vi "Text control 2 v6.8_pump-specific.vi"() -> ()   [LabVIEW 2016]
panel:
  in  "Tab Control":enum32{"Main", "Other parameters"}(tab)
  out "Line running":i32
  out "Total lines":i32
  out "Path":path=path "C:/users/rlp38/09Apr2009LTtesting/test2.txt"
  out "I vs Vg":cluster{"Y data in":dbl[], "X data in":dbl[]}[](graph)
  out "Is max":dbl format="%.2e"
  out "Id max":dbl format="%.2e"
  out "Ig max":dbl format="%.2e"
  out "Imax vs time":cluster{"Y data in":dbl[], "X data in":dbl[]}[](graph)
  out "Imin vs time":cluster{"Y data in":dbl[], "X data in":dbl[]}[](graph)
  out "I vs Vd":cluster{"Y data in":dbl[], "X data in":dbl[]}[](graph)
  in  "Script":string="#-------------------------------------------------------\n# SPM pump cleaning script\n#\n# Version: 0.5\n# Author: Dimitrios Simatos\n# Last updated: 2018-01-05\n#-------------------------------------------------------\n# Description\n#\n# This script is designed to run the cleaning sequence of the SPM OEM pump.\n# This script needs to be run 4 times!\n#-------------------------------------------------------\n# Changes\n#\n# Placed initialization and hard stop commands in the beginning.\n#-------------------------------------------------------\n# Important points\n#\n# Never leave any liquid in the pump to dry after the experiments. If they dry, the residue may block the valve.\n# Always run the cleaning cycle after the experiments.\n# Use clockwise rotation when going up in valve port numbers and vice versa.\n#-------------------------------------------------------\n# Things to do before running the script\n#\n# Set time units to minutes.\n# Set filenames.\n# Replace the tubing, if necessary.\n#-------------------------------------------------------\n# Port connections\n#\n# Port 1: Waste\n# Port 2: Waste\n# Port 3: Various cleaning liquids\n# Port 4: Waste\n# Port 5: Waste\n# Port 6: Waste\n#\n# Between each of the 4 runs, the settings of Port 3 will change, according to the cleaning protocol.\n# The settings for Port 3 are:\n# 1st run: 1% v/v solution of sodium hypochlorite in ultrapure water\n# 2nd run: 0.1% w/v solution of sodium dodecyl sulfate in ultrapure water\n# 3rd run: Ultrapure water\n# 4th run: Waste (in air, not immersed in liquid)\n#-------------------------------------------------------\n# Cleaning protocol for the SPM OEM pump (from the manual)\n#\n# A cleaning procedure should be performed at the end of each day or in between two different experiments.\n# An effective cleaning can be performed in the following manner:\n# • Bleach solution to kill microorganisms\n# 1. Prepare a solution of 1% chlorine bleach and deionized water\n#    NOTE: Prepare a 1% v/v solution of sodium hypochlorite in deionized water\n# 2. Prepare a reservoir and place 1 tubing in the bleach solution and 5 tubings in a waste recipient\n# 3. Pick up the bleach solution through 1 port to entirely fill the syringe\n# 4. Sequentially output the syringe content through the remaining ports and throw it to the waste\n# 5. Repeat operation at least 2 times\n# • Detergent solution to remove debris\n# 1. Prepare a solution of 0.1% detergent and deionized water\n#    NOTE: Prepare a 0.1% w/v solution of sodium dodecyl sulfate in deionized water\n# 2. Move the tubing from the bleach solution reservoir and place it into a reservoir of detergent solution\n# 3. Pick up the detergent solution through 1 port to entirely fill the syringe\n# 4. Sequentially output the detergent solution through the remaining ports into the waste recipient\n# 5. Repeat operation at least 2 times\n# • Rinsing water to prepare the pump for your next experiment\n# 1. Move the tubing from the detergent solution reservoir and place it into a reservoir of deionized water\n# 2. Pick up the rinsing solution through 1 port to entirely fill the syringe\n# 3. Sequentially output the rinse water through the remaining ports into the waste recipient\n# 4. Repeat operation at least 2 times\n# • Replace the tubing, if necessary\n#-------------------------------------------------------\n# Pumping cycles and execution time\n#\n# Execution time for a single cycle: 6 x (1 min + 10 sec) = 7 minutes\n# Total execution time: 4 x 7 = 28 minutes\n# Since the script has to run 4 times, the cleaning lasts for: 4 x 28 = 112 minutes\n# Air must be the last to be pumped through the valve, to remove all liquids.\n# There are 4 pumping cycles. Each one draws a different liquid through port 3 and pumps it sequentially through ports 1,2,4,5,6.\n# During the sequential pumping, each port receives 200 ml of liquid (20% of the total syringe volume = 600 \"plunger units\")\n# The device must be disconnected from the port during the cleaning procedure.\n# All cycles are similar, except cycle 1 has the initialization command uncommented and the first report valve command commented.\n#-------------------------------------------------------\n# Volume of liquid needed\n#\n# Volume of liquid needed per cycle: 1 ml\n# Total volume of liquid needed per script run: 4 x 1 = 4 ml\n# Since the script has to run 4 times, the first 3 with different liquids, I need:\n# 4 ml of 1% v/v solution of sodium hypochlorite in ultrapure water\n# 4 ml of 0.1% w/v solution of sodium dodecyl sulfate in ultrapure water\n# 4 ml of ultrapure water\n#-------------------------------------------------------\n# Parameters\n#\n# Syringe size: 1 ml\n# Step resolution N = 0.01 mm\n# Drawing flow V = 300 pulses/second (6000 ul/min)\n# Pumping flow V = 300 pulses/second (6000 ul/min)\n#-------------------------------------------------------\n# Pump initialization\npump /1T #hard stop pump\npump /1ZR #initialize pump\n#-------------------------------------------------------\n# Cycle 1\n# Fill the syringe\npump /1Q #query pump\npump /1? #report absolute plunger position\n#pump /1?6 #report valve position\nwait-min 1 #wait 1 minute\npump /1N0R #set step resolution: 0.01 mm\npump /1Q #query pump\npump /1? #report absolute plunger position (the plunger should be at 0)\npump /1?6 #report valve position\nwait 1000 #wait 1 second\npump /1V300R #choose speed: 300 steps/s (6000 ul/min)\npump /1Q #query pump\nwait 1000 #wait 1 second\npump /1I3R #go to port 3, clockwise rotation\npump /1Q #query pump\npump /1?6 #report valve position\nwait 1000 #wait 1 second\npump /1A3000R #go to absolute position 3000 (= draw 1 ml)\nwait 30000 #wait 30 seconds\npump /1Q #query pump\npump /1? #report absolute plunger position (the plunger should have finished moving)\n#pump /1?6 #report valve position\n# The sequential pumping begins\n# Port 1\npump /1O1R #switch to port 1, counterclockwise rotation\npump /1Q #query pump\npump /1?6 #report valve position\npump /1A2400R #go to absolute position 2400 (= pump 200 ul)\npump /1Q #query pump\npump /1? #report absolute plunger position (the plunger should be moving to 0)\nwait-min 1 #wait 1 minute\npump /1? #report absolute plunger position (the plunger should have finished moving)\n# Port 2\npump /1I2R #switch to port 2, clockwise rotation\npump /1Q #query pump\npump /1?6 #report valve position\npump /1A1800R #go to absolute position 1800 (= pump 200 ul)\npump /1Q #query pump\npump /1? #report absolute plunger position (the plunger should be moving to 0)\nwait-min 1 #wait 1 minute\npump /1? #report absolute plunger position (the plunger should have finished moving)\n# Port 4\npump /1I4R #switch to port 4, clockwise rotation\npump /1Q #query pump\npump /1?6 #report valve position\npump /1A1200R #go to absolute position 1200 (= pump 200 ul)\npump /1Q #query pump\npump /1? #report absolute plunger position (the plunger should be moving to 0)\nwait-min 1 #wait 1 minute\npump /1? #report absolute plunger position (the plunger should have finished moving)\n# Port 5\npump /1I5R #switch to port 5, clockwise rotation\npump /1Q #query pump\npump /1?6 #report valve position\npump /1A600R #go to absolute position 600 (= pump 200 ul)\npump /1Q #query pump\npump /1? #report absolute plunger position (the plunger should be moving to 0)\nwait-min 1 #wait 1 minute\npump /1? #report absolute plunger position (the plunger should have finished moving)\n# Port 6\npump /1I6R #switch to port 6, clockwise rotation\npump /1Q #query pump\npump /1?6 #report valve position\npump /1A0R #go to absolute position 0 (= pump 200 ul)\npump /1Q #query pump\npump /1? #report absolute plunger position (the plunger should be moving to 0)\nwait-min 1 #wait 1 minute\npump /1? #report absolute plunger position (the plunger should have finished moving)\n#-------------------------------------------------------\n# Cycle 2\n# Fill the syringe\n#pump /1ZR #initialize pump\npump /1Q #query pump\npump /1? #report absolute plunger position\npump /1?6 #report valve position\nwait-min 1 #wait 1 minute\npump /1N0R #set step resolution: 0.01 mm\npump /1Q #query pump\npump /1? #report absolute plunger position (the plunger should be at 0)\npump /1?6 #report valve position\nwait 1000 #wait 1 second\npump /1V300R #choose speed: 300 steps/s (6000 ul/min)\npump /1Q #query pump\nwait 1000 #wait 1 second\npump /1O3R #go to port 3, counterclockwise rotation\npump /1Q #query pump\npump /1?6 #report valve position\nwait 1000 #wait 1 second\npump /1A3000R #go to absolute position 3000 (= draw 1 ml)\nwait 30000 #wait 30 seconds\npump /1Q #query pump\npump /1? #report absolute plunger position (the plunger should have finished moving)\n#pump /1?6 #report valve position\n# The sequential pumping begins\n# Port 1\npump /1O1R #switch to port 1, counterclockwise rotation\npump /1Q #query pump\npump /1?6 #report valve position\npump /1A2400R #go to absolute position 2400 (= pump 200 ul)\npump /1Q #query pump\npump /1? #report absolute plunger position (the plunger should be moving to 0)\nwait-min 1 #wait 1 minute\npump /1? #report absolute plunger position (the plunger should have finished moving)\n# Port 2\npump /1I2R #switch to port 2, clockwise rotation\npump /1Q #query pump\npump /1?6 #report valve position\npump /1A1800R #go to absolute position 1800 (= pump 200 ul)\npump /1Q #query pump\npump /1? #report absolute plunger position (the plunger should be moving to 0)\nwait-min 1 #wait 1 minute\npump /1? #report absolute plunger position (the plunger should have finished moving)\n# Port 4\npump /1I4R #switch to port 4, clockwise rotation\npump /1Q #query pump\npump /1?6 #report valve position\npump /1A1200R #go to absolute position 1200 (= pump 200 ul)\npump /1Q #query pump\npump /1? #report absolute plunger position (the plunger should be moving to 0)\nwait-min 1 #wait 1 minute\npump /1? #report absolute plunger position (the plunger should have finished moving)\n# Port 5\npump /1I5R #switch to port 5, clockwise rotation\npump /1Q #query pump\npump /1?6 #report valve position\npump /1A600R #go to absolute position 600 (= pump 200 ul)\npump /1Q #query pump\npump /1? #report absolute plunger position (the plunger should be moving to 0)\nwait-min 1 #wait 1 minute\npump /1? #report absolute plunger position (the plunger should have finished moving)\n# Port 6\npump /1I6R #switch to port 6, clockwise rotation\npump /1Q #query pump\npump /1?6 #report valve position\npump /1A0R #go to absolute position 0 (= pump 200 ul)\npump /1Q #query pump\npump /1? #report absolute plunger position (the plunger should be moving to 0)\nwait-min 1 #wait 1 minute\npump /1? #report absolute plunger position (the plunger should have finished moving)\n#-------------------------------------------------------\n# Cycle 3\n# Fill the syringe\n#pump /1ZR #initialize pump\npump /1Q #query pump\npump /1? #report absolute plunger position\npump /1?6 #report valve position\nwait-min 1 #wait 1 minute\npump /1N0R #set step resolution: 0.01 mm\npump /1Q #query pump\npump /1? #report absolute plunger position (the plunger should be at 0)\npump /1?6 #report valve position\nwait 1000 #wait 1 second\npump /1V300R #choose speed: 300 steps/s (6000 ul/min)\npump /1Q #query pump\nwait 1000 #wait 1 second\npump /1O3R #go to port 3, counterclockwise rotation\npump /1Q #query pump\npump /1?6 #report valve position\nwait 1000 #wait 1 second\npump /1A3000R #go to absolute position 3000 (= draw 1 ml)\nwait 30000 #wait 30 seconds\npump /1Q #query pump\npump /1? #report absolute plunger position (the plunger should have finished moving)\n#pump /1?6 #report valve position\n# The sequential pumping begins\n# Port 1\npump /1O1R #switch to port 1, counterclockwise rotation\npump /1Q #query pump\npump /1?6 #report valve position\npump /1A2400R #go to absolute position 2400 (= pump 200 ul)\npump /1Q #query pump\npump /1? #report absolute plunger position (the plunger should be moving to 0)\nwait-min 1 #wait 1 minute\npump /1? #report absolute plunger position (the plunger should have finished moving)\n# Port 2\npump /1I2R #switch to port 2, clockwise rotation\npump /1Q #query pump\npump /1?6 #report valve position\npump /1A1800R #go to absolute position 1800 (= pump 200 ul)\npump /1Q #query pump\npump /1? #report absolute plunger position (the plunger should be moving to 0)\nwait-min 1 #wait 1 minute\npump /1? #report absolute plunger position (the plunger should have finished moving)\n# Port 4\npump /1I4R #switch to port 4, clockwise rotation\npump /1Q #query pump\npump /1?6 #report valve position\npump /1A1200R #go to absolute position 1200 (= pump 200 ul)\npump /1Q #query pump\npump /1? #report absolute plunger position (the plunger should be moving to 0)\nwait-min 1 #wait 1 minute\npump /1? #report absolute plunger position (the plunger should have finished moving)\n# Port 5\npump /1I5R #switch to port 5, clockwise rotation\npump /1Q #query pump\npump /1?6 #report valve position\npump /1A600R #go to absolute position 600 (= pump 200 ul)\npump /1Q #query pump\npump /1? #report absolute plunger position (the plunger should be moving to 0)\nwait-min 1 #wait 1 minute\npump /1? #report absolute plunger position (the plunger should have finished moving)\n# Port 6\npump /1I6R #switch to port 6, clockwise rotation\npump /1Q #query pump\npump /1?6 #report valve position\npump /1A0R #go to absolute position 0 (= pump 200 ul)\npump /1Q #query pump\npump /1? #report absolute plunger position (the plunger should be moving to 0)\nwait-min 1 #wait 1 minute\npump /1? #report absolute plunger position (the plunger should have finished moving)\n#-------------------------------------------------------\n# Cycle 4\n# Fill the syringe\n#pump /1ZR #initialize pump\npump /1Q #query pump\npump /1? #report absolute plunger position\npump /1?6 #report valve position\nwait-min 1 #wait 1 minute\npump /1N0R #set step resolution: 0.01 mm\npump /1Q #query pump\npump /1? #report absolute plunger position (the plunger should be at 0)\npump /1?6 #report valve position\nwait 1000 #wait 1 second\npump /1V300R #choose speed: 300 steps/s (6000 ul/min)\npump /1Q #query pump\nwait 1000 #wait 1 second\npump /1O3R #go to port 3, counterclockwise rotation\npump /1Q #query pump\npump /1?6 #report valve position\nwait 1000 #wait 1 second\npump /1A3000R #go to absolute position 3000 (= draw 1 ml)\nwait 30000 #wait 30 seconds\npump /1Q #query pump\npump /1? #report absolute plunger position (the plunger should have finished moving)\n#pump /1?6 #report valve position\n# The sequential pumping begins\n# Port 1\npump /1O1R #switch to port 1, counterclockwise rotation\npump /1Q #query pump\npump /1?6 #report valve position\npump /1A2400R #go to absolute position 2400 (= pump 200 ul)\npump /1Q #query pump\npump /1? #report absolute plunger position (the plunger should be moving to 0)\nwait-min 1 #wait 1 minute\npump /1? #report absolute plunger position (the plunger should have finished moving)\n# Port 2\npump /1I2R #switch to port 2, clockwise rotation\npump /1Q #query pump\npump /1?6 #report valve position\npump /1A1800R #go to absolute position 1800 (= pump 200 ul)\npump /1Q #query pump\npump /1? #report absolute plunger position (the plunger should be moving to 0)\nwait-min 1 #wait 1 minute\npump /1? #report absolute plunger position (the plunger should have finished moving)\n# Port 4\npump /1I4R #switch to port 4, clockwise rotation\npump /1Q #query pump\npump /1?6 #report valve position\npump /1A1200R #go to absolute position 1200 (= pump 200 ul)\npump /1Q #query pump\npump /1? #report absolute plunger position (the plunger should be moving to 0)\nwait-min 1 #wait 1 minute\npump /1? #report absolute plunger position (the plunger should have finished moving)\n# Port 5\npump /1I5R #switch to port 5, clockwise rotation\npump /1Q #query pump\npump /1?6 #report valve position\npump /1A600R #go to absolute position 600 (= pump 200 ul)\npump /1Q #query pump\npump /1? #report absolute plunger position (the plunger should be moving to 0)\nwait-min 1 #wait 1 minute\npump /1? #report absolute plunger position (the plunger should have finished moving)\n# Port 6\npump /1I6R #switch to port 6, clockwise rotation\npump /1Q #query pump\npump /1?6 #report valve position\npump /1A0R #go to absolute position 0 (= pump 200 ul)\npump /1Q #query pump\npump /1? #report absolute plunger position (the plunger should be moving to 0)\nwait-min 1 #wait 1 minute\npump /1? #report absolute plunger position (the plunger should have finished moving)\n#-------------------------------------------------------"
  out "Command running:":string
  out "Serial port data":string
  out "Elapsed Time":dbl caption="Elapsed Time (s)"
  in  "Time Units":u16(ring)=1 items=["Seconds", "Minutes", "Hours"]
  in  "Time Offset":dbl caption="Set Start Time (s)"
  in  "Reset":bool
  in  "Auto Reset":bool
  in  "integration time":u32(slide) max=2 step=1 scale=0.0..2.0
  in  "Interrupt scan":bool
  out "Absolute plunger position vs time":cluster{"Y data in":dbl[], "X data in":dbl[]}[](graph)
  out "Valve position vs time":cluster{"Y data in":dbl[], "X data in":dbl[]}[](graph)
  out "Is on":dbl format="%.2e"
  out "Id on":dbl format="%.2e"
  out "Ig on":dbl format="%.2e"
  out "Ion vs time":cluster{"Y data in":dbl[], "X data in":dbl[]}[](graph)
  out "Ioff vs time":cluster{"Y data in":dbl[], "X data in":dbl[]}[](graph)
  out "Ig min":dbl format="%.2e"
  out "Id min":dbl format="%.2e"
  out "Is min":dbl format="%.2e"
  out "Is off":dbl format="%.2e"
  out "Id off":dbl format="%.2e"
  out "Ig off":dbl format="%.2e"
  in  "Integration time (long)":dbl=0.32 min=0.04 max=2.0 step=0.02 format="%.2f"
  in  "Integration time (short)":dbl=0.0019 min=8e-05 max=0.0019 step=8e-05 format="%^.0e"
  in  "Gate: Compliance":dbl=0.001 format="%.8f"
  in  "Drain: Compliance":dbl=0.001 format="%.8f"
  in  "Hard stop pump":bool
  in  "Halt pump":bool
  in  "Interrupt program":bool
  in  "Suffix (script)":string="step_1_up-H2O_initial_script.txt"
  in  "Filename (variable part)":string="step_1_up-H2O_initial_"
  in  "Plot output curve extrema vs time":bool
  in  "Plot transfer curve extrema vs time":bool=TRUE
  in  "Plot sample extrema vs time":bool
  out "I vs time (Bias Stress)":cluster{"Y data in":dbl[], "X data in":dbl[]}[](graph)
  in  "Sample I - Probe 4 (Disabled)":u32(ring)=3 items=["SMU1  ", "SMU2  ", "SMU3  ", "SMU4  ", "SMU5  ", "SMU6  "]
  in  "Sample I - Source/Common":u32(ring) items=["SMU1  ", "SMU2  ", "SMU3  ", "SMU4  ", "SMU5  ", "SMU6  "]
  in  "Sample I - Probe 3 (Disabled)":u32(ring)=2 items=["SMU1  ", "SMU2  ", "SMU3  ", "SMU4  ", "SMU5  ", "SMU6  "]
  in  "Sample I - Drain/Gate":u32(ring)=1 items=["SMU1  ", "SMU2  ", "SMU3  ", "SMU4  ", "SMU5  ", "SMU6  "]
  in  "Sample - Probe 4":u32(ring)=3 items=["SMU1  ", "SMU2  ", "SMU3  ", "SMU4  ", "SMU5  ", "SMU6  "]
  in  "Sample - Source/Common":u32(ring) items=["SMU1  ", "SMU2  ", "SMU3  ", "SMU4  ", "SMU5  ", "SMU6  "]
  in  "Sample - Gate":u32(ring)=2 items=["SMU1  ", "SMU2  ", "SMU3  ", "SMU4  ", "SMU5  ", "SMU6  "]
  in  "Sample - Drain":u32(ring)=1 items=["SMU1  ", "SMU2  ", "SMU3  ", "SMU4  ", "SMU5  ", "SMU6  "]
  in  "VSU2 Stress - Source/Common":u32(ring) items=["SMU1  ", "SMU2  ", "SMU3  ", "SMU4  ", "SMU5  ", "SMU6  "]
  in  "Stress I - Source/Common":u32(ring) items=["SMU1  ", "SMU2  ", "SMU3  ", "SMU4  ", "SMU5  ", "SMU6  "]
  in  "Stress I - Drain/Gate":u32(ring)=1 items=["SMU1  ", "SMU2  ", "SMU3  ", "SMU4  ", "SMU5  ", "SMU6  "]
  in  "Stress V - Source/Common":u32(ring) items=["SMU1  ", "SMU2  ", "SMU3  ", "SMU4  ", "SMU5  ", "SMU6  "]
  in  "Stress V - Gate":u32(ring)=2 items=["SMU1  ", "SMU2  ", "SMU3  ", "SMU4  ", "SMU5  ", "SMU6  "]
  in  "Stress V - Drain":u32(ring)=1 items=["SMU1  ", "SMU2  ", "SMU3  ", "SMU4  ", "SMU5  ", "SMU6  "]
  in  "FPP - Source":u32(ring) items=["VSU1  ", "VSU2  "]
  in  "FPP - Probe 2":u32(ring)=3 items=["SMU1  ", "SMU2  ", "SMU3  ", "SMU4  ", "SMU5  ", "SMU6  "]
  in  "FPP - Probe 1":u32(ring) items=["SMU1  ", "SMU2  ", "SMU3  ", "SMU4  ", "SMU5  ", "SMU6  "]
  in  "FPP - Gate":u32(ring)=2 items=["SMU1  ", "SMU2  ", "SMU3  ", "SMU4  ", "SMU5  ", "SMU6  "]
  in  "FPP - Drain":u32(ring)=1 items=["SMU1  ", "SMU2  ", "SMU3  ", "SMU4  ", "SMU5  ", "SMU6  "]
  in  "Pulsed Stress V - Vextra":u32(ring)=1 items=["VSU1  ", "VSU2  "]
  in  "Pulsed Stress V - Probe 4":u32(ring)=3 items=["SMU1  ", "SMU2  ", "SMU3  ", "SMU4  ", "SMU5  ", "SMU6  "]
  in  "Pulsed Stress V - Source/Common":u32(ring) items=["SMU1  ", "SMU2  ", "SMU3  ", "SMU4  ", "SMU5  ", "SMU6  "]
  in  "Pulsed Stress V - Gate":u32(ring)=2 items=["SMU1  ", "SMU2  ", "SMU3  ", "SMU4  ", "SMU5  ", "SMU6  "]
  in  "Pulsed Stress V - Drain":u32(ring)=1 items=["SMU1  ", "SMU2  ", "SMU3  ", "SMU4  ", "SMU5  ", "SMU6  "]
  in  "Transfer/Output - Probe 4":u32(ring)=3 items=["SMU1  ", "SMU2  ", "SMU3  ", "SMU4  ", "SMU5  ", "SMU6  "]
  in  "Transfer/Output - Source/Common":u32(ring) items=["SMU1  ", "SMU2  ", "SMU3  ", "SMU4  ", "SMU5  ", "SMU6  "]
  in  "Transfer/Output - Gate":u32(ring)=2 items=["SMU1  ", "SMU2  ", "SMU3  ", "SMU4  ", "SMU5  ", "SMU6  "]
  in  "Transfer/Output - Drain":u32(ring)=1 items=["SMU1  ", "SMU2  ", "SMU3  ", "SMU4  ", "SMU5  ", "SMU6  "]
  in  "Gate Range\nmode":u16(ring) items=["Auto", "Limited", "Fixed"]
  in  "Gate Range":u8(slide)=3 max=11 scale=0.0..11.0
  in  "Source/Drain\nRange mode":u16(ring) items=["Auto", "Limited", "Fixed"]
  in  "Source/Drain Range":u8(slide)=3 max=11 scale=0.0..11.0
  in  "Panel Controls":T1={"Emergency Stop"=refnum, "TransGraph Max"=1e-05, "Text/Graph (text=false)"=TRUE} {"TransGraph Max" format="%.2e"}
  in  "Panel Controls 2":T2={"Emergency Stop"=refnum, "TransGraph Max"=1e-05, "Text/Graph (text=false)"=TRUE, "TransGraph Min"=1e-11} {"TransGraph Min" format="%.2e"; "TransGraph Max" format="%.2e"}
  in  "Probe 4":cluster{"on/off":bool, "Voltage":dbl} {"Voltage" min=-100.0 max=100.0 format="%.2f"}
  in  "Full Reset":bool
  in  "Standby":T3
  out "error out":errorcluster
  in  "Delay before read (ms)":u32=1000
  in  "byte count":u32=64
  in  "Serial End Mode for Reads":u16(ring)=2 items=["None", "LastBit", "TermChar"]
  in  "Timeout (ms)":u32=10000
  in  "Enable Termination\nChar (T)":bool=TRUE
  in  "Termination char\n(0xA = '\\n' = LF)\n(0xD = '\\r' = CR)":u8=13 format="%.0x"
  in  "flow control":u16(ring) items=["None"=0, "XON/XOFF"=1, "RTS/CTS"=2, "DTR/DSR"=4]
  in  "stop bits":u16(ring)=10 items=["1.0"=10, "1.5"=15, "2.0"=20]
  in  "parity":u16(ring) items=["None", "Odd", "Even", "Mark", "Space"]
  in  "data bits":u16=8 min=5 max=8 step=1
  in  "VISA resource name":refnum<visa-resource-name>="COM6"
  in  "baud rate":u32=9600
  out "Timings Indicator":T4 {"integration time" scale=0.0..2.0}
  in  "Timings (overwritten by the Front Panel)":T5={"integration time"=0, "Short/Long integration time"=0.00064, "hold time (sec)"=0.0, "delay time (sec)"=0.0, "Step Time (0 disables)"=0.0, "sweep method"=0, "Pulse period"=0.005, "Base voltage"=0.0, "Pulse width"=0.0005} {"Pulse width" min=0.0005 max=0.1 step=0.0001 format="%.4f"; "Base voltage" format="%^.4e"; "Pulse period" min=0.005 max=1.0 step=0.0001 format="%.4f"; "sweep method" items=["Continuous", "Pulsed"]; "Step Time (0 disables)" format="%.2f"; "delay time (sec)" format="%.4f"; "hold time (sec)" format="%.4f"; "Short/Long integration time" format="%^.0e"; "integration time" scale=0.0..2.0}
  out "Probe 4 Indicator":cluster{"on/off":bool, "Voltage":dbl} {"Voltage" min=-100.0 max=100.0 format="%.2f"}
  in  "VISA resource name in":refnum<visa-resource-name>="GPIB0::14::INSTR"
  in  "Gate":T6={"Gate Start"=0.0, "Gate Stop"=2.0, "Gate Step (linear only)"=1.0, "Gate Compliance"=0.0001, "Gate PComp"=0.0, "Range mode"=0, "Range"=6} {"Range" max=11 scale=0.0..11.0; "Range mode" items=["Auto", "Limited", "Fixed"]; "Gate PComp" format="%^.2e"; "Gate Compliance" format="%^.2e"; "Gate Step (linear only)" format="%^.4e"; "Gate Stop" format="%^.4e"; "Gate Start" format="%^.4e"}
  in  "Drain 2":T7={"Drain Start"=0.0, "Drain Stop"=2.0, "Drain Compliance"=0.0001, "Drain Step"=1.0, "Drain PComp"=0.0, "Range mode"=0, "Range"=6} {"Range" max=11 scale=0.0..11.0; "Range mode" items=["Auto", "Limited", "Fixed"]; "Drain PComp" format="%^.2e"; "Drain Step" format="%^.4e"; "Drain Compliance" format="%^.2e"; "Drain Stop" format="%^.4e"; "Drain Start" format="%^.4e"}
  # "Syntax:\nitime [s|m|l] time(sec): [s|m|l] determines the integration time setting (small|medium|long) and time sets the value.\nNOTE: The value of the integration time has to be within the range allowed by its category (s|m|l), otherwise, the closest value will be used. (e.g. if the category is set to short but the time value is very long, the actual value used will be the maximum short integration time.\nIntegration times:\n    Short: Default: 640 us. Range: 8E-5 - 1.92E-3 seconds.\n    Medium: Fixed at 1 NPL cycle (0.02 seconds).\n    Long: Default: 16 NPL cycles (0.32 seconds). Range: 2-100 NPL cycles (0.04 seconds - 2 seconds).\ngaterangemode [a|l|f]\ndrainrangemode [a|l|f]\npulsed [on|off] PulsePeriod(sec) PulseBaseVoltage PulseONWidth(sec)\nstandby [on l off]\nwait NumMilliseconds\nwait-min NumMinutes\n# texthere = comment\nProbe4 [ON|OFF] Voltage\ntransfer [s|d] VgStart VgStop VgStep VdStart VdStop VdStep\noutput [s|d] VgStart VgStop VgStep VdStart VdStop VdStep\nsample Vg Vd NumSamples Time(s) SampleInterval(s)\nsamplei Idg NumSamples Time(s) SampleInterval(s) VDGcompliance\n100 samples is approximately 13 seconds with medium integration\n# If in doubt use SampleInterval(s) = 0.004\n    NOTE: When doing bias stress measurements, set the Time Units to \"Seconds\", as the \"sample\" command has been configured to give the output to seconds.\nstressV VG VD IGcompliance IDcompliance Duration(sec)\nstressI IDG VDGcompliance Duration(sec)\nvsu2pulse Bias Duration(s)\npulsedstressV [s|d] VEstop VgON VgOFF Period(s) PulseONwidth(s) Vd\nsample-fpp Vg Vd NumSamples Time\nresample-fpp Vg Vd\ntransfer-fpp [s|d] VgStart VgStop VgStep VdStart VdStop VdStep\noutput-fpp [s|d] VgStart VgStop VgStep VdStart VdStop VdStep\nserial SerialPortCommand\npump SerialPortCommand for the SPM pump\n\nSPM Pump Syntax (<x>: pump number, use 1 if only one pump):\nif the command syntax contains [R], then append the letter R to the command\n/<x>Q: query (a query command should follow each command)\n/<x>Z[R] or /<x>Y[R]: initialize pump\n/<x>N<n>[R] (<n>=0,1): <0> (<1>) microstep 0.01 mm (0.00125 mm) resolution\n/<x>I<n> (<n>=0-6): turn to port number n (clockwise)\n/<x>O<n> (<n>=0-6): turn to port number n (counterclockwise)\n/<x>X: Re-execute last command string\n/<x>G<n>[R] (<n>=0-60000): repeat command sequence (default: 0, 0=loop forever)\n/<x>g: Mark the start of a repeat sequence (max = 10)\n/<x>M<n>[R] (<n>=0-86400000): delay command execution by n milliseconds\n/<x>H: Halt; Pause the sequence after finishing the current move\n/<x>T: Hardstop; Interrupt the current move and suppress it from the sequence\n/<x>A<n>[R] (<n>=0-3000 with N=0, 0-24000 with N=1): absolute position\n/<x>P<n>[R] (<n>=0-3000 with N=0, 0-24000 with N=1): relative pickup\n/<x>D<n>[R] (<n>=0-3000 with N=0, 0-24000 with N=1): relative dispense\n/<x>V<n>[R] (<n>=1-1600 default: 150): set peak speed (pulses/sec)\nNOTE: The lowest speed limit is 1 pulse/sec, not 5, as the manual states.\n/<x>S<n>[R] (<n>=10-40 default: 22): set speed (NOT in pulses/sec, look in manual)\nNOTE: When controlled with absolute position, one does not need to pay special attention to the syringe that is mounted on the pump.\nWithdraw from lower stage (ports 3, 5), dispense from higher stage (ports 2, 4, 6).\nConnect Port 1 to waste."
  # "Time"
  # "1\n2\n3\n4\n5\n6\n7\n8\n9\n10\n11\n12\n13\n14\n15\n16\n17\n18\n19\n20"
  # "Serial port settings"
  # "SMUs"
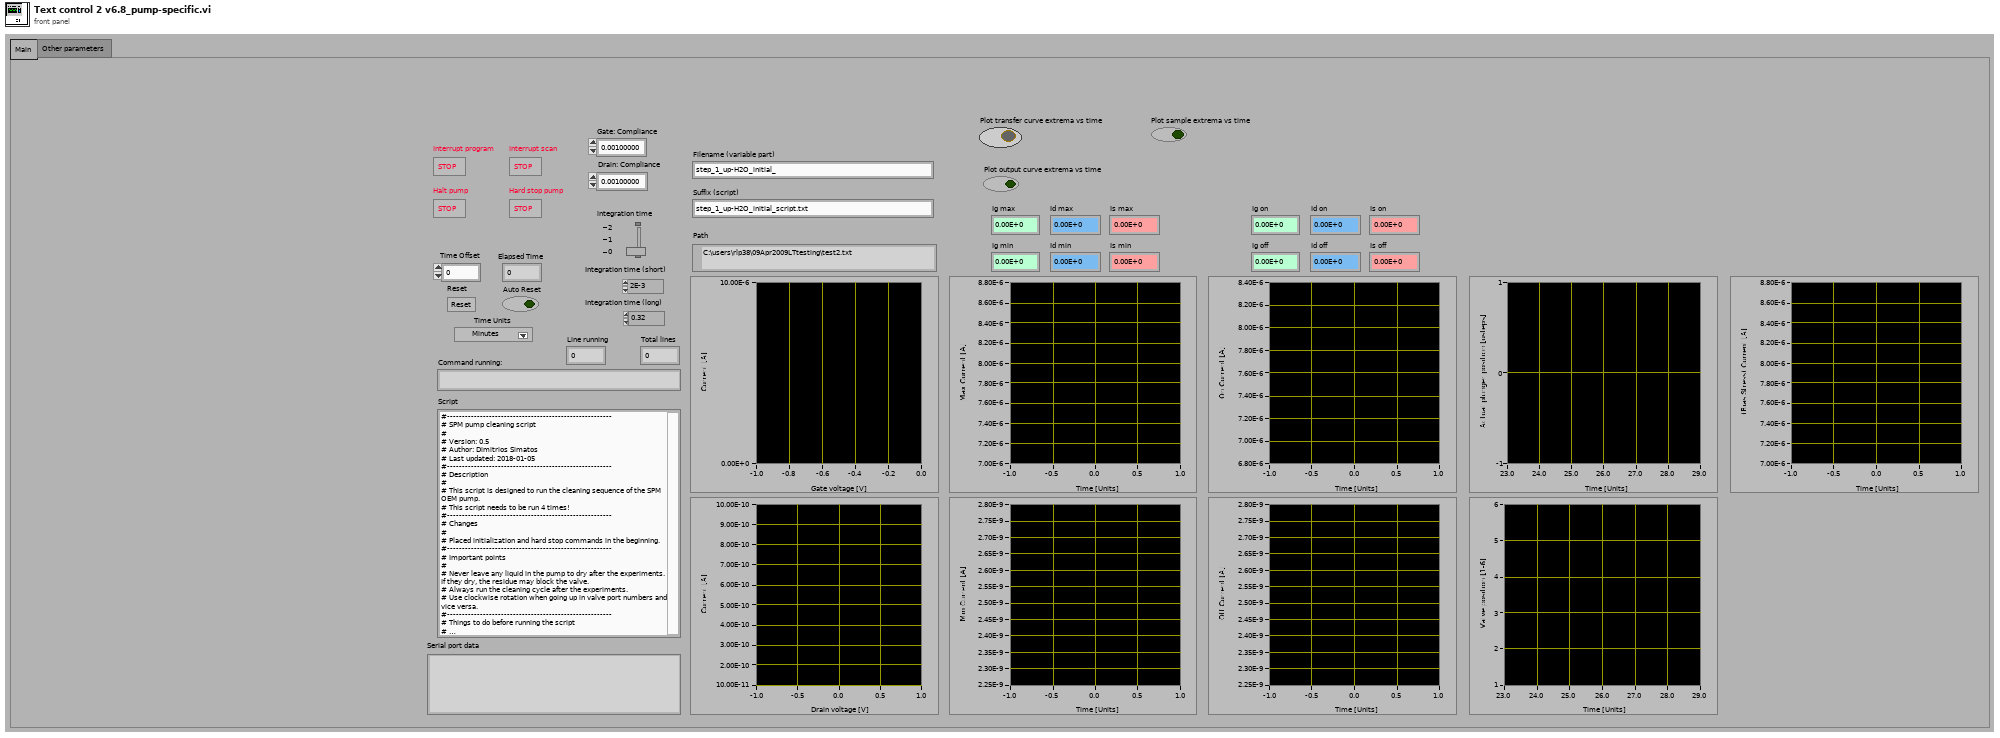
[diagram p1: front panel]
types:
  T1 = cluster{"Emergency Stop":refnum<vi>, "TransGraph Max":dbl, "Text/Graph (text=false)":bool}
  T2 = cluster{"Emergency Stop":refnum<vi>, "TransGraph Max":dbl, "Text/Graph (text=false)":bool, "TransGraph Min":dbl}
  T3 = cluster{"Gate Standby":bool, "Drain Standby":bool}
  T4 = cluster{"Short/Long integration time":dbl, "hold time (sec)":dbl, "delay time (sec)":dbl, "Step Time (0 disables)":dbl, "sweep method":u16, "Pulse period":dbl, "Base voltage":dbl, "Pulse width":dbl, "integration time":u32}
  T5 = cluster{"integration time":u32, "Short/Long integration time":dbl, "hold time (sec)":dbl, "delay time (sec)":dbl, "Step Time (0 disables)":dbl, "sweep method":u16, "Pulse period":dbl, "Base voltage":dbl, "Pulse width":dbl}
  T6 = cluster{"Gate Start":dbl, "Gate Stop":dbl, "Gate Step (linear only)":dbl, "Gate Compliance":dbl, "Gate PComp":dbl, "Range mode":u16, "Range":u8}
  T7 = cluster{"Drain Start":dbl, "Drain Stop":dbl, "Drain Compliance":dbl, "Drain Step":dbl, "Drain PComp":dbl, "Range mode":u16, "Range":u8}
  T8 = enum16{"open", "replace", "create", "open or create", "replace or create", "replace or create with confirmation"}
  T9 = cluster{"V2 Start":dbl, "V2 Step":dbl, "Number of points":i32}
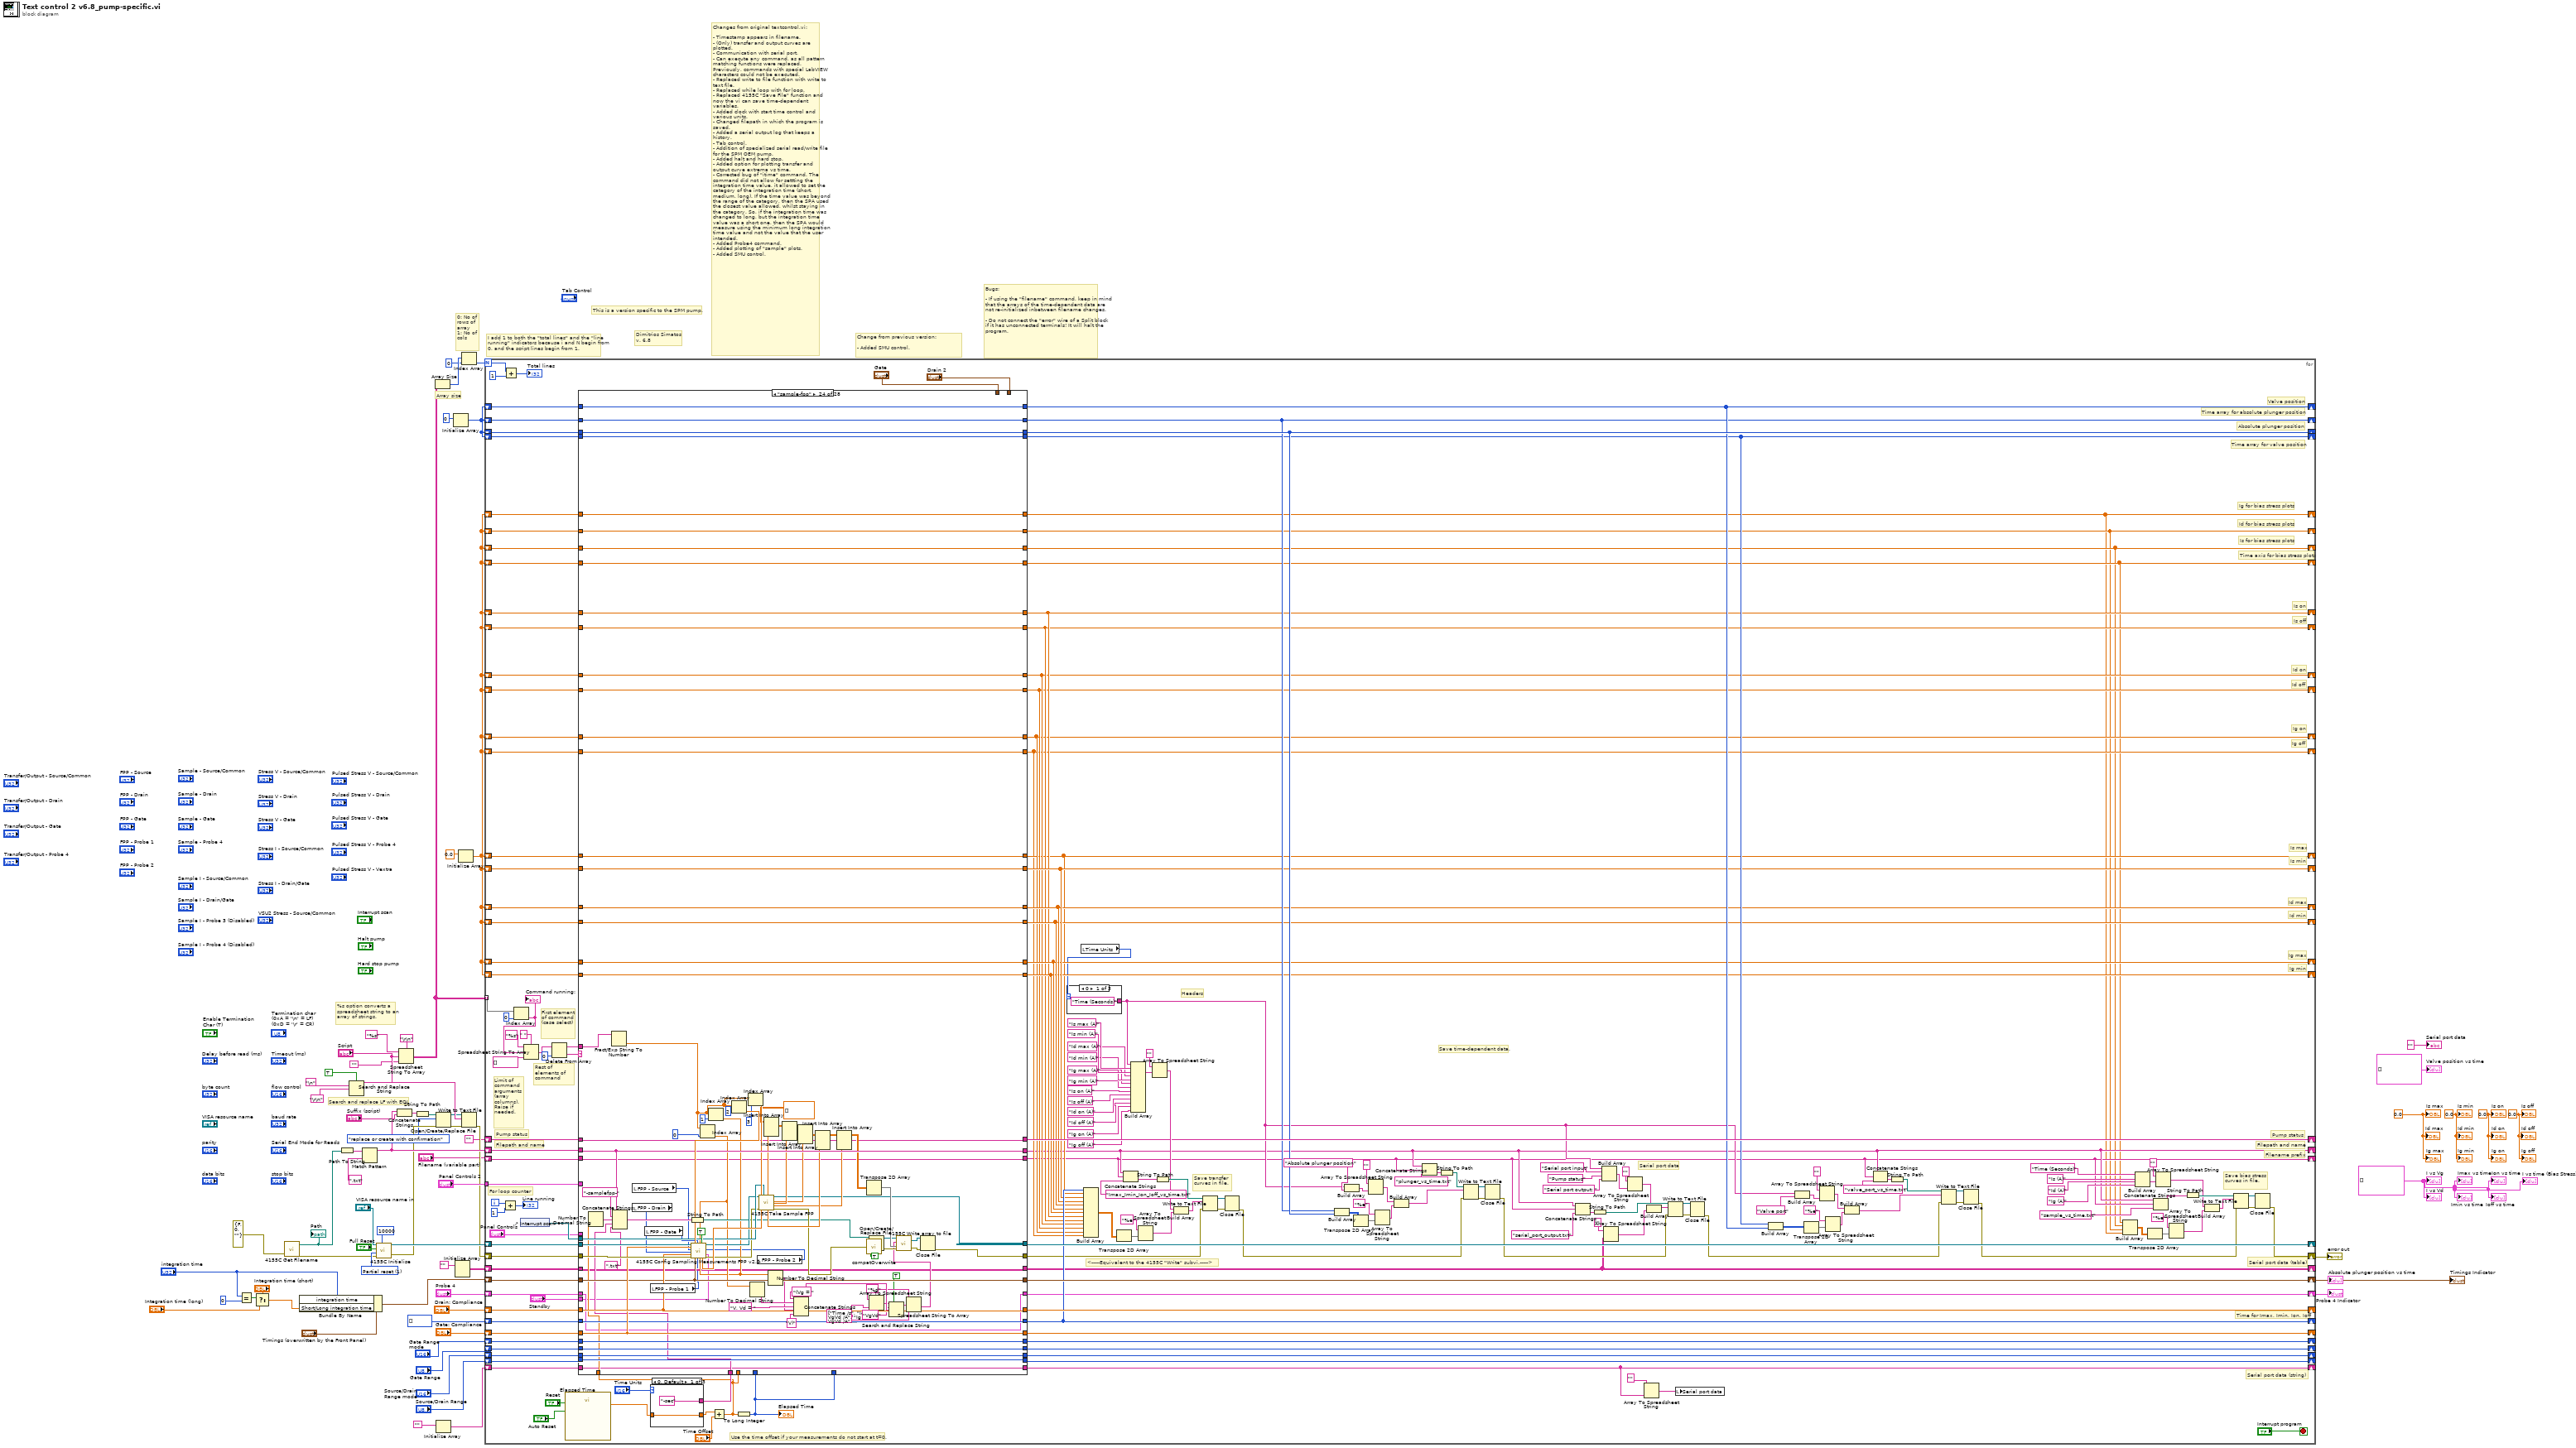
[diagram p0: block diagram]
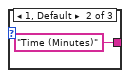
[diagram p2: hidden frame]
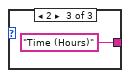
[diagram p3: hidden frame]
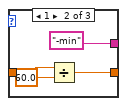
[diagram p4: hidden frame]
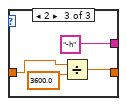
[diagram p5: hidden frame]
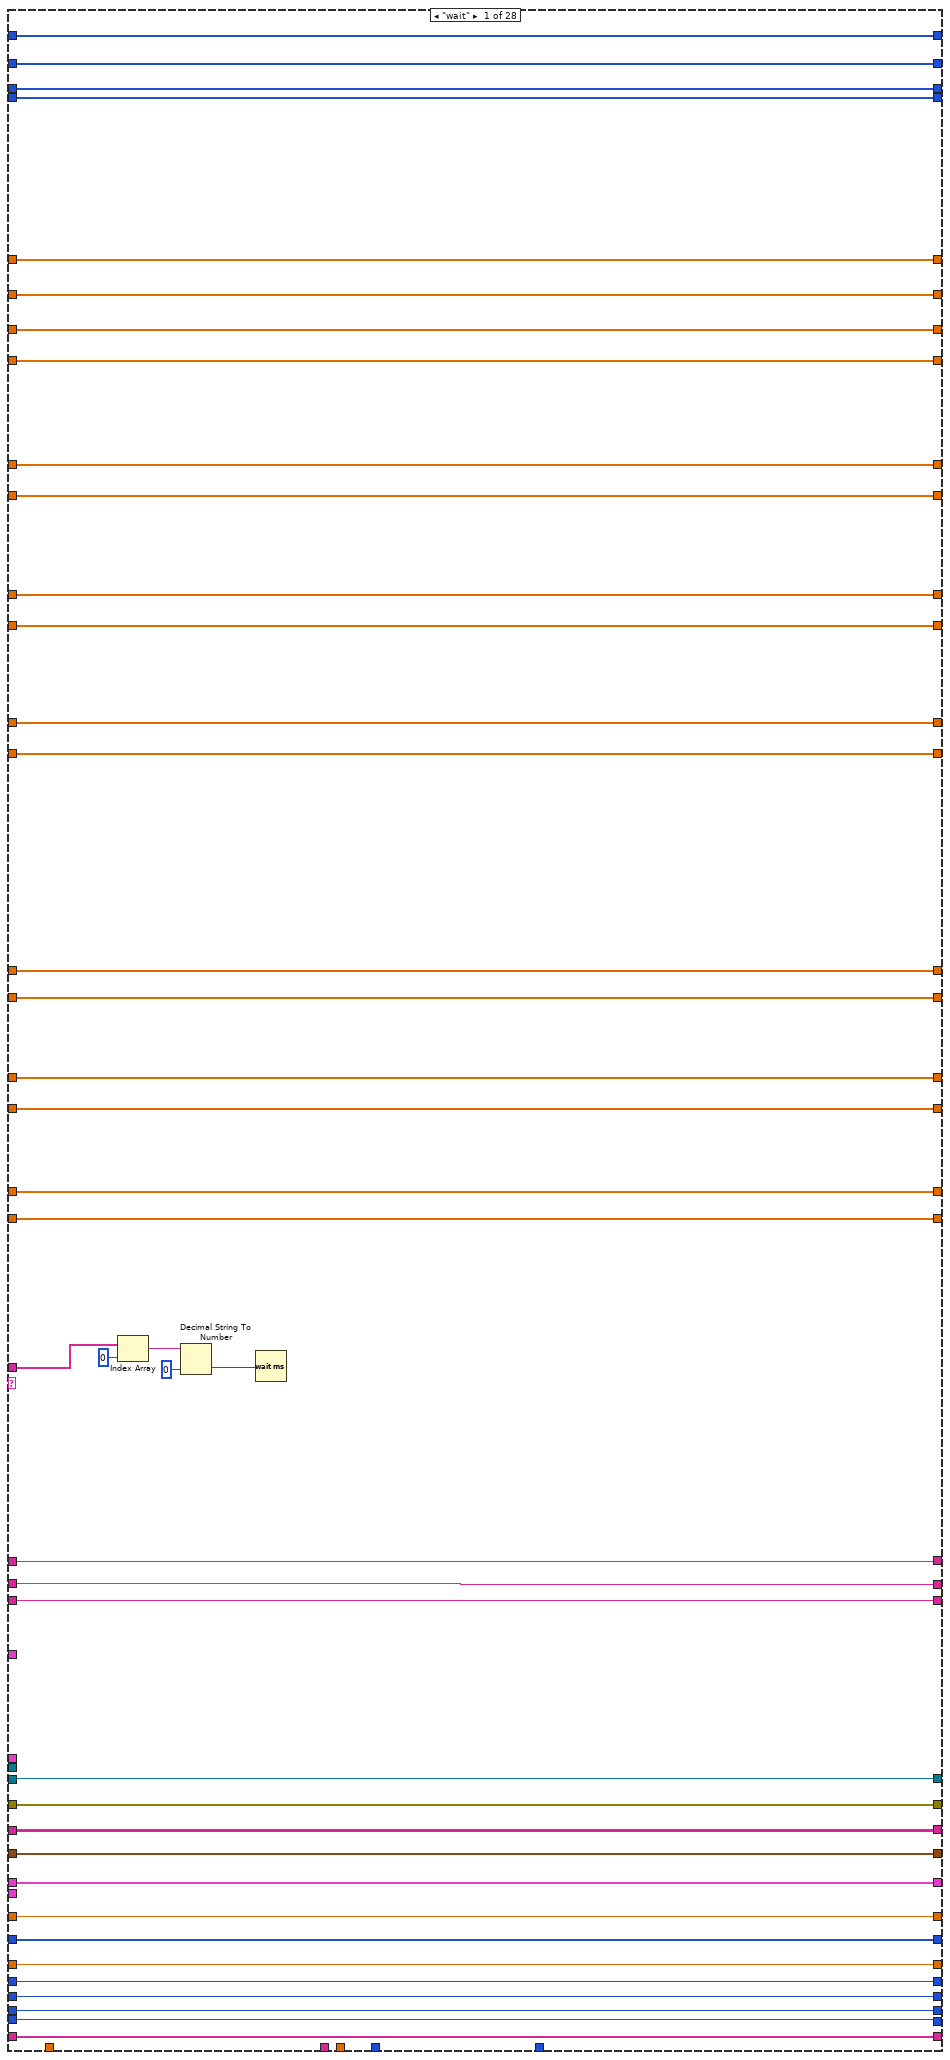
[diagram p6: hidden frame]
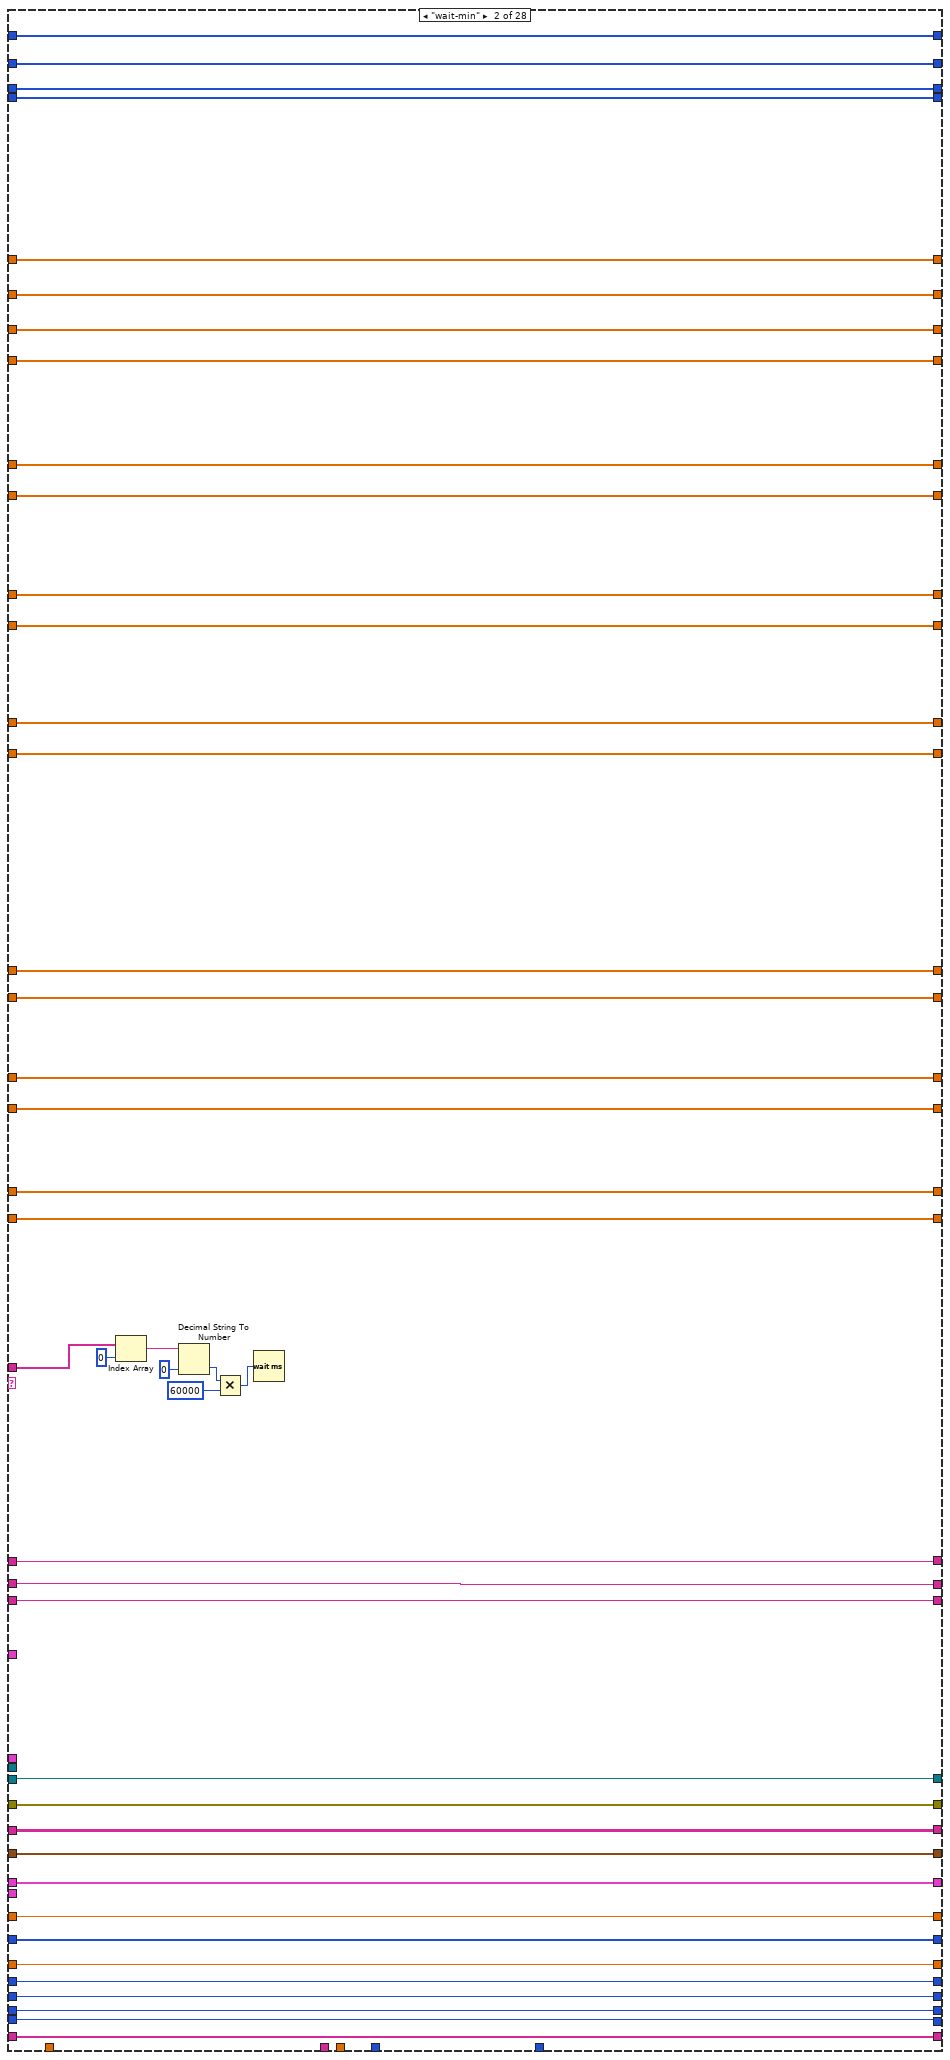
[diagram p7: hidden frame]
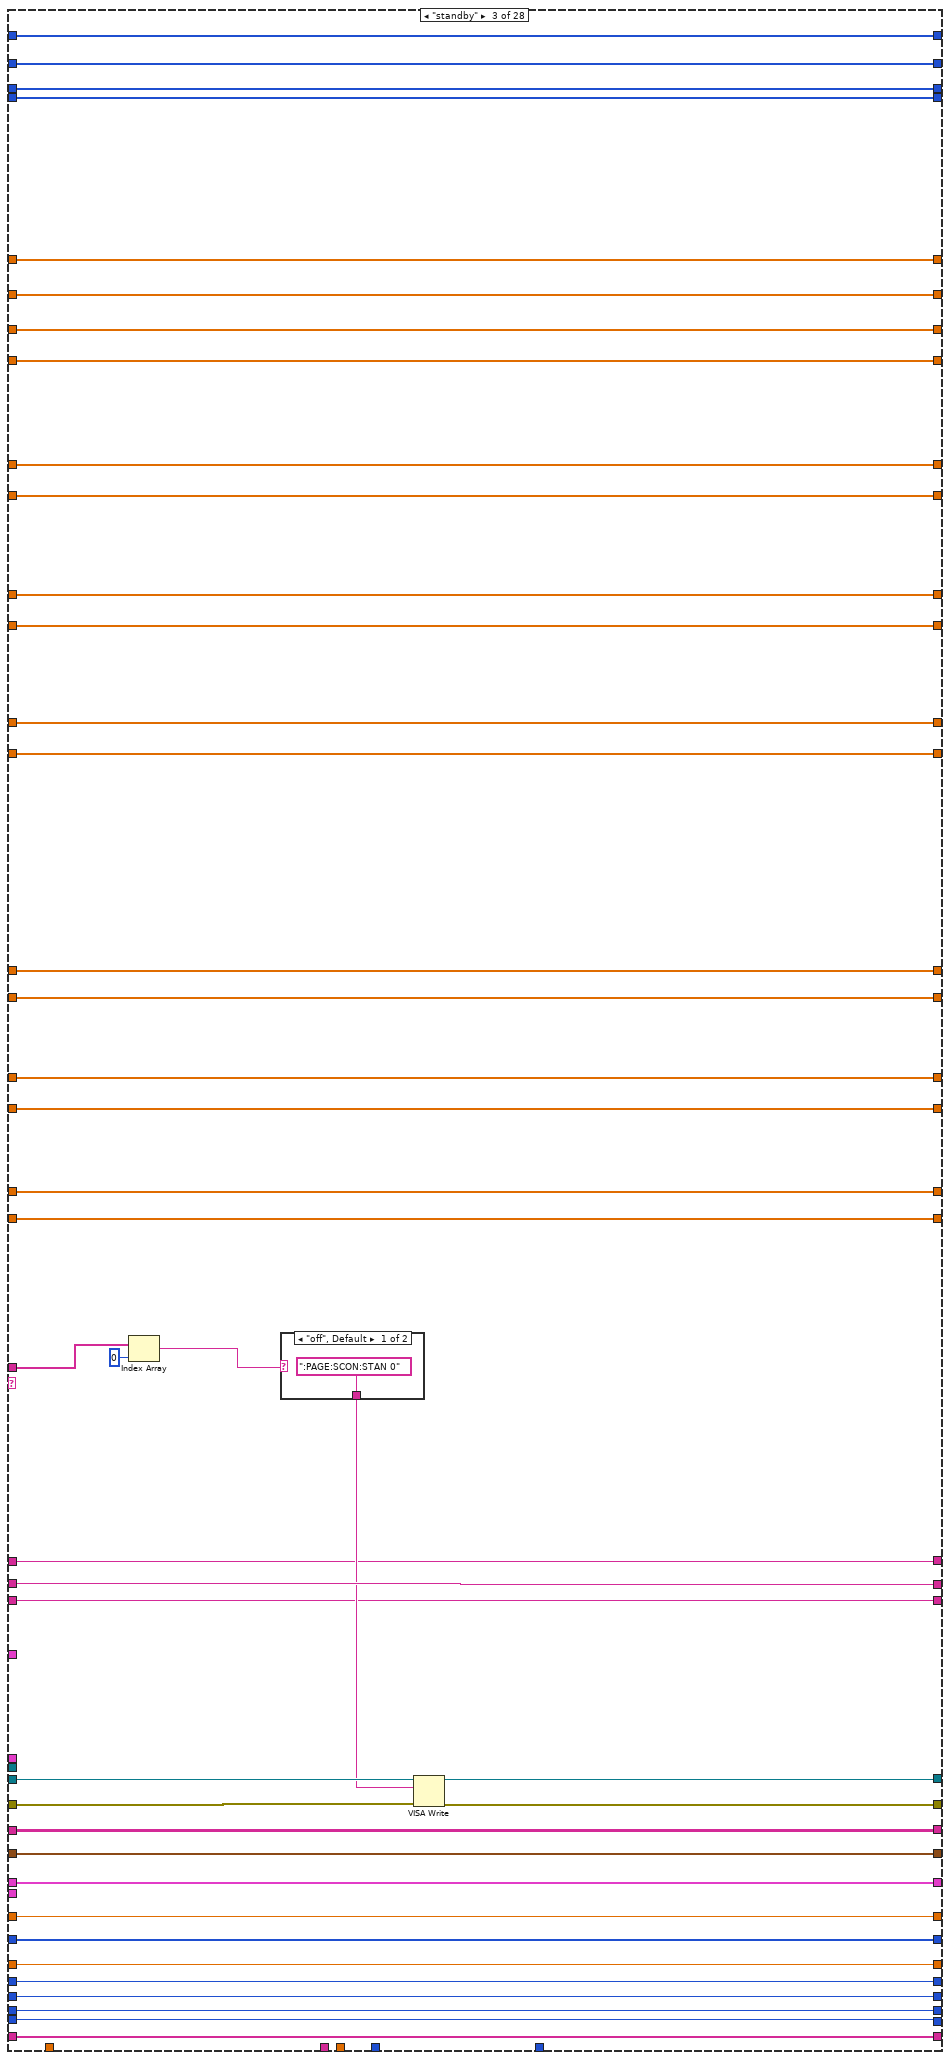
[diagram p8: hidden frame]
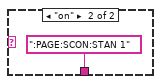
[diagram p9: hidden frame]
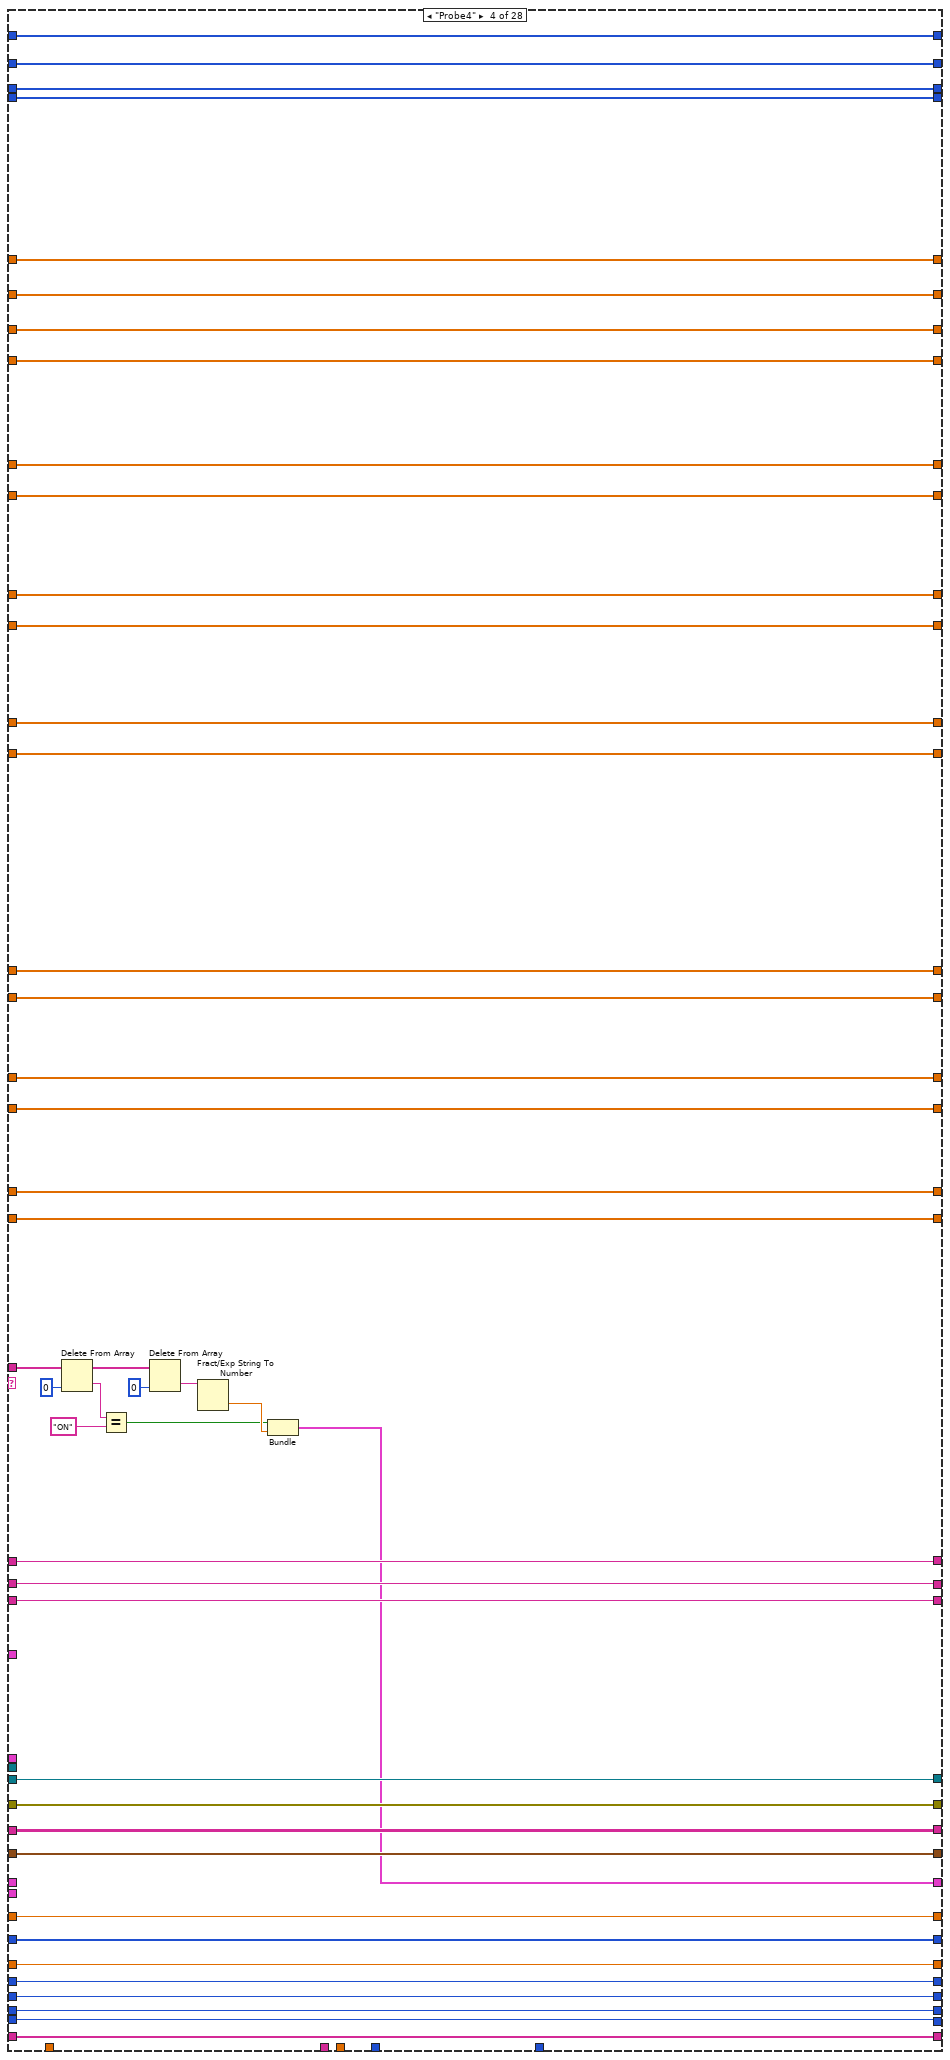
[diagram p10: hidden frame]
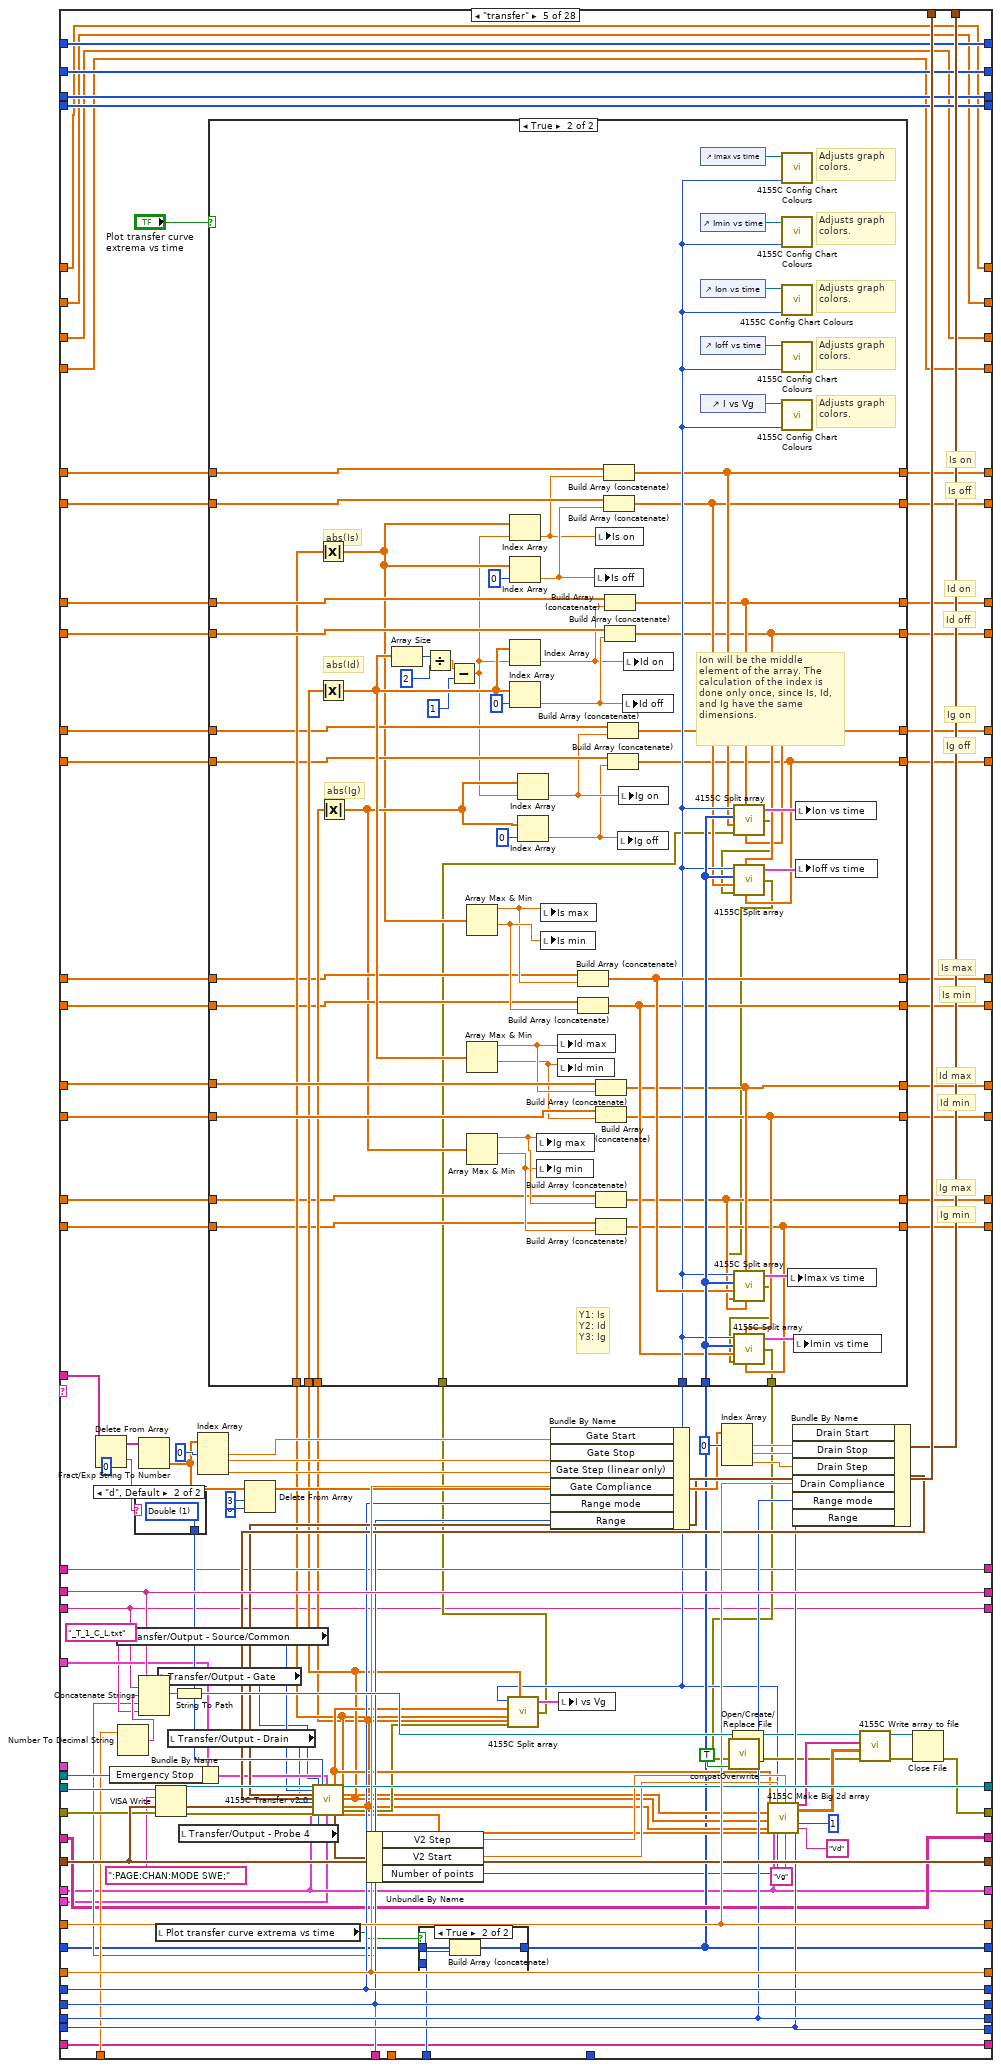
[diagram p11: hidden frame]
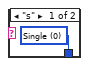
[diagram p14: hidden frame]
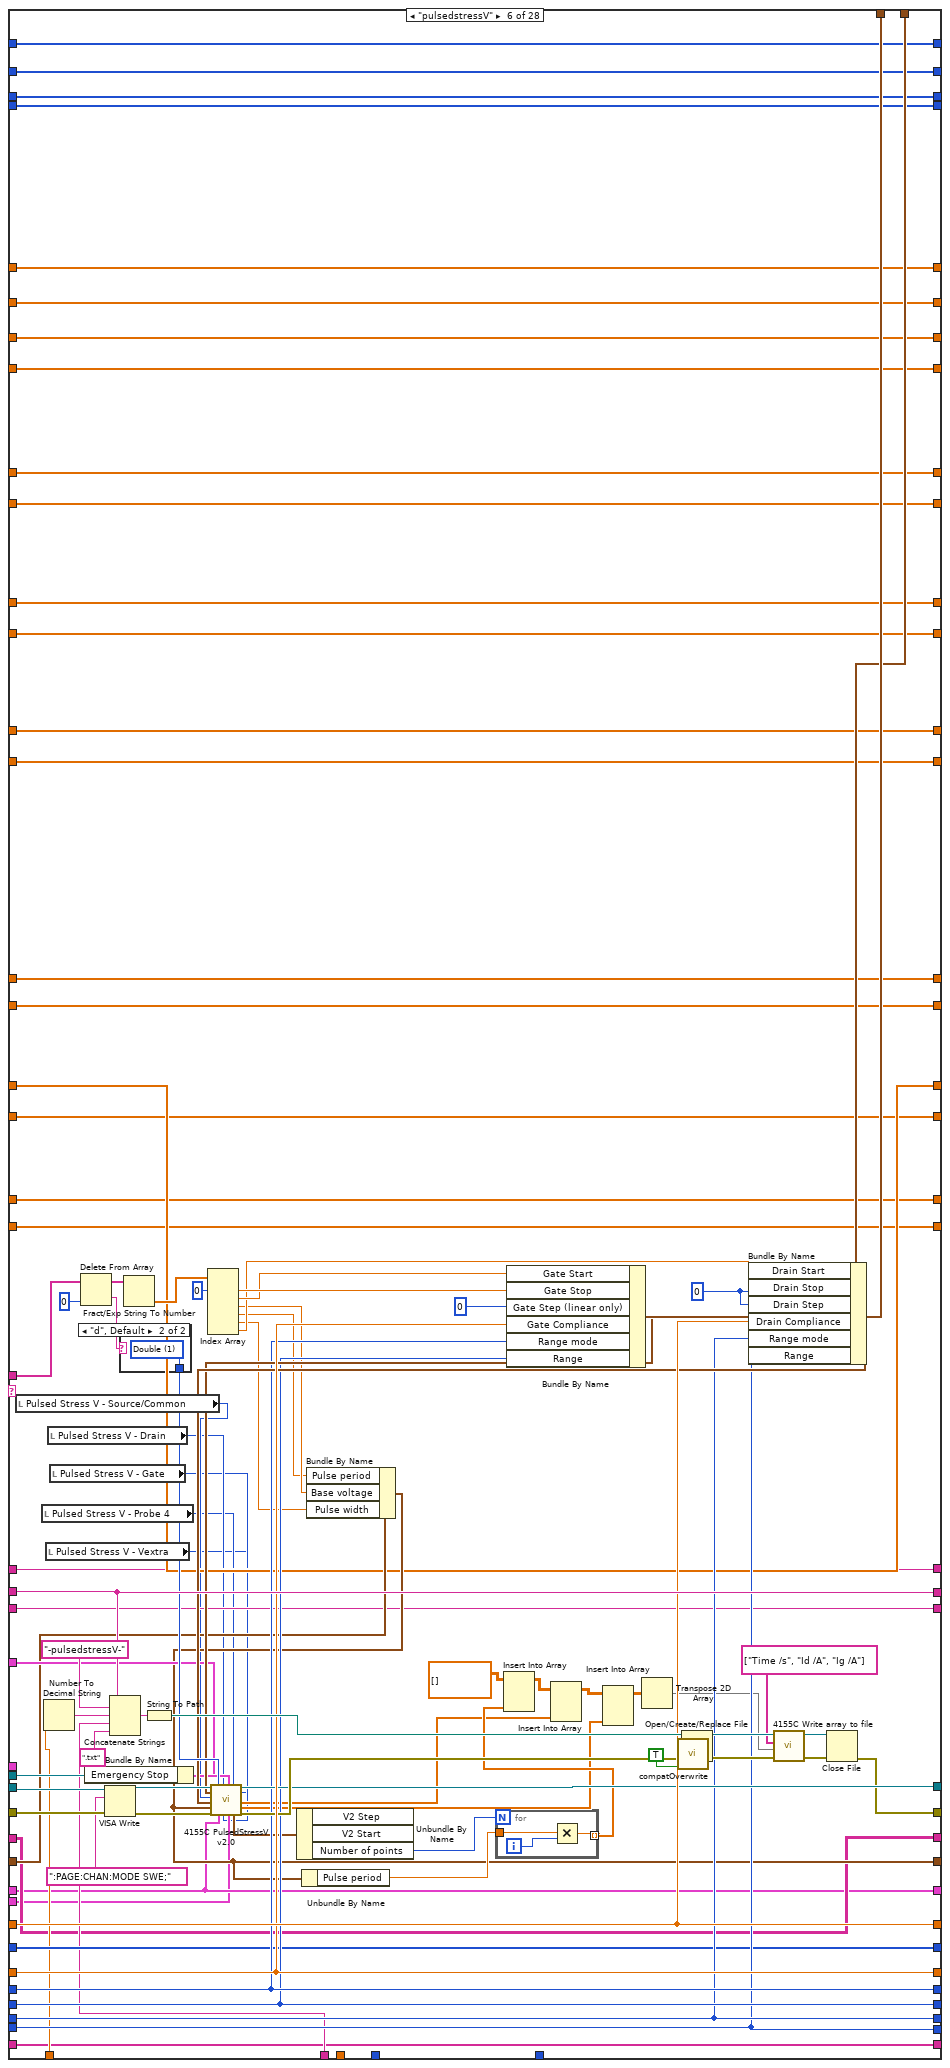
[diagram p15: hidden frame]
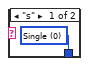
[diagram p16: hidden frame]
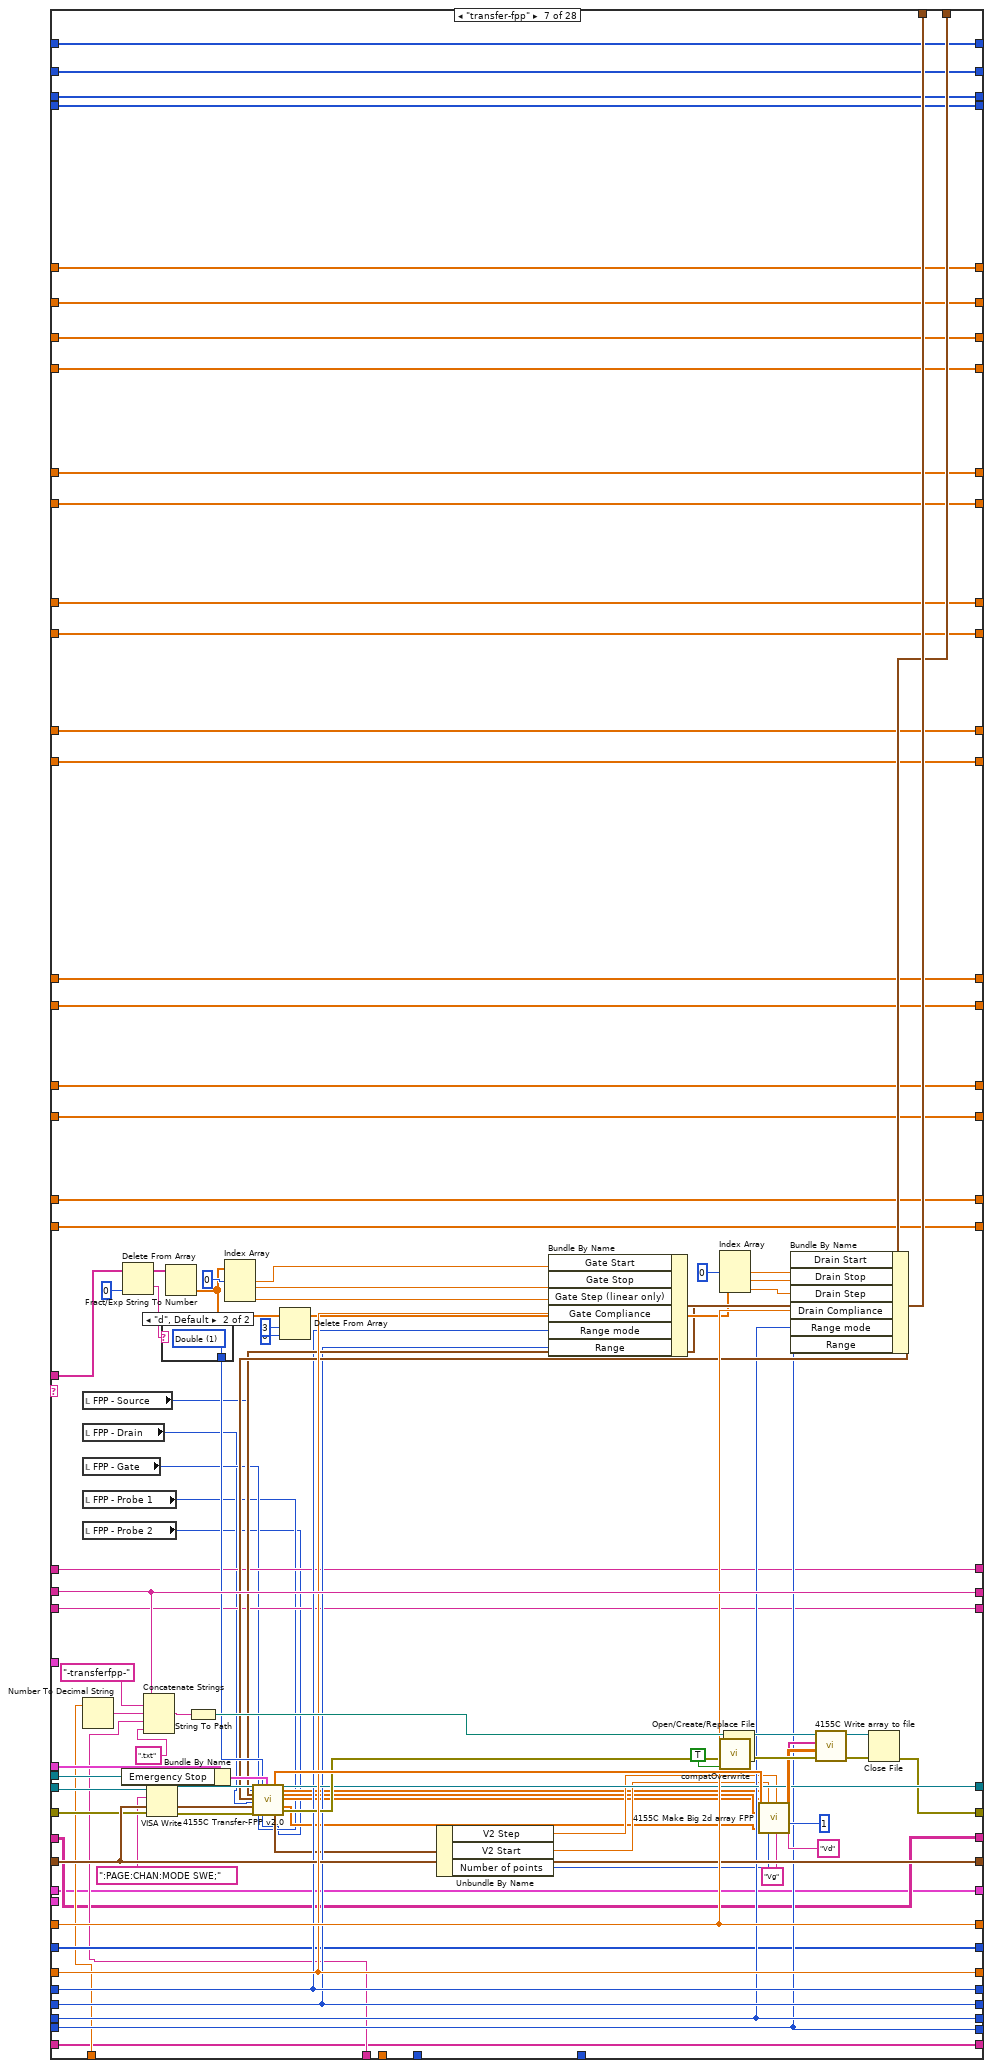
[diagram p17: hidden frame]
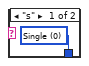
[diagram p18: hidden frame]
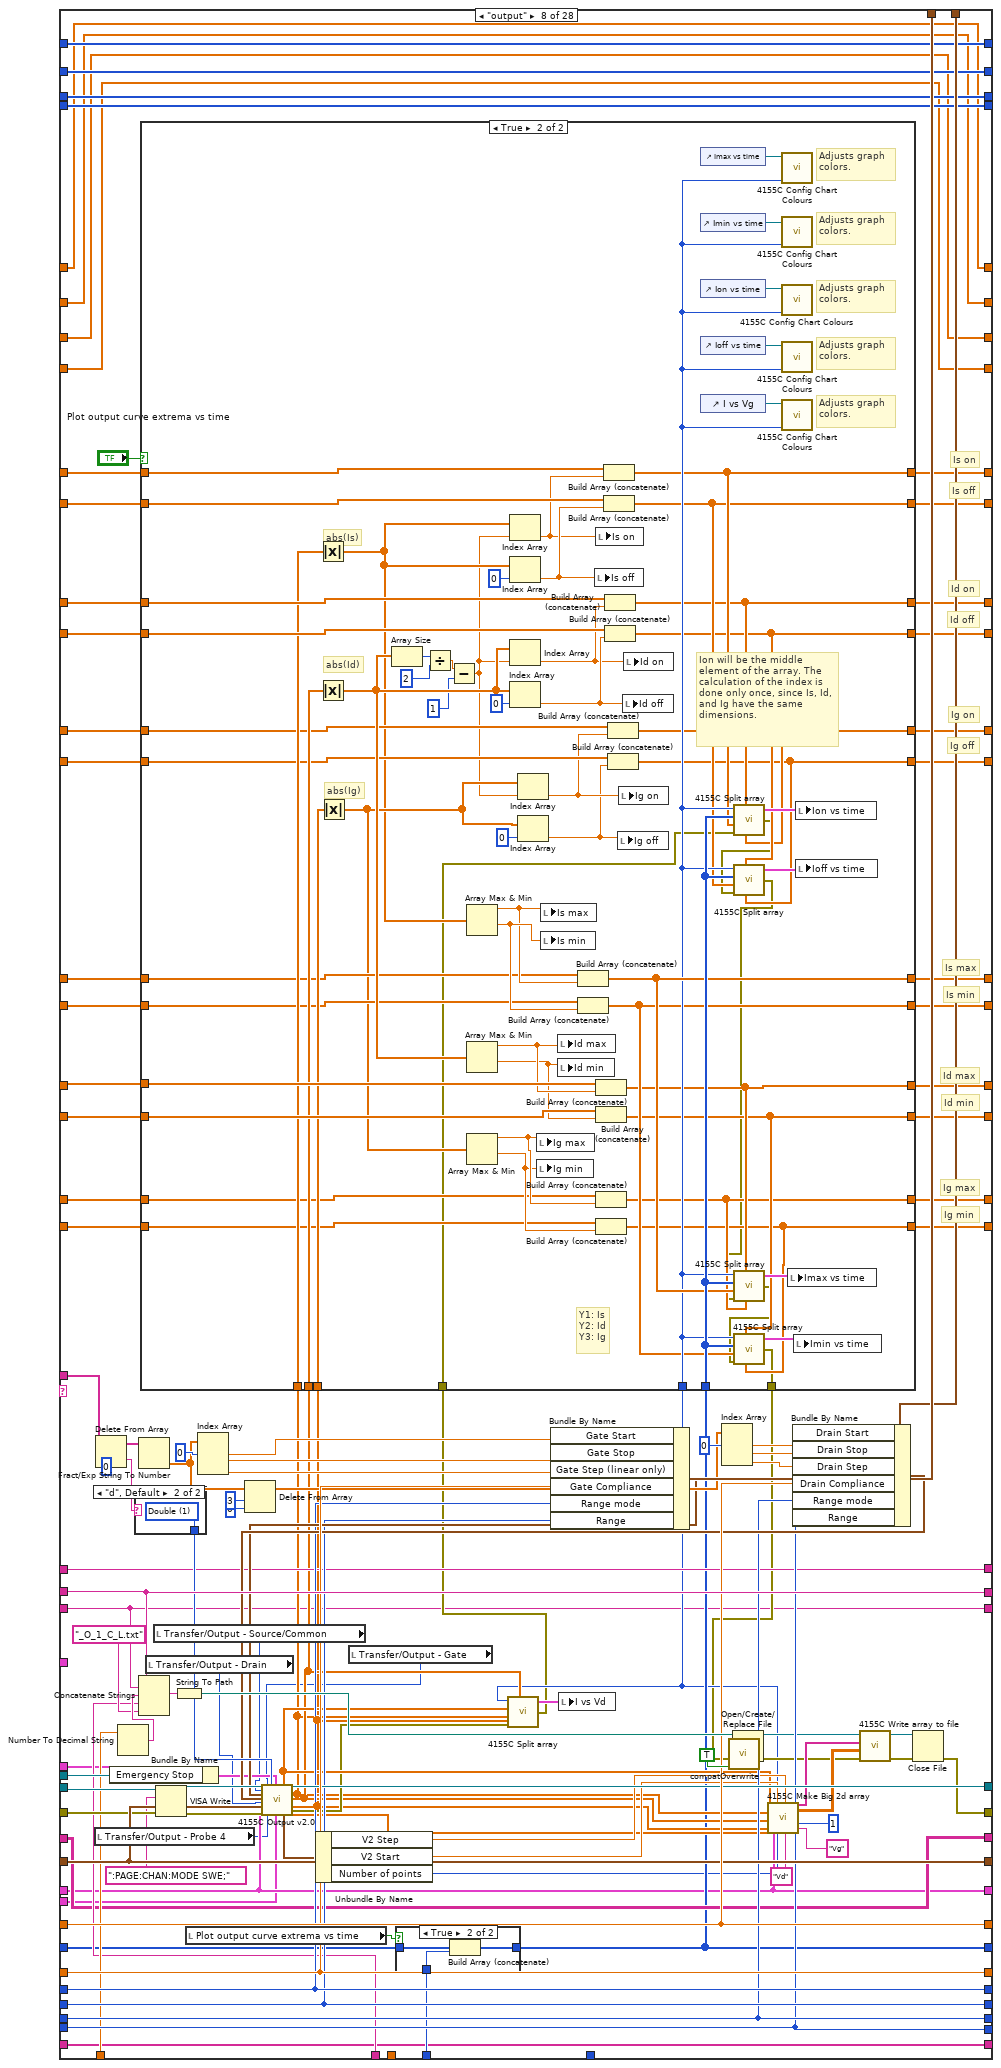
[diagram p19: hidden frame]
diagram:
  w1 = cluster{"Y data in":dbl[], "X data in":dbl[]}[] [] ("I vs Vg")
  w12 = 0.0 ("Is off")
  w13 = 0.0 ("Is on")
  w14 = 0.0 ("Is min")
  w15 = 0.0 ("Is max")
  w63 = u16 1 items=["Reset All", "Partial reset"] ("Type of reset")
  # "Change from previous version:\n\n- Added SMU control."
  # "This is a version specific to the SPM pump."
  # "I add 1 to both the \"total lines\" and the \"line running\" indicators because i and N begin from 0, and the script lines begin from 1."
  # "Bugs:\n\n- If using the \"filename\" command, keep in mind that the arrays of the time-dependent data are not re-initialized inbetween filename changes. \n\n- Do not connect the \"error\" wire of a Split block if it has unconnected terminals! It will halt the program."
  # "Array size"
  # "%s option converts a spreadsheet string to an array of strings."
  # "0: No of rows of array\n1: No of cols"
  # "Dimitrios Simatos\nv. 6.8"
  # "Changes from original textcontrol.vi:\n\n- Timestamp appears in filename.\n- (Only) transfer and output curves are plotted.\n- Communication with serial port.\n- Can execute any command, as all pattern matching functions were replaced. Previously, commands with special LabVIEW characters could not be executed.\n- Replaced write to file function with write to text file.\n- Replaced while loop with for loop.\n- Replaced 4155C \"Save File\" function and now the vi can save time-dependent variables.\n- Added clock with start time control and various units.\n- Changed filepath in which the program is saved.\n- Added a serial output log that keeps a history.\n- Tab control.\n- Addition of specialized serial read/write file for the SPM OEM pump.\n- Added halt and hard stop.\n- Added option for plotting transfer and output curve extrema vs time.\n- Corrected bug of \"itime\" command. The command did not allow for settting the integration time value, it allowed to set the category of the integration time (short, medium, long). If the time value was beyond the range of the category, then the SPA used the closest value allowed, whilst staying in the category. So, if the integration time was changed to long, but the integration time value was a short one, then the SPA would measure using the minimum long integration time value and not the value that the user intended.\n- Added Probe4 command.\n- Added plotting of \"sample\" plots.\n- Added SMU control."
  # "Search and replace LF with EOL"
  n1 = Equal?(x="integration time", y=u32 0) -> (x = y?=w64:bool)
  n2 = Select(t="Integration time (short)", s=w64, f="Integration time (long)") -> (s? t:f=w16:dbl)
  n3 = call "4155C Get Filename.vi"("error in (no error)"=errorcluster {"status"=FALSE, "code"=0, "source"=""}) -> ("error out"=w58:errorcluster, "path"=w33:path)  [unwired: 2 in, 1 out]
  "Path" <- w33
  n4 = Bundle By Name(cluster="Timings (overwritten by the Front Panel)", "integration time"="integration time", "Short/Long integration time"=w16) -> (w56:T5)
  n5 = Path To String(path=w33) -> (string=w34:string)
  n6 = Search and Replace String(replace all?=TRUE ("replace all? (F)"), input string="Script", search string="\n", replace string="\r\n") -> (result string=w46:string)  [unwired: 4 in, 3 out]
  n7 = Match Pattern(string=w34, regular expression=".txt") -> (before substring=w29:string)  [unwired: 1 in, 3 out]
  n8 = call "4155C Initialise.vi"("VISA resource name in"="VISA resource name in", "Reset"="Full Reset", "Type of reset"=w63, "error in (no error)"=w58, "VISA Timeout Value"=u32 10000) -> ("VISA Resource Name out"=w57:refnum<visa-resource-name>, "error out"=w5:errorcluster)
  n9 = Concatenate Strings(w29, "Suffix (script)") -> (w28:string)
  n10 = Spreadsheet String To Array(delimiter (Tab)="\r\n", format string="%s", spreadsheet string="Script", array type (2D Dbl)="") -> (array=w37:string[][])
  n11 = String To Path(string=w28) -> (path=w8:path)
  n12 = Array Size(array=w37) -> (size(s)=w41:i32[])
  n13 = Initialize Array("") -> (w21:string[])  [unwired: 1 in]
  n14 = Open/Create/Replace File(file path (use dialog)=w8, error in=w5, operation (0:open)=T8."replace or create with confirmation") -> (refnum out=w7:refnum<file>, error out=w6:errorcluster)  [unwired: 3 in, 1 out]
  n15 = Initialize Array(0 ("element")) -> (w23:i32[])  [unwired: 1 in]
  n16 = Initialize Array("") -> (w19:string[][])  [unwired: 2 in]
  n17 = Initialize Array(0.0 ("element")) -> (w2:dbl[])  [unwired: 1 in]
  n18 = Index Array(array=w41, index=0) -> (element=w39:i32)
  n19 = Write to Text File(file (use dialog)=w7, text=w46, error in=w6) -> (error out=w27:errorcluster)  [unwired: 1 in, 2 out]
  n20 = for {
    N: w39 -> [w208]
    shift-left: "Source/Drain Range" -> [w248]
    shift-right: [w244] -> _
    shift-left: "Source/Drain\nRange mode" -> [w249]
    shift-right: [w245] -> _
    shift-left: "Gate Range" -> [w250]
    shift-right: [w246] -> _
    shift-left: "Gate Range\nmode" -> [w251]
    shift-right: [w247] -> _
    shift-left: "Gate: Compliance" -> [w260]
    shift-right: [w256] -> _
    shift-left: "Drain: Compliance" -> [w261]
    shift-right: [w257] -> _
    shift-left: w56 -> [w262]
    shift-right: [w258] -> w17
    shift-left: w27 -> [w263]
    shift-right: [w76] -> w32
    shift-left: w57 -> [w264]
    shift-right: [w259] -> _
    shift-left: w29 -> [w265]
    shift-right: [w75] -> _
    tunnel: "Panel Controls 2" -> [w242]
    shift-right: [w120] -> _
    shift-left: w2 -> [w241]
    shift-right: [w178] -> _
    shift-left: i32[] [] -> [w237]
    tunnel: w37 -> [w236] mode=indexing
    shift-right: [w119] -> _
    shift-left: w2 -> [w213]
    shift-right: [w151] -> _
    shift-left: w21 -> [w200]
    shift-right: [w179] -> _
    shift-left: w23 -> [w195]
    shift-right: [w161] -> _
    shift-left: w23 -> [w194]
    shift-right: [w193] -> _
    shift-left: "" -> [w192]
    shift-right: [w156] -> _
    shift-left: w23 -> [w176]
    shift-right: [w155] -> _
    shift-left: w23 -> [w160]
    shift-right: [w152] -> _
    shift-left: w19 -> [w154]
    shift-right: [w113] -> _
    shift-left: w2 -> [w141]
    shift-right: [w114] -> _
    shift-left: w2 -> [w140]
    shift-right: [w118] -> _
    shift-left: w2 -> [w129]
    shift-right: [w117] -> _
    shift-left: w2 -> [w128]
    shift-right: [w111] -> _
    shift-left: w2 -> [w127]
    shift-right: [w121] -> _
    shift-left: w2 -> [w126]
    shift-right: [w112] -> _
    shift-left: w2 -> [w125]
    shift-right: [w110] -> _
    shift-left: w2 -> [w124]
    shift-right: [w116] -> _
    shift-left: w2 -> [w123]
    shift-right: [w115] -> _
    shift-left: w2 -> [w122]
    shift-right: [w74] -> _
    shift-left: "Filename (variable part)" -> [w105]
    shift-right: [w102] -> w3
    shift-left: "Probe 4" -> [w243]
    shift-right: [w70] -> _
    shift-left: w2 -> [w99]
    shift-right: [w71] -> _
    shift-left: w2 -> [w98]
    shift-right: [w72] -> _
    shift-left: w2 -> [w97]
    shift-right: [w73] -> _
    shift-left: w2 -> [w96]
    i -> [w203]
    stop <- "Interrupt program" stop-if-true
    # "Ig for bias stress plots"
    # "Id for bias stress plots"
    # "Is for bias stress plots"
    # "Time axis for bias stress plots"
    # "Save bias stress curves in file."
    # "Filename prefix"
    # "Is off"
    # "Is on"
    # "Ig off"
    # "Ig on"
    # "Is min"
    # "Is max"
    # "Ig min"
    # "Ig max"
    # "Id min"
    # "Id max"
    # "Id off"
    # "Id on"
    # "Pump status"
    # "Filepath and name"
    # "Pump status"
    # "Limit of command arguments (array columns). Raise if needed."
    # "Serial port data (string)"
    # "Serial port data (table)"
    # "Time array for valve position"
    # "Time array for absolute plunger position"
    # "Valve position"
    # "Absolute plunger position"
    # "Serial port data"
    # "For loop counter"
    # "<-----Equivalent to the 4155C \"Write\" subvi.----->"
    # "Headers"
    # "Save transfer curves in file."
    # "Filepath and name"
    # "Save time-dependent data."
    # "Use the time offset if your measurements do not start at t=0."
    # "Time for Imax, Imin, Ion, Ioff"
    # "Rest of elements of command"
    # "First element of command\n(case select)"
    n21 = Add(x=w203, y=1) -> (x+y=→"Line running":i32)
    n22 = Add(x=w208, y=1) -> (x+y=→"Total lines":i32)
    n23 = Index Array(array=w236, index=0 ("line index")) -> (element=w231:string)
    "Command running:" <- w231
    n24 = control-ref of="Interrupt scan"() -> (w255:refnum<vi>)
    n25 = Spreadsheet String To Array(delimiter (Tab)=" ", format string="%s", spreadsheet string=w231, array type (2D Dbl)=string[] []) -> (array=w229:string[])
    n26 = Delete From Array(array=w229, index=0) -> (deleted portion=w142:string, array with subset deleted=w228:string[])  [unwired: 1 in]
    n27 = call "Elapsed Time"("Reset"="Reset", "Auto Reset"="Auto Reset") -> ("Elapsed Time (s)"=w238:dbl)  [unwired: 10 in, 7 out]
    n28 = case shown="0, Default" "Time Units" {
      tunnel: ["-sec" "-min" "-h"] -> w239
      tunnel: [w269 w273 w276] -> w209
      tunnel: w238 -> [w269 w272 w277]
      frame 0, Default {
      }
      frame 1 {
        n29 = Divide(x=w272, y=60.0) -> (x/y=w273:dbl)
      }
      frame 2 {
        n30 = Divide(x=w277, y=3600.0) -> (x/y=w276:dbl)
      }
    }
    n31 = Add(x=w209, y="Time Offset") -> (x+y=w100:dbl)
    n32 = To Long Integer(number=w100) -> (32bit integer=w101:i32)
    "Elapsed Time" <- w101
    n33 = case shown="\"sample-fpp\"" w142 {
      tunnel: w228 -> [w319 w362 w404 w412 w557 w675 w830 w959 w1130 w1162 w1247 w1298 w1347 w1392 w1430 _ _ w1639 w1769 _ w1885 w1955 w2022 w2121 w2207 w2251 w2326 w2385]
      tunnel: w265 -> [w314 w358 w402 w434 w564 w739 w838 w966 w1138 w1185 w1236 w1290 w1340 w1386 w1423 w1466 w1532 w1565 w1751 w1806 w1872 w1942 w2010 w2115 w2203 w2253 w2328 w2387]
      tunnel: w264 -> [w313 w357 w393 w432 w535 w724 w807 w937 w1106 w1186 w1237 w1291 w1341 w1387 w1424 w1471 w1534 w1644 w1775 w1810 w1891 w1961 w2028 w2127 w2161 w2257 w2332 w2389]
      tunnel: w263 -> [w312 w356 w392 w431 w534 w723 w806 w936 w1103 w1187 w1238 w1292 w1342 w1388 w1425 w1470 w1505 w1643 w1774 w1809 w1890 w1960 w2027 w2126 w2160 w2256 w2331 w2390]
      tunnel: w262 -> [w311 w355 w401 w429 w560 w700 w834 w962 w1134 w1195 w1246 w1289 w1339 w1385 w1422 w1469 w1529 w1614 w1743 w1815 w1865 w1935 w2003 w2114 w2202 w2258 w2333 w2392]
      tunnel: w261 -> [w310 w354 w400 w428 w562 w737 w836 w964 w1136 w1194 w1245 w1297 w1346 w1391 w1429 w1468 w1514 w1642 w1773 w1818 w1889 w1959 w2026 w2125 w2211 w2259 w2334 w2393]
      tunnel: w260 -> [w309 w353 w399 w426 w561 w736 w835 w963 w1135 w1193 w1244 w1296 w1345 w1390 w1428 w1467 w1515 w1622 w1752 w1817 w1873 w1943 w2011 w2116 w2204 w2261 w2335 w2395]
      tunnel: [w313 w357 w391 w432 w559 w734 w832 w961 w1132 w1186 w1237 w1291 w1341 w1387 w1424 w1471 w1534 w1615 w1725 w1808 w1866 w1936 w2004 w2068 w2163 w2257 w2332 w2389] -> w259
      tunnel: [w312 w356 w390 w431 w558 w733 w831 w960 w1131 w1187 w1238 w1292 w1342 w1388 w1425 w1470 w1504 w1623 w1726 w1807 w1874 w1944 w2012 w2067 w2162 w2255 w2330 w2390] -> w175
      tunnel: [w311 w355 w401 w429 w560 w696 w834 w962 w1134 w1188 w1239 w1289 w1339 w1385 w1422 w1469 w1529 w1614 w1743 w1815 w1865 w1935 w2003 w2114 w2202 w2258 w2333 w2392] -> w258
      tunnel: [w310 w354 w400 w428 w562 w737 w836 w964 w1136 w1194 w1245 w1297 w1346 w1391 w1429 w1468 w1514 w1642 w1773 w1818 w1889 w1959 w2026 w2125 w2211 w2259 w2334 w2393] -> w257
      tunnel: [w309 w353 w399 w426 w561 w736 w835 w963 w1135 w1193 w1244 w1296 w1345 w1390 w1428 w1467 w1515 w1622 w1752 w1817 w1873 w1943 w2011 w2116 w2204 w2261 w2335 w2395] -> w256
      tunnel: [w314 w358 w402 w434 w564 w739 w838 w966 w1138 w1185 w1236 w1290 w1340 w1386 w1423 w1466 w1532 w1565 w1751 w1806 w1872 w1942 w2010 w2115 w2203 w2253 w2328 w2387] -> w75
      tunnel: w255 -> [_ _ _ _ w566 w743 w843 w968 w1142 _ _ _ _ _ _ _ _ w1619 w1748 _ w1871 w1941 w2009 w2087 w2179 _ _ _]
      tunnel: "Gate" -> [_ _ _ _ w544 w727 w817 w946 w1117 _ _ _ _ _ _ _ _ _ _ _ _ _ _ _ _ _ _ _]
      tunnel: "Drain 2" -> [_ _ _ _ w543 w726 w816 w945 w1116 _ _ _ _ _ _ _ _ _ _ _ _ _ _ _ _ _ _ _]
      tunnel: "Panel Controls" -> [_ _ _ _ _ _ w815 w866 w1115 _ _ _ _ _ _ _ _ _ _ _ _ _ _ _ _ _ _ _]
      tunnel: w251 -> [w308 w352 w398 w425 w528 w717 w800 w930 w1101 w1192 w1243 _ w1338 w1384 w1421 w1465 w1516 w1610 w1739 w1811 w1861 w1931 w1999 w2110 w2198 w2262 w2336 w2396]
      tunnel: w250 -> [w307 w351 w397 w424 w527 w716 w799 w929 w1100 w1191 w1242 w1295 _ w1375 w1427 w1464 w1517 w1611 w1740 w1812 w1862 w1932 w2000 w2111 w2199 w2263 w2337 w2397]
      tunnel: w249 -> [w306 w350 w396 w423 w526 w715 w798 w928 w1099 w1190 w1241 w1294 w1344 w1389 _ w1463 w1518 w1612 w1741 w1813 w1863 w1933 w2001 w2112 w2200 w2264 w2338 w2398]
      tunnel: w248 -> [w305 w349 w395 w422 w525 w714 w797 w927 w1102 w1189 w1240 w1293 w1343 _ w1426 w1462 w1519 w1613 w1742 w1814 w1864 w1934 w2002 w2113 w2201 w2265 w2339 w2399]
      tunnel: [w308 w352 w398 w425 w528 w717 w800 w930 w1101 w1192 w1243 w1288 w1338 w1384 w1421 w1465 w1516 w1610 w1739 w1811 w1861 w1931 w1999 w2110 w2198 w2262 w2336 w2396] -> w247
      tunnel: [w307 w351 w397 w424 w527 w716 w799 w929 w1100 w1191 w1242 w1295 w1330 w1375 w1427 w1464 w1517 w1611 w1740 w1812 w1862 w1932 w2000 w2111 w2199 w2263 w2337 w2397] -> w246
      tunnel: [w306 w350 w396 w423 w526 w715 w798 w928 w1099 w1190 w1241 w1294 w1344 w1389 w1420 w1463 w1518 w1612 w1741 w1813 w1863 w1933 w2001 w2112 w2200 w2264 w2338 w2398] -> w245
      tunnel: [w305 w349 w395 w422 w525 w714 w797 w927 w1102 w1189 w1240 w1293 w1343 w1376 w1426 w1462 w1519 w1613 w1742 w1814 w1864 w1934 w2002 w2113 w2201 w2265 w2339 w2399] -> w244
      tunnel: w243 -> [w283 w324 w367 _ w461 w663 w763 w863 w1064 w1159 w1213 w1266 w1308 w1353 w1398 w1440 w1476 w1587 w1699 w1784 w1826 w1900 w1969 w2041 w2132 w2216 w2270 w2383]
      tunnel: w242 -> [_ _ _ _ w519 w711 _ _ _ _ _ _ _ _ _ _ _ _ _ _ _ _ _ _ _ _ _ _]
      tunnel: [w304 w345 w388 w439 w476 w688 w787 w879 w1088 w1184 w1234 w1287 w1329 w1374 w1419 w1461 w1500 w1576 w1704 w1805 w1850 w1924 w1993 w2065 w2156 w2254 w2329 w2404] -> w120
      tunnel: w241 -> [w304 w345 w388 w439 w516 w688 w787 w919 w1088 w1184 w1234 w1287 w1329 w1374 w1419 w1461 w1500 w1583 w1704 w1805 w1850 w1924 w1993 w2065 w2156 w2254 w2329 w2404]
      tunnel: w100 -> [_ _ _ _ w515 w685 w785 w918 w1085 _ _ _ _ _ _ _ w1498 w1603 w1721 _ w1847 w1921 w1990 w2062 w2152 _ _ _]
      tunnel: w239 -> [_ _ _ _ w512 w684 w783 w915 w1084 _ _ _ _ _ _ _ w1496 w1601 w1720 _ w1846 w1920 w1989 w2061 w2153 _ w2297 _]
      tunnel: w101 -> [_ _ _ _ w508 _ _ w911 _ _ _ _ _ _ _ _ _ _ _ _ _ _ _ _ _ _ w2300 _]
      tunnel: [w303 w344 w387 w427 w480 w687 w786 w883 w1087 w1183 w1233 w1286 w1328 w1373 w1418 w1460 w1499 w1568 w1723 w1804 w1849 w1923 w1992 w2064 w2155 w2260 w2309 w2394] -> w178
      tunnel: w237 -> [w303 w344 w387 w427 w511 w687 w786 w914 w1087 w1183 w1233 w1286 w1328 w1373 w1418 w1460 w1499 w1572 w1723 w1804 w1849 w1923 w1992 w2064 w2155 w2260 w2309 w2394]
      tunnel: [w302 w343 w386 w438 w475 w683 w782 w878 w1083 w1182 w1232 w1285 w1327 w1372 w1417 w1459 w1495 w1575 w1703 w1803 w1845 w1919 w1988 w2060 w2151 w2249 w2325 w2403] -> w119
      tunnel: w213 -> [w302 w343 w386 w438 w507 w683 w782 w910 w1083 w1182 w1232 w1285 w1327 w1372 w1417 w1459 w1495 w1582 w1703 w1803 w1845 w1919 w1988 w2060 w2151 w2249 w2325 w2403]
      tunnel: [w301 w342 w385 w421 w500 w682 w781 w903 w1082 w1181 w1231 w1284 w1326 w1371 w1416 w1458 w1494 w1600 w1719 w1802 w1844 w1918 w1987 w2059 w2150 w2248 w2324 w2400] -> w151
      tunnel: w200 -> [w301 w342 w385 w421 w500 w682 w781 w903 w1082 w1181 w1231 w1284 w1326 w1371 w1416 w1458 w1494 w1600 w1719 w1802 w1844 w1918 w1987 w2059 w2150 w2247 w2298 w2400]
      tunnel: [w300 w341 w384 w449 w499 w681 w780 w902 w1081 w1180 w1230 w1283 w1325 w1370 w1415 w1457 w1493 w1599 w1718 w1801 w1843 w1917 w1986 w2058 w2149 w2233 w2311 w2414] -> w179
      tunnel: w195 -> [w300 w341 w384 w449 w499 w681 w780 w902 w1081 w1180 w1230 w1283 w1325 w1370 w1415 w1457 w1493 w1599 w1718 w1801 w1843 w1917 w1986 w2058 w2149 w2233 w2310 w2414]
      tunnel: [w299 w340 w383 w451 w498 w680 w779 w901 w1080 w1179 w1229 w1282 w1324 w1369 w1414 w1456 w1492 w1598 w1717 w1800 w1842 w1916 w1985 w2057 w2148 w2232 w2293 w2416] -> w161
      tunnel: w194 -> [w299 w340 w383 w451 w498 w680 w779 w901 w1080 w1179 w1229 w1282 w1324 w1369 w1414 w1456 w1492 w1598 w1717 w1800 w1842 w1916 w1985 w2057 w2148 w2232 w2291 w2416]
      tunnel: [w298 w339 w382 w435 w497 w679 w778 w900 w1079 w1178 w1228 w1281 w1323 w1368 w1413 w1455 w1491 w1597 w1716 w1799 w1841 w1915 w1984 w2056 w2147 w2231 w2290 w2388] -> w193
      tunnel: w192 -> [w298 w339 w382 w435 w497 w679 w778 w900 w1079 w1178 w1228 w1281 w1323 w1368 w1413 w1455 w1491 w1597 w1716 w1799 w1841 w1915 w1984 w2056 w2147 w2231 w2301 w2388]
      tunnel: w101 -> [_ _ _ _ _ _ _ _ _ _ _ _ _ _ _ _ _ _ _ _ _ _ _ _ _ _ w2289 _]
      tunnel: w176 -> [w297 w338 w381 w450 w496 w678 w777 w899 w1078 w1177 w1227 w1280 w1322 w1367 w1412 w1454 w1490 w1596 w1715 w1798 w1840 w1914 w1983 w2055 w2146 w2230 w2288 w2415]
      tunnel: [w297 w338 w381 w450 w496 w678 w777 w899 w1078 w1177 w1227 w1280 w1322 w1367 w1412 w1454 w1490 w1596 w1715 w1798 w1840 w1914 w1983 w2055 w2146 w2230 w2287 w2415] -> w156
      tunnel: [w296 w337 w380 w448 w495 w677 w776 w898 w1077 w1176 w1226 w1279 w1321 w1366 w1411 w1453 w1489 w1595 w1714 w1797 w1839 w1913 w1982 w2054 w2145 w2229 w2286 w2413] -> w155
      tunnel: w160 -> [w296 w337 w380 w448 w495 w677 w776 w898 w1077 w1176 w1226 w1279 w1321 w1366 w1411 w1453 w1489 w1595 w1714 w1797 w1839 w1913 w1982 w2054 w2145 w2229 w2285 w2413]
      tunnel: [w295 w336 w379 w430 w494 w676 w775 w897 w1076 w1175 w1225 w1278 w1320 w1365 w1410 w1452 w1488 w1594 w1713 w1796 w1838 w1912 w1981 w2053 w2144 w2228 w2283 w2391] -> w152
      tunnel: w154 -> [w295 w336 w379 w430 w494 w676 w775 w897 w1076 w1175 w1225 w1278 w1320 w1365 w1410 w1452 w1488 w1594 w1713 w1796 w1838 w1912 w1981 w2053 w2144 w2228 w2282 w2391]
      tunnel: [w293 w334 w377 w444 w469 w673 w773 w872 w1074 w1173 w1224 w1277 w1318 w1363 w1408 w1450 w1486 w1593 w1712 w1795 w1837 w1911 w1979 w2052 w2143 w2227 w2281 w2409] -> w113
      tunnel: w141 -> [w293 w334 w377 w444 w493 w673 w773 w896 w1074 w1173 w1224 w1277 w1318 w1363 w1408 w1450 w1486 w1593 w1712 w1795 w1837 w1911 w1979 w2052 w2143 w2227 w2281 w2409]
      tunnel: [w294 w335 w378 w445 w470 w674 w774 w873 w1075 w1174 w1223 w1276 w1319 w1364 w1409 w1451 w1487 w1592 w1711 w1794 w1836 w1910 w1980 w2051 w2142 w2226 w2280 w2410] -> w114
      tunnel: w140 -> [w294 w335 w378 w445 w492 w674 w774 w895 w1075 w1174 w1223 w1276 w1319 w1364 w1409 w1451 w1487 w1592 w1711 w1794 w1836 w1910 w1980 w2051 w2142 w2226 w2280 w2410]
      tunnel: [w286 w327 w370 w437 w474 w670 w771 w877 w1072 w1166 w1221 w1274 w1316 w1361 w1406 w1448 w1479 w1574 w1702 w1793 w1829 w1903 w1972 w2044 w2137 w2219 w2279 w2402] -> w118
      tunnel: w129 -> [w286 w327 w370 w437 w488 w670 w771 w891 w1072 w1166 w1221 w1274 w1316 w1361 w1406 w1448 w1479 w1581 w1702 w1793 w1829 w1903 w1972 w2044 w2137 w2219 w2279 w2402]
      tunnel: [w285 w326 w369 w436 w473 w671 w772 w876 w1073 w1165 w1222 w1275 w1317 w1362 w1407 w1449 w1478 w1573 w1701 w1792 w1828 w1902 w1971 w2043 w2136 w2218 w2278 w2401] -> w117
      tunnel: w128 -> [w285 w326 w369 w436 w487 w671 w772 w890 w1073 w1165 w1222 w1275 w1317 w1362 w1407 w1449 w1478 w1580 w1701 w1792 w1828 w1902 w1971 w2043 w2136 w2218 w2278 w2401]
      tunnel: [w288 w329 w372 w441 w479 w669 w769 w882 w1070 w1171 w1219 w1272 w1314 w1359 w1404 w1446 w1481 w1578 w1706 w1787 w1831 w1905 w1974 w2046 w2135 w2223 w2276 w2406] -> w111
      tunnel: w127 -> [w288 w329 w372 w441 w486 w669 w769 w889 w1070 w1171 w1219 w1272 w1314 w1359 w1404 w1446 w1481 w1585 w1706 w1787 w1831 w1905 w1974 w2046 w2135 w2223 w2276 w2406]
      tunnel: [w287 w328 w371 w440 w477 w672 w770 w880 w1071 w1172 w1220 w1273 w1315 w1360 w1405 w1447 w1480 w1577 w1705 w1786 w1830 w1904 w1973 w2045 w2134 w2222 w2277 w2405] -> w121
      tunnel: w126 -> [w287 w328 w371 w440 w485 w672 w770 w888 w1071 w1172 w1220 w1273 w1315 w1360 w1405 w1447 w1480 w1584 w1705 w1786 w1830 w1904 w1973 w2045 w2134 w2222 w2277 w2405]
      tunnel: [w290 w331 w374 w443 w468 w668 w767 w871 w1068 w1169 w1217 w1270 w1312 w1357 w1402 w1444 w1483 w1589 w1708 w1789 w1833 w1907 w1976 w2048 w2139 w2225 w2274 w2408] -> w112
      tunnel: w125 -> [w290 w331 w374 w443 w484 w668 w767 w887 w1068 w1169 w1217 w1270 w1312 w1357 w1402 w1444 w1483 w1589 w1708 w1789 w1833 w1907 w1976 w2048 w2139 w2225 w2274 w2408]
      tunnel: [w289 w330 w373 w442 w467 w667 w768 w870 w1069 w1170 w1218 w1271 w1313 w1358 w1403 w1445 w1482 w1588 w1707 w1788 w1832 w1906 w1975 w2047 w2138 w2224 w2275 w2407] -> w110
      tunnel: w124 -> [w289 w330 w373 w442 w483 w667 w768 w886 w1069 w1170 w1218 w1271 w1313 w1358 w1403 w1445 w1482 w1588 w1707 w1788 w1832 w1906 w1975 w2047 w2138 w2224 w2275 w2407]
      tunnel: [w292 w333 w376 w447 w472 w666 w765 w875 w1066 w1167 w1215 w1268 w1310 w1355 w1400 w1442 w1485 w1591 w1710 w1791 w1835 w1909 w1978 w2050 w2141 w2221 w2272 w2412] -> w116
      tunnel: w123 -> [w292 w333 w376 w447 w482 w666 w765 w885 w1066 w1167 w1215 w1268 w1310 w1355 w1400 w1442 w1485 w1591 w1710 w1791 w1835 w1909 w1978 w2050 w2141 w2221 w2272 w2412]
      tunnel: [w291 w332 w375 w446 w471 w665 w766 w874 w1067 w1168 w1216 w1269 w1311 w1356 w1401 w1443 w1484 w1590 w1709 w1790 w1834 w1908 w1977 w2049 w2140 w2220 w2273 w2411] -> w115
      tunnel: w122 -> [w291 w332 w375 w446 w481 w665 w766 w884 w1067 w1168 w1216 w1269 w1311 w1356 w1401 w1443 w1484 w1590 w1709 w1790 w1834 w1908 w1977 w2049 w2140 w2220 w2273 w2411]
      tunnel: w105 -> [w284 w325 w368 w433 w464 w664 w764 w867 w1065 w1164 w1214 w1267 w1309 w1354 w1399 w1441 w1477 w1564 w1700 w1785 w1827 w1901 w1970 w2042 w2133 w2217 w2271 _]
      tunnel: [w284 w325 w368 w433 w464 w664 w764 w867 w1065 w1164 w1214 w1267 w1309 w1354 w1399 w1441 w1477 w1564 w1700 w1785 w1827 w1901 w1970 w2042 w2133 w2217 w2271 w2384] -> w74
      tunnel: [w283 w324 w367 w411 w461 w663 w763 w863 w1064 w1159 w1213 w1266 w1308 w1353 w1398 w1440 w1476 w1587 w1699 w1784 w1826 w1900 w1969 w2041 w2132 w2216 w2270 w2383] -> w102
      tunnel: w100 -> [_ _ _ _ _ _ _ _ _ _ _ _ _ _ _ _ _ w1563 _ _ _ _ _ _ _ _ _ _]
      tunnel: [w282 w323 w366 w410 w460 w662 w762 w862 w1063 w1158 w1212 w1265 w1307 w1352 w1397 w1439 w1475 w1547 w1698 w1783 w1825 w1899 w1968 w2040 w2131 w2215 w2269 w2382] -> w70
      tunnel: [w281 w322 w365 w409 w459 w661 w761 w861 w1062 w1157 w1211 w1264 w1306 w1351 w1396 w1438 w1474 w1546 w1697 w1782 w1824 w1898 w1967 w2039 w2130 w2214 w2268 w2381] -> w71
      tunnel: [w280 w321 w364 w408 w458 w660 w760 w860 w1061 w1156 w1210 w1263 w1305 w1350 w1395 w1437 w1473 w1548 w1696 w1781 w1823 w1897 w1966 w2038 w2129 w2213 w2267 w2380] -> w72
      tunnel: [w279 w320 w363 w407 w457 w659 w759 w859 w1060 w1155 w1209 w1262 w1304 w1349 w1394 w1436 w1472 w1545 w1695 w1780 w1822 w1896 w1965 w2037 w2128 w2212 w2266 w2379] -> w73
      tunnel: w99 -> [w282 w323 w366 w410 w460 w662 w762 w862 w1063 w1158 w1212 w1265 w1307 w1352 w1397 w1439 w1475 w1544 w1698 w1783 w1825 w1899 w1968 w2040 w2131 w2215 w2269 w2382]
      tunnel: w98 -> [w281 w322 w365 w409 w459 w661 w761 w861 w1062 w1157 w1211 w1264 w1306 w1351 w1396 w1438 w1474 w1543 w1697 w1782 w1824 w1898 w1967 w2039 w2130 w2214 w2268 w2381]
      tunnel: w97 -> [w280 w321 w364 w408 w458 w660 w760 w860 w1061 w1156 w1210 w1263 w1305 w1350 w1395 w1437 w1473 w1542 w1696 w1781 w1823 w1897 w1966 w2038 w2129 w2213 w2267 w2380]
      tunnel: w96 -> [w279 w320 w363 w407 w457 w659 w759 w859 w1060 w1155 w1209 w1262 w1304 w1349 w1394 w1436 w1472 w1541 w1695 w1780 w1822 w1896 w1965 w2037 w2128 w2212 w2266 w2379]
      tunnel: "Standby" -> [_ _ _ _ w456 w658 _ w858 _ _ _ _ _ _ _ _ _ w1539 w1694 _ _ _ _ w2036 _ _ _ _]
      frame "wait" {
        n34 = Index Array(array=w319, index=0 ("Index")) -> (element=w317:string)
        n35 = Decimal String To Number(string=w317, default (0L)=u32 0) -> (number=w316:u32)  [unwired: 1 in, 1 out]
        n36 = Wait (ms)(milliseconds to wait=w316) -> ()  [unwired: 1 out]
      }
      frame "wait-min" {
        n37 = Index Array(array=w362, index=0 ("Index")) -> (element=w360:string)
        n38 = Decimal String To Number(string=w360, default (0L)=u32 0) -> (number=w348:u32)  [unwired: 1 in, 1 out]
        n39 = Multiply(x=w348, y=u32 60000) -> (x*y=w347:u32)
        n40 = Wait (ms)(milliseconds to wait=w347) -> ()  [unwired: 1 out]
      }
      frame "standby" {
        n41 = Index Array(array=w404, index=0 ("Index")) -> (element=w394:string)
        n42 = case shown="\"off\", Default" w394 {
          tunnel: [":PAGE:SCON:STAN 0" ":PAGE:SCON:STAN 1"] -> w389
          frame "off", Default {
          }
          frame "on" {
          }
        }
        n43 = VISA Write(VISA resource name=w393, write buffer=w389, error in (no error)=w392) -> (VISA resource name out=w391:refnum<visa-resource-name>, error out=w390:errorcluster)  [unwired: 1 out]
      }
      frame "Probe4" {
        n44 = Delete From Array(array=w412, index=0) -> (deleted portion=w415:string, array with subset deleted=w418:string[])  [unwired: 1 in]
        n45 = Equal?(x=w415, y="ON") -> (x = y?=w413:bool)
        n46 = Delete From Array(array=w418, index=0) -> (deleted portion=w417:string)  [unwired: 1 in, 1 out]
        n47 = Fract/Exp String To Number(string=w417) -> (number=w414:dbl)  [unwired: 3 in, 1 out]
        n48 = Bundle(w413, w414) -> (w411:cluster{bool, dbl})  [unwired: 1 in]
      }
      frame "transfer" {
        # "Is off"
        # "Is on"
        # "Ig off"
        # "Ig on"
        # "Is min"
        # "Is max"
        # "Ig min"
        # "Ig max"
        # "Id min"
        # "Id max"
        # "Id off"
        # "Id on"
        n49 = Delete From Array(array=w557, index=0 ("Index")) -> (deleted portion=w555:string, array with subset deleted=w554:string[])  [unwired: 1 in]
        n50 = Bundle By Name(cluster=w519, "Emergency Stop"=w566) -> (w520:T2)
        n51 = local read "Transfer/Output - Source/Common"() -> (w455:u32)
        n52 = Number To Decimal String(number=w515) -> (decimal integer string=w514:string)  [unwired: 1 in]
        n53 = case shown="\"d\", Default" w555 {
          tunnel: [w651 w652] -> w553
          frame "s" {
            w651 = u16 0 items=["Single", "Double"] ("sweep mode")
          }
          frame "d", Default {
            w652 = u16 1 items=["Single", "Double"] ("sweep mode")
          }
        }
        n54 = Fract/Exp String To Number(string=w554) -> (number=w539:dbl[])  [unwired: 3 in, 1 out]
        n55 = Concatenate Strings(w564, w464, w514, w512, "_T_1_C_L.txt" ("Suffix (transfer)")) -> (w565:string)
        n56 = VISA Write(VISA resource name=w535, write buffer=":PAGE:CHAN:MODE SWE;" ("write buffer (\"\")"), error in (no error)=w534) -> (VISA resource name out=w532:refnum<visa-resource-name>, error out=w533:errorcluster)  [unwired: 1 out]
        n57 = local read "Plot transfer curve extrema vs time"() -> (w462:bool)
        n58 = local read "Transfer/Output - Gate"() -> (w453:u32)
        n59 = local read "Transfer/Output - Drain"() -> (w454:u32)
        n60 = String To Path(string=w565) -> (path=w563:path)
        n61 = local read "Transfer/Output - Probe 4"() -> (w452:u32)
        n62 = Index Array(array=w539, index #1=0 ("Index")) -> (element #1=w552:dbl, element #2=w551:dbl, element #3=w550:dbl)  [unwired: 2 in]
        n63 = Delete From Array(array=w539, length=3 ("Length"), index=0 ("Index")) -> (array with subset deleted=w537:dbl[])  [unwired: 1 out]
        n64 = case shown="True" w462 {
          tunnel: w511 -> [w568 w571]
          tunnel: w508 -> [_ w570]
          tunnel: [w568 w569] -> w480
          frame False {
          }
          frame True {
            n65 = Build Array (concatenate)(w571, w570) -> (w569:i32[])
          }
        }
        n66 = Bundle By Name(cluster=w544, "Gate Start"=w552, "Gate Stop"=w551, "Gate Step (linear only)"=w550, "Gate Compliance"=w561, "Range mode"=w528, "Range"=w527) -> (w529:T6)
        n67 = Index Array(array=w537, index #1=0 ("Index")) -> (element #1=w547:dbl, element #2=w546:dbl, element #3=w545:dbl)  [unwired: 2 in]
        n68 = call <vilib>:"compatOverwrite.vi"("overwrite (F)"=TRUE) -> ("overwrite?"=w518:T8)
        n69 = Bundle By Name(cluster=w543, "Drain Start"=w547, "Drain Stop"=w546, "Drain Step"=w545, "Drain Compliance"=w562, "Range mode"=w526, "Range"=w525) -> (w530:T7)
        n70 = call "4155C Transfer v2.0.vi"("VISA resource name in"=w532, "Source/Common"=w455, 2:"Gate"=w529, 3:"Drain"=w530, 4:"Drain"=w454, "Timings"=w560, "error in (no error)"=w533, 7:"Probe 4"=w461, 8:"Gate"=w453, 9:"Probe 4"=w452, "sweep mode"=w553, "Panel Controls"=w520, "Standby"=w456) -> ("VG"=w517:dbl[], "Outparams"=w524:T9, "VISA Resource Name out"=w559:refnum<visa-resource-name>, "IS"=w490:dbl[], "ID"=w491:dbl[], "IG"=w489:dbl[], "error out"=w509:errorcluster, "Probe 4"=w521:dbl[])  [unwired: 7 in]
        n71 = Unbundle By Name(w524) -> ("V2 Step"=w523:dbl, "V2 Start"=w522:dbl, "Number of points"=w478:i32)
        n72 = call "4155C Split array.vi"("Number of VAR2 steps"=w478, "Y2 data in"=w491, "X data in"=w517, "Y1 data in"=w490, "Y3 data in"=w489, "error in (no error)"=w509) -> ("Array of clusters"=w510:cluster{"Y data in":dbl[], "X data in":dbl[]}[], "error out"=w466:errorcluster)  [unwired: 1 in]
        n73 = case shown="True" "Plot transfer curve extrema vs time" {
          tunnel: w516 -> [w580 w650]
          tunnel: w507 -> [w581 w645]
          tunnel: w493 -> [w574 w641]
          tunnel: w492 -> [w575 w640]
          tunnel: w491 -> [_ w637]
          tunnel: w490 -> [_ w635]
          tunnel: w489 -> [_ w634]
          tunnel: w488 -> [w582 w630]
          tunnel: w487 -> [w583 w629]
          tunnel: w486 -> [w578 w626]
          tunnel: w485 -> [w579 w625]
          tunnel: w484 -> [w573 w622]
          tunnel: w483 -> [w572 w621]
          tunnel: w482 -> [w577 w618]
          tunnel: w481 -> [w576 w617]
          tunnel: w480 -> [_ w610]
          tunnel: [w578 w605] -> w479
          tunnel: w478 -> [_ w604]
          tunnel: [w579 w603] -> w477
          tunnel: [w580 w602] -> w476
          tunnel: [w581 w601] -> w475
          tunnel: [w582 w600] -> w474
          tunnel: [w583 w599] -> w473
          tunnel: [w577 w598] -> w472
          tunnel: [w576 w597] -> w471
          tunnel: [w575 w596] -> w470
          tunnel: [w574 w595] -> w469
          tunnel: [w573 w594] -> w468
          tunnel: [w572 w593] -> w467
          tunnel: w466 -> [w584 w592]
          tunnel: [w584 w588] -> w465
          frame False {
          }
          frame True {
            # "Adjusts graph colors."
            # "Adjusts graph colors."
            # "Ion will be the middle element of the array. The calculation of the index is done only once, since Is, Id, and Ig have the same dimensions."
            # "abs(Ig)"
            # "abs(Is)"
            # "Y1: Is\nY2: Id\nY3: Ig"
            # "abs(Id)"
            # "Adjusts graph colors."
            # "Adjusts graph colors."
            # "Adjusts graph colors."
            n74 = Absolute Value(x=w635) -> (abs(x)=w620:dbl[])
            n75 = Absolute Value(x=w637) -> (abs(x)=w636:dbl[])
            n76 = Absolute Value(x=w634) -> (abs(x)=w623:dbl[])
            n77 = Array Size(array=w636) -> (size(s)=w644:i32)
            n78 = Divide(x=w644, y=2) -> (x/y=w587:dbl)
            n79 = Subtract(x=w587, y=1) -> (x-y=w586:dbl)
            n80 = Array Max & Min(array=w620) -> (max value=w627:dbl, min value=w628:dbl)  [unwired: 2 out]
            n81 = Array Max & Min(array=w636) -> (max value=w649:dbl, min value=w633:dbl)  [unwired: 2 out]
            n82 = Array Max & Min(array=w623) -> (max value=w632:dbl, min value=w631:dbl)  [unwired: 2 out]
            n83 = Index Array(array=w620, index=w586) -> (element=w611:dbl)
            n84 = Index Array(array=w620, index=0) -> (element=w612:dbl)
            n85 = Index Array(array=w636, index=w586) -> (element=w613:dbl)
            n86 = Index Array(array=w636, index=0) -> (element=w614:dbl)
            n87 = Index Array(array=w623, index=w586) -> (element=w616:dbl)
            n88 = Index Array(array=w623, index=0) -> (element=w615:dbl)
            n89 = local write "Ig max"(w632) -> ()
            n90 = local write "Ig min"(w631) -> ()
            n91 = local write "Is max"(w627) -> ()
            n92 = local write "Is min"(w628) -> ()
            n93 = local write "Id max"(w649) -> ()
            n94 = local write "Id min"(w633) -> ()
            n95 = Build Array (concatenate)(w626, w627) -> (w605:dbl[])
            n96 = Build Array (concatenate)(w625, w628) -> (w603:dbl[])
            n97 = local write "Is off"(w612) -> ()
            n98 = local write "Is on"(w611) -> ()
            n99 = Build Array (concatenate)(w650, w649) -> (w602:dbl[])
            n100 = Build Array (concatenate)(w645, w633) -> (w601:dbl[])
            n101 = Build Array (concatenate)(w630, w632) -> (w600:dbl[])
            n102 = Build Array (concatenate)(w629, w631) -> (w599:dbl[])
            n103 = Build Array (concatenate)(w618, w611) -> (w598:dbl[])
            n104 = Build Array (concatenate)(w617, w612) -> (w597:dbl[])
            n105 = Build Array (concatenate)(w640, w613) -> (w596:dbl[])
            n106 = Build Array (concatenate)(w641, w614) -> (w595:dbl[])
            n107 = Build Array (concatenate)(w622, w616) -> (w594:dbl[])
            n108 = Build Array (concatenate)(w621, w615) -> (w593:dbl[])
            n109 = local write "Ig off"(w615) -> ()
            n110 = local write "Ig on"(w616) -> ()
            n111 = local write "Id off"(w614) -> ()
            n112 = local write "Id on"(w613) -> ()
            n113 = control-ref of="Imax vs time"() -> (w639:refnum<vi>)
            n114 = control-ref of="Imin vs time"() -> (w638:refnum<vi>)
            n115 = control-ref of="Ion vs time"() -> (w607:refnum<vi>)
            n116 = control-ref of="Ioff vs time"() -> (w606:refnum<vi>)
            n117 = control-ref of="I vs Vg"() -> (w648:refnum<vi>)
            n118 = call "4155C Split array.vi"("Number of VAR2 steps"=w604, "Y2 data in"=w596, "X data in"=w610, "Y1 data in"=w598, "Y3 data in"=w594, "error in (no error)"=w592) -> ("Array of clusters"=w608:cluster{"Y data in":dbl[], "X data in":dbl[]}[], "error out"=w591:errorcluster)  [unwired: 1 in]
            n119 = call "4155C Split array.vi"("Number of VAR2 steps"=w604, "Y2 data in"=w595, "X data in"=w610, "Y1 data in"=w597, "Y3 data in"=w593, "error in (no error)"=w591) -> ("Array of clusters"=w609:cluster{"Y data in":dbl[], "X data in":dbl[]}[], "error out"=w590:errorcluster)  [unwired: 1 in]
            n120 = call "4155C Split array.vi"("Number of VAR2 steps"=w604, "Y2 data in"=w602, "X data in"=w610, "Y1 data in"=w605, "Y3 data in"=w600, "error in (no error)"=w590) -> ("Array of clusters"=w647:cluster{"Y data in":dbl[], "X data in":dbl[]}[], "error out"=w589:errorcluster)  [unwired: 1 in]
            n121 = call "4155C Split array.vi"("Number of VAR2 steps"=w604, "Y2 data in"=w601, "X data in"=w610, "Y1 data in"=w603, "Y3 data in"=w599, "error in (no error)"=w589) -> ("Array of clusters"=w646:cluster{"Y data in":dbl[], "X data in":dbl[]}[], "error out"=w588:errorcluster)  [unwired: 1 in]
            n122 = call "4155C Config Chart Colours.vi"("Numeric"=w604, "XY Graph 2"=w639) -> ()  [unwired: 6 in]
            n123 = call "4155C Config Chart Colours.vi"("Numeric"=w604, "XY Graph 2"=w638) -> ()  [unwired: 6 in]
            n124 = call "4155C Config Chart Colours.vi"("Numeric"=w604, "XY Graph 2"=w607) -> ()  [unwired: 6 in]
            n125 = call "4155C Config Chart Colours.vi"("Numeric"=w604, "XY Graph 2"=w606) -> ()  [unwired: 6 in]
            n126 = call "4155C Config Chart Colours.vi"("Numeric"=w604, "XY Graph 2"=w648) -> ()  [unwired: 6 in]
            n127 = local write "Imax vs time"(w647) -> ()
            n128 = local write "Imin vs time"(w646) -> ()
            n129 = local write "Ion vs time"(w608) -> ()
            n130 = local write "Ioff vs time"(w609) -> ()
          }
        }
        n131 = local write "I vs Vg"(w510) -> ()
        n132 = Open/Create/Replace File(file path (use dialog)=w563, error in=w465, operation (0:open)=w518) -> (refnum out=w505:refnum<file>, error out=w503:errorcluster)  [unwired: 3 in, 1 out]
        n133 = call "4155C Make Big 2d array.vi"("1D Var1"=w517, "1d IS"=w490, "1d ID"=w491, "1d IG"=w489, "1d SMU4"=w521, "SMU4"=w461, "VAR2 START"=w522, "Number of VAR2 steps"=w478, "VAR2 STEP"=w523, "VAR1 Name"="Vg", "Decimal places in header"=i8 1, "VAR2 Name"="Vd") -> ("Header array"=w506:string[], "Data array"=w504:dbl[][])  [unwired: 14 in]
        n134 = call "4155C Write array to file.vi"("Byte Stream File Refnum"=w505, "Header"=w506, "Data Array"=w504, "error in (no error)"=w503) -> ("dup refnum"=w502:refnum<file>, "error out"=w501:errorcluster)  [unwired: 1 in]
        n135 = Close File(refnum=w502, error in=w501) -> (error out=w558:errorcluster)  [unwired: 1 out]
      }
      frame "pulsedstressV" {
        w694 = 0
        n136 = local read "Pulsed Stress V - Source/Common"() -> (w657:u32)
        n137 = local read "Pulsed Stress V - Probe 4"() -> (w654:u32)
        n138 = Number To Decimal String(number=w685) -> (decimal integer string=w740:string)  [unwired: 1 in]
        n139 = local read "Pulsed Stress V - Vextra"() -> (w653:u32)
        n140 = local read "Pulsed Stress V - Drain"() -> (w656:u32)
        n141 = local read "Pulsed Stress V - Gate"() -> (w655:u32)
        n142 = Delete From Array(array=w675, index=0 ("Index")) -> (deleted portion=w731:string, array with subset deleted=w730:string[])  [unwired: 1 in]
        n143 = Bundle By Name(cluster=w711, "Emergency Stop"=w743) -> (w712:T2)
        n144 = VISA Write(VISA resource name=w724, write buffer=":PAGE:CHAN:MODE SWE;" ("write buffer (\"\")"), error in (no error)=w723) -> (VISA resource name out=w721:refnum<visa-resource-name>, error out=w722:errorcluster)  [unwired: 1 out]
        n145 = Concatenate Strings(w739, "-pulsedstressV-" ("Substring"), w740, w684, ".txt" ("Substring")) -> (w742:string)
        n146 = case shown="\"d\", Default" w731 {
          tunnel: [w752 w753] -> w729
          frame "s" {
            w752 = u16 0 items=["Single", "Double"] ("sweep mode")
          }
          frame "d", Default {
            w753 = u16 1 items=["Single", "Double"] ("sweep mode")
          }
        }
        n147 = Fract/Exp String To Number(string=w730) -> (number=w725:dbl[])  [unwired: 3 in, 1 out]
        n148 = String To Path(string=w742) -> (path=w738:path)
        n149 = Index Array(array=w725, index #1=0 ("Index")) -> (element #1=w703:dbl, element #2=w702:dbl, element #3=w699:dbl, element #4=w698:dbl, element #5=w697:dbl, element #6=w701:dbl)  [unwired: 5 in]
        n150 = Bundle By Name(cluster=w700, "Pulse period"=w698, "Base voltage"=w699, "Pulse width"=w697) -> (w696:T5)
        n151 = Unbundle By Name(w696) -> ("Pulse period"=w704:dbl)
        n152 = Bundle By Name(cluster=w727, "Gate Start"=w702, "Gate Stop"=w703, "Gate Step (linear only)"=0, "Gate Compliance"=w736, "Range mode"=w717, "Range"=w716) -> (w718:T6)
        n153 = call <vilib>:"compatOverwrite.vi"("overwrite (F)"=TRUE) -> ("overwrite?"=w689:T8)
        n154 = Bundle By Name(cluster=w726, "Drain Start"=w701, "Drain Stop"=w694, "Drain Step"=w694, "Drain Compliance"=w737, "Range mode"=w715, "Range"=w714) -> (w719:T7)
        n155 = call "4155C PulsedStressV v2.0.vi"("VISA resource name in"=w721, "Gate"=w718, "Pulsed Stress V - Source/Common"=w657, "Drain"=w719, "Timings"=w696, "error in (no error)"=w722, "sweep mode"=w729, "Probe 4"=w663, "Pulsed Stress V - Drain"=w656, "Pulsed Stress V - Gate"=w655, "Panel Controls"=w712, "Standby"=w658, "Pulsed Stress V - Probe 4"=w654, "Pulsed Stress V - Vextra"=w653) -> ("Outparams"=w713:T9, "VISA Resource Name out"=w734:refnum<visa-resource-name>, "ID"=w692:dbl[], "IG"=w690:dbl[], "error out"=w735:errorcluster)  [unwired: 1 in]
        n156 = Unbundle By Name(w713) -> ("Number of points"=w691:i32)  [unwired: 2 out]
        n157 = for {
          N: w691 -> [_]
          tunnel: [w749] -> w693 mode=indexing
          tunnel: w704 -> [w751]
          i -> [w750]
          n158 = Multiply(x=w751, y=w750) -> (x*y=w749:dbl)
        }
        n159 = Insert Into Array(array=dbl[][] [] ("Input Array"), new element=w693) -> (w705:dbl[][])  [unwired: 2 in]
        n160 = Insert Into Array(array=w705, new element=w692) -> (w710:dbl[][])  [unwired: 2 in]
        n161 = Insert Into Array(array=w710, new element=w690) -> (w709:dbl[][])  [unwired: 2 in]
        n162 = Transpose 2D Array(2D array=w709) -> (transposed array=w708:dbl[][])
        n163 = Open/Create/Replace File(file path (use dialog)=w738, error in=w735, operation (0:open)=w689) -> (refnum out=w746:refnum<file>, error out=w747:errorcluster)  [unwired: 3 in, 1 out]
        n164 = call "4155C Write array to file.vi"("Byte Stream File Refnum"=w746, "Header"=string[] ["Time /s", "Id /A", "Ig /A"], "Data Array"=w708, "error in (no error)"=w747) -> ("dup refnum"=w744:refnum<file>, "error out"=w745:errorcluster)  [unwired: 1 in]
        n165 = Close File(refnum=w744, error in=w745) -> (error out=w733:errorcluster)  [unwired: 1 out]
      }
      frame "transfer-fpp" {
        n166 = local read "FPP - Source"() -> (w758:u32)
        n167 = local read "FPP - Drain"() -> (w756:u32)
        n168 = local read "FPP - Gate"() -> (w757:u32)
        n169 = local read "FPP - Probe 1"() -> (w755:u32)
        n170 = local read "FPP - Probe 2"() -> (w754:u32)
        n171 = Number To Decimal String(number=w785) -> (decimal integer string=w839:string)  [unwired: 1 in]
        n172 = Bundle By Name(cluster=w815, "Emergency Stop"=w843) -> (w851:T1)
        n173 = Delete From Array(array=w830, index=0 ("Index")) -> (deleted portion=w828:string, array with subset deleted=w827:string[])  [unwired: 1 in]
        n174 = Concatenate Strings(w838, "-transferfpp-" ("Substring"), w839, w783, ".txt" ("Substring")) -> (w841:string)
        n175 = VISA Write(VISA resource name=w807, write buffer=":PAGE:CHAN:MODE SWE;" ("write buffer (\"\")"), error in (no error)=w806) -> (VISA resource name out=w804:refnum<visa-resource-name>, error out=w805:errorcluster)  [unwired: 1 out]
        n176 = case shown="\"d\", Default" w828 {
          tunnel: [w852 w853] -> w826
          frame "s" {
            w852 = u16 0 items=["Single", "Double"] ("sweep mode")
          }
          frame "d", Default {
            w853 = u16 1 items=["Single", "Double"] ("sweep mode")
          }
        }
        n177 = Fract/Exp String To Number(string=w827) -> (number=w811:dbl[])  [unwired: 3 in, 1 out]
        n178 = String To Path(string=w841) -> (path=w837:path)
        n179 = Index Array(array=w811, index #1=0 ("Index")) -> (element #1=w825:dbl, element #2=w824:dbl, element #3=w823:dbl)  [unwired: 2 in]
        n180 = Delete From Array(array=w811, length=3 ("Length"), index=0 ("Index")) -> (array with subset deleted=w809:dbl[])  [unwired: 1 out]
        n181 = Bundle By Name(cluster=w817, "Gate Start"=w825, "Gate Stop"=w824, "Gate Step (linear only)"=w823, "Gate Compliance"=w835, "Range mode"=w800, "Range"=w799) -> (w801:T6)
        n182 = Index Array(array=w809, index #1=0 ("Index")) -> (element #1=w820:dbl, element #2=w819:dbl, element #3=w818:dbl)  [unwired: 2 in]
        n183 = call <vilib>:"compatOverwrite.vi"("overwrite (F)"=TRUE) -> ("overwrite?"=w788:T8)
        n184 = Bundle By Name(cluster=w816, "Drain Start"=w820, "Drain Stop"=w819, "Drain Step"=w818, "Drain Compliance"=w836, "Range mode"=w798, "Range"=w797) -> (w802:T7)
        n185 = call "4155C Transfer-FPP v2.0.vi"("VISA resource name in"=w804, "FPP - Source"=w758, "Gate"=w801, "Drain"=w802, "FPP - Drain"=w756, "Timings"=w834, "error in (no error)"=w805, "FPP - Gate"=w757, "FPP - Probe 1"=w755, "sweep mode"=w826, "FPP - Probe 2"=w754, "Panel Controls"=w851) -> ("VG"=w842:dbl[], "Outparams"=w796:T9, "VISA Resource Name out"=w832:refnum<visa-resource-name>, "Vprobe2"=w792:dbl[], "ID"=w791:dbl[], "IG"=w790:dbl[], "Vprobe1"=w789:dbl[], "error out"=w833:errorcluster)  [unwired: 8 in]
        n186 = Unbundle By Name(w796) -> ("V2 Step"=w795:dbl, "V2 Start"=w794:dbl, "Number of points"=w793:i32)
        n187 = Open/Create/Replace File(file path (use dialog)=w837, error in=w833, operation (0:open)=w788) -> (refnum out=w848:refnum<file>, error out=w849:errorcluster)  [unwired: 3 in, 1 out]
        n188 = call "4155C Make Big 2d array FPP.vi"("1D Var1"=w842, "1d ID"=w791, "1d Vp2"=w792, "1d IG"=w790, "1d Vp1"=w789, "VAR2 START"=w794, "Number of VAR2 steps"=w793, "VAR2 STEP"=w795, "VAR1 Name"="Vg", "Decimal places in header"=i8 1, "VAR2 Name"="Vd") -> ("Header array"=w844:string[], "Data array"=w845:dbl[][])  [unwired: 15 in]
        n189 = call "4155C Write array to file.vi"("Byte Stream File Refnum"=w848, "Header"=w844, "Data Array"=w845, "error in (no error)"=w849) -> ("dup refnum"=w846:refnum<file>, "error out"=w847:errorcluster)  [unwired: 1 in]
        n190 = Close File(refnum=w846, error in=w847) -> (error out=w831:errorcluster)  [unwired: 1 out]
      }
      frame "output" {
        # "Is off"
        # "Is on"
        # "Ig off"
        # "Ig on"
        # "Is min"
        # "Is max"
        # "Ig min"
        # "Ig max"
        # "Id min"
        # "Id max"
        # "Id off"
        # "Id on"
        n191 = local read "Transfer/Output - Probe 4"() -> (w854:u32)
        n192 = Delete From Array(array=w959, index=0 ("Index")) -> (deleted portion=w957:string, array with subset deleted=w956:string[])  [unwired: 1 in]
        n193 = Bundle By Name(cluster=w866, "Emergency Stop"=w968) -> (w922:T1)
        n194 = Number To Decimal String(number=w918) -> (decimal integer string=w917:string)  [unwired: 1 in]
        n195 = case shown="\"d\", Default" w957 {
          tunnel: [w1053 w1054] -> w955
          frame "s" {
            w1053 = u16 0 items=["Single", "Double"] ("sweep mode")
          }
          frame "d", Default {
            w1054 = u16 1 items=["Single", "Double"] ("sweep mode")
          }
        }
        n196 = Fract/Exp String To Number(string=w956) -> (number=w941:dbl[])  [unwired: 3 in, 1 out]
        n197 = Concatenate Strings(w966, w867, w917, w915, "_O_1_C_L.txt" ("Suffix (transfer)")) -> (w967:string)
        n198 = local read "Transfer/Output - Drain"() -> (w856:u32)
        n199 = local read "Transfer/Output - Source/Common"() -> (w857:u32)
        n200 = VISA Write(VISA resource name=w937, write buffer=":PAGE:CHAN:MODE SWE;" ("write buffer (\"\")"), error in (no error)=w936) -> (VISA resource name out=w934:refnum<visa-resource-name>, error out=w935:errorcluster)  [unwired: 1 out]
        n201 = String To Path(string=w967) -> (path=w965:path)
        n202 = local read "Plot output curve extrema vs time"() -> (w864:bool)
        n203 = Index Array(array=w941, index #1=0 ("Index")) -> (element #1=w954:dbl, element #2=w953:dbl, element #3=w952:dbl)  [unwired: 2 in]
        n204 = Delete From Array(array=w941, length=3 ("Length"), index=0 ("Index")) -> (array with subset deleted=w939:dbl[])  [unwired: 1 out]
        n205 = local read "Transfer/Output - Gate"() -> (w855:u32)
        n206 = case shown="True" w864 {
          tunnel: w914 -> [w970 w973]
          tunnel: w911 -> [_ w972]
          tunnel: [w970 w971] -> w883
          frame False {
          }
          frame True {
            n207 = Build Array (concatenate)(w973, w972) -> (w971:i32[])
          }
        }
        n208 = Bundle By Name(cluster=w946, "Gate Start"=w954, "Gate Stop"=w953, "Gate Step (linear only)"=w952, "Gate Compliance"=w963, "Range mode"=w930, "Range"=w929) -> (w931:T6)
        n209 = Index Array(array=w939, index #1=0 ("Index")) -> (element #1=w949:dbl, element #2=w948:dbl, element #3=w947:dbl)  [unwired: 2 in]
        n210 = call <vilib>:"compatOverwrite.vi"("overwrite (F)"=TRUE) -> ("overwrite?"=w921:T8)
        n211 = Bundle By Name(cluster=w945, "Drain Start"=w949, "Drain Stop"=w948, "Drain Step"=w947, "Drain Compliance"=w964, "Range mode"=w928, "Range"=w927) -> (w932:T7)
        n212 = call "4155C Output v2.0.vi"("VISA resource name in"=w934, "Source/Common"=w857, 2:"Gate"=w931, 3:"Drain"=w932, 4:"Drain"=w856, "Timings"=w962, "error in (no error)"=w935, 7:"Probe 4"=w863, 8:"Gate"=w855, 9:"Probe 4"=w854, "sweep mode"=w955, "Panel controls"=w922, "Standby"=w858) -> ("VD"=w920:dbl[], "Outparams"=w926:T9, "VISA Resource Name out"=w961:refnum<visa-resource-name>, "IS"=w893:dbl[], "ID"=w894:dbl[], "IG"=w892:dbl[], "error out"=w912:errorcluster, "Probe 4"=w923:dbl[])  [unwired: 7 in]
        n213 = Unbundle By Name(w926) -> ("V2 Step"=w925:dbl, "V2 Start"=w924:dbl, "Number of points"=w881:i32)
        n214 = call "4155C Split array.vi"("Number of VAR2 steps"=w881, "Y2 data in"=w894, "X data in"=w920, "Y1 data in"=w893, "Y3 data in"=w892, "error in (no error)"=w912) -> ("Array of clusters"=w913:cluster{"Y data in":dbl[], "X data in":dbl[]}[], "error out"=w869:errorcluster)  [unwired: 1 in]
        n215 = case shown="True" "Plot output curve extrema vs time" {
          tunnel: w919 -> [w977 w1052]
          tunnel: w910 -> [w976 w1047]
          tunnel: w896 -> [w982 w1043]
          tunnel: w895 -> [w983 w1042]
          tunnel: w894 -> [_ w1039]
          tunnel: w893 -> [_ w1037]
          tunnel: w892 -> [_ w1036]
          tunnel: w891 -> [w975 w1032]
          tunnel: w890 -> [w974 w1031]
          tunnel: w889 -> [w979 w1028]
          tunnel: w888 -> [w978 w1027]
          tunnel: w887 -> [w981 w1024]
          tunnel: w886 -> [w980 w1023]
          tunnel: w885 -> [w985 w1020]
          tunnel: w884 -> [w984 w1019]
          tunnel: w883 -> [_ w1012]
          tunnel: [w979 w1007] -> w882
          tunnel: w881 -> [_ w1006]
          tunnel: [w978 w1005] -> w880
          tunnel: [w977 w1004] -> w879
          tunnel: [w976 w1003] -> w878
          tunnel: [w975 w1002] -> w877
          tunnel: [w974 w1001] -> w876
          tunnel: [w985 w1000] -> w875
          tunnel: [w984 w999] -> w874
          tunnel: [w983 w998] -> w873
          tunnel: [w982 w997] -> w872
          tunnel: [w981 w996] -> w871
          tunnel: [w980 w995] -> w870
          tunnel: w869 -> [w986 w994]
          tunnel: [w986 w990] -> w868
          frame False {
          }
          frame True {
            # "Adjusts graph colors."
            # "Adjusts graph colors."
            # "Ion will be the middle element of the array. The calculation of the index is done only once, since Is, Id, and Ig have the same dimensions."
            # "abs(Ig)"
            # "abs(Is)"
            # "Y1: Is\nY2: Id\nY3: Ig"
            # "abs(Id)"
            # "Adjusts graph colors."
            # "Adjusts graph colors."
            # "Adjusts graph colors."
            n216 = Absolute Value(x=w1037) -> (abs(x)=w1022:dbl[])
            n217 = Absolute Value(x=w1039) -> (abs(x)=w1038:dbl[])
            n218 = Absolute Value(x=w1036) -> (abs(x)=w1025:dbl[])
            n219 = Array Size(array=w1038) -> (size(s)=w1046:i32)
            n220 = Divide(x=w1046, y=2) -> (x/y=w989:dbl)
            n221 = Subtract(x=w989, y=1) -> (x-y=w988:dbl)
            n222 = Array Max & Min(array=w1022) -> (max value=w1029:dbl, min value=w1030:dbl)  [unwired: 2 out]
            n223 = Array Max & Min(array=w1038) -> (max value=w1051:dbl, min value=w1035:dbl)  [unwired: 2 out]
            n224 = Array Max & Min(array=w1025) -> (max value=w1034:dbl, min value=w1033:dbl)  [unwired: 2 out]
            n225 = Index Array(array=w1022, index=w988) -> (element=w1013:dbl)
            n226 = Index Array(array=w1022, index=0) -> (element=w1014:dbl)
            n227 = Index Array(array=w1038, index=w988) -> (element=w1015:dbl)
            n228 = Index Array(array=w1038, index=0) -> (element=w1016:dbl)
            n229 = Index Array(array=w1025, index=w988) -> (element=w1018:dbl)
            n230 = Index Array(array=w1025, index=0) -> (element=w1017:dbl)
            n231 = local write "Ig max"(w1034) -> ()
            n232 = local write "Ig min"(w1033) -> ()
            n233 = local write "Is max"(w1029) -> ()
            n234 = local write "Is min"(w1030) -> ()
            n235 = local write "Id max"(w1051) -> ()
            n236 = local write "Id min"(w1035) -> ()
            n237 = Build Array (concatenate)(w1028, w1029) -> (w1007:dbl[])
            n238 = Build Array (concatenate)(w1027, w1030) -> (w1005:dbl[])
            n239 = local write "Is off"(w1014) -> ()
            n240 = local write "Is on"(w1013) -> ()
            n241 = Build Array (concatenate)(w1052, w1051) -> (w1004:dbl[])
            n242 = Build Array (concatenate)(w1047, w1035) -> (w1003:dbl[])
            n243 = Build Array (concatenate)(w1032, w1034) -> (w1002:dbl[])
            n244 = Build Array (concatenate)(w1031, w1033) -> (w1001:dbl[])
            n245 = Build Array (concatenate)(w1020, w1013) -> (w1000:dbl[])
            n246 = Build Array (concatenate)(w1019, w1014) -> (w999:dbl[])
            n247 = Build Array (concatenate)(w1042, w1015) -> (w998:dbl[])
            n248 = Build Array (concatenate)(w1043, w1016) -> (w997:dbl[])
            n249 = Build Array (concatenate)(w1024, w1018) -> (w996:dbl[])
            n250 = Build Array (concatenate)(w1023, w1017) -> (w995:dbl[])
            n251 = local write "Ig off"(w1017) -> ()
            n252 = local write "Ig on"(w1018) -> ()
            n253 = local write "Id off"(w1016) -> ()
            n254 = local write "Id on"(w1015) -> ()
            n255 = control-ref of="Imax vs time"() -> (w1041:refnum<vi>)
            n256 = control-ref of="Imin vs time"() -> (w1040:refnum<vi>)
            n257 = control-ref of="Ion vs time"() -> (w1009:refnum<vi>)
            n258 = control-ref of="Ioff vs time"() -> (w1008:refnum<vi>)
            n259 = control-ref of="I vs Vg"() -> (w1050:refnum<vi>)
            n260 = call "4155C Split array.vi"("Number of VAR2 steps"=w1006, "Y2 data in"=w998, "X data in"=w1012, "Y1 data in"=w1000, "Y3 data in"=w996, "error in (no error)"=w994) -> ("Array of clusters"=w1010:cluster{"Y data in":dbl[], "X data in":dbl[]}[], "error out"=w993:errorcluster)  [unwired: 1 in]
            n261 = call "4155C Split array.vi"("Number of VAR2 steps"=w1006, "Y2 data in"=w997, "X data in"=w1012, "Y1 data in"=w999, "Y3 data in"=w995, "error in (no error)"=w993) -> ("Array of clusters"=w1011:cluster{"Y data in":dbl[], "X data in":dbl[]}[], "error out"=w992:errorcluster)  [unwired: 1 in]
            n262 = call "4155C Split array.vi"("Number of VAR2 steps"=w1006, "Y2 data in"=w1004, "X data in"=w1012, "Y1 data in"=w1007, "Y3 data in"=w1002, "error in (no error)"=w992) -> ("Array of clusters"=w1049:cluster{"Y data in":dbl[], "X data in":dbl[]}[], "error out"=w991:errorcluster)  [unwired: 1 in]
            n263 = call "4155C Split array.vi"("Number of VAR2 steps"=w1006, "Y2 data in"=w1003, "X data in"=w1012, "Y1 data in"=w1005, "Y3 data in"=w1001, "error in (no error)"=w991) -> ("Array of clusters"=w1048:cluster{"Y data in":dbl[], "X data in":dbl[]}[], "error out"=w990:errorcluster)  [unwired: 1 in]
            n264 = call "4155C Config Chart Colours.vi"("Numeric"=w1006, "XY Graph 2"=w1041) -> ()  [unwired: 6 in]
            n265 = call "4155C Config Chart Colours.vi"("Numeric"=w1006, "XY Graph 2"=w1040) -> ()  [unwired: 6 in]
            n266 = call "4155C Config Chart Colours.vi"("Numeric"=w1006, "XY Graph 2"=w1009) -> ()  [unwired: 6 in]
            n267 = call "4155C Config Chart Colours.vi"("Numeric"=w1006, "XY Graph 2"=w1008) -> ()  [unwired: 6 in]
            n268 = call "4155C Config Chart Colours.vi"("Numeric"=w1006, "XY Graph 2"=w1050) -> ()  [unwired: 6 in]
            n269 = local write "Imax vs time"(w1049) -> ()
            n270 = local write "Imin vs time"(w1048) -> ()
            n271 = local write "Ion vs time"(w1010) -> ()
            n272 = local write "Ioff vs time"(w1011) -> ()
          }
        }
        n273 = local write "I vs Vd"(w913) -> ()
        n274 = Open/Create/Replace File(file path (use dialog)=w965, error in=w868, operation (0:open)=w921) -> (refnum out=w908:refnum<file>, error out=w906:errorcluster)  [unwired: 3 in, 1 out]
        n275 = call "4155C Make Big 2d array.vi"("1D Var1"=w920, "1d IS"=w893, "1d ID"=w894, "1d IG"=w892, "1d SMU4"=w923, "SMU4"=w863, "VAR2 START"=w924, "Number of VAR2 steps"=w881, "VAR2 STEP"=w925, "VAR1 Name"="Vd", "Decimal places in header"=i8 1, "VAR2 Name"="Vg") -> ("Header array"=w909:string[], "Data array"=w907:dbl[][])  [unwired: 14 in]
        n276 = call "4155C Write array to file.vi"("Byte Stream File Refnum"=w908, "Header"=w909, "Data Array"=w907, "error in (no error)"=w906) -> ("dup refnum"=w905:refnum<file>, "error out"=w904:errorcluster)  [unwired: 1 in]
        n277 = Close File(refnum=w905, error in=w904) -> (error out=w960:errorcluster)  [unwired: 1 out]
      }
      frame "output-fpp" {
        n278 = local read "FPP - Source"() -> (w1059:u32)
        n279 = local read "FPP - Drain"() -> (w1058:u32)
        n280 = local read "FPP - Gate"() -> (w1057:u32)
        n281 = local read "FPP - Probe 1"() -> (w1056:u32)
        n282 = local read "FPP - Probe 2"() -> (w1055:u32)
        n283 = Number To Decimal String(number=w1085) -> (decimal integer string=w1139:string)  [unwired: 1 in]
        n284 = Bundle By Name(cluster=w1115, "Emergency Stop"=w1142) -> (w1152:T1)
        n285 = Delete From Array(array=w1130, index=0 ("Index")) -> (deleted portion=w1128:string, array with subset deleted=w1127:string[])  [unwired: 1 in]
        n286 = VISA Write(VISA resource name=w1106, write buffer=":PAGE:CHAN:MODE SWE;" ("write buffer (\"\")"), error in (no error)=w1103) -> (VISA resource name out=w1105:refnum<visa-resource-name>, error out=w1104:errorcluster)  [unwired: 1 out]
        n287 = Concatenate Strings(w1138, "-outputfpp-" ("Substring"), w1139, w1084, ".txt" ("Substring")) -> (w1141:string)
        n288 = case shown="\"d\", Default" w1128 {
          tunnel: [w1153 w1154] -> w1126
          frame "s" {
            w1153 = u16 0 items=["Single", "Double"] ("sweep mode")
          }
          frame "d", Default {
            w1154 = u16 1 items=["Single", "Double"] ("sweep mode")
          }
        }
        n289 = Fract/Exp String To Number(string=w1127) -> (number=w1109:dbl[])  [unwired: 3 in, 1 out]
        n290 = String To Path(string=w1141) -> (path=w1137:path)
        n291 = Index Array(array=w1109, index #1=0 ("Index")) -> (element #1=w1125:dbl, element #2=w1124:dbl, element #3=w1123:dbl)  [unwired: 2 in]
        n292 = Delete From Array(array=w1109, length=3 ("Length"), index=0 ("Index")) -> (array with subset deleted=w1108:dbl[])  [unwired: 1 out]
        n293 = Bundle By Name(cluster=w1117, "Gate Start"=w1125, "Gate Stop"=w1124, "Gate Step (linear only)"=w1123, "Gate Compliance"=w1135, "Range mode"=w1101, "Range"=w1100) -> (w1151:T6)
        n294 = Index Array(array=w1108, index #1=0 ("Index")) -> (element #1=w1120:dbl, element #2=w1119:dbl, element #3=w1118:dbl)  [unwired: 2 in]
        n295 = call <vilib>:"compatOverwrite.vi"("overwrite (F)"=TRUE) -> ("overwrite?"=w1089:T8)
        n296 = Bundle By Name(cluster=w1116, "Drain Start"=w1120, "Drain Stop"=w1119, "Drain Step"=w1118, "Drain Compliance"=w1136, "Range mode"=w1099, "Range"=w1102) -> (w1150:T7)
        n297 = call "4155C Output-FPP v2.0.vi"("VISA resource name in"=w1105, "FPP - Source"=w1059, "Gate"=w1151, "Drain"=w1150, "FPP - Drain"=w1058, "Timings"=w1134, "error in (no error)"=w1104, "FPP - Gate"=w1057, "FPP - Probe 1"=w1056, "sweep mode"=w1126, "FPP - Probe 2"=w1055, "Panel controls"=w1152) -> ("VD"=w1094:dbl[], "Outparams"=w1097:T9, "VISA Resource Name out"=w1132:refnum<visa-resource-name>, "Vprobe2"=w1093:dbl[], "ID"=w1092:dbl[], "IG"=w1091:dbl[], "Vprobe1"=w1090:dbl[], "error out"=w1133:errorcluster)  [unwired: 8 in]
        n298 = Unbundle By Name(w1097) -> ("V2 Step"=w1098:dbl, "V2 Start"=w1096:dbl, "Number of points"=w1095:i32)
        n299 = Open/Create/Replace File(file path (use dialog)=w1137, error in=w1133, operation (0:open)=w1089) -> (refnum out=w1147:refnum<file>, error out=w1148:errorcluster)  [unwired: 3 in, 1 out]
        n300 = call "4155C Make Big 2d array FPP.vi"("1D Var1"=w1094, "1d ID"=w1092, "1d Vp2"=w1093, "1d IG"=w1091, "1d Vp1"=w1090, "VAR2 START"=w1096, "Number of VAR2 steps"=w1095, "VAR2 STEP"=w1098, "VAR1 Name"="Vd", "Decimal places in header"=i8 1, "VAR2 Name"="Vg") -> ("Header array"=w1143:string[], "Data array"=w1144:dbl[][])  [unwired: 15 in]
        n301 = call "4155C Write array to file.vi"("Byte Stream File Refnum"=w1147, "Header"=w1143, "Data Array"=w1144, "error in (no error)"=w1148) -> ("dup refnum"=w1145:refnum<file>, "error out"=w1146:errorcluster)  [unwired: 1 in]
        n302 = Close File(refnum=w1145, error in=w1146) -> (error out=w1131:errorcluster)  [unwired: 1 out]
      }
      frame "itime" {
        n303 = Delete From Array(array=w1162, index=1) -> (deleted portion=w1161:string)  [unwired: 1 in, 1 out]
        n304 = Delete From Array(array=w1162, index=0 ("Index")) -> (deleted portion=w1196:string)  [unwired: 1 in, 1 out]
        n305 = Fract/Exp String To Number(string=w1161) -> (number=w1160:dbl)  [unwired: 3 in, 1 out]
        n306 = case shown="\"l\"" w1196 {
          tunnel: w1195 -> [w1201 w1203 w1207]
          tunnel: [w1200 w1202 w1206] -> w1188
          tunnel: w1160 -> [w1198 _ w1205]
          frame "s" {
            w1199 = u32 0 items=["short  ", "medium  ", "long  "] ("integration time 2")
            n307 = Bundle By Name(cluster=w1201, "integration time"=w1199, "Short/Long integration time"=w1198) -> (w1200:T5)
          }
          frame "m", Default {
            w1204 = u32 1 items=["short  ", "medium  ", "long  "] ("integration time 2")
            n308 = Bundle By Name(cluster=w1203, "integration time"=w1204) -> (w1202:T5)
          }
          frame "l" {
            w1208 = u32 2 items=["short  ", "medium  ", "long  "] ("integration time 2")
            n309 = Bundle By Name(cluster=w1207, "integration time"=w1208, "Short/Long integration time"=w1205) -> (w1206:T5)
          }
        }
      }
      frame "pulsed" {
        n310 = Delete From Array(array=w1247, index=0 ("Index")) -> (deleted portion=w1248:string, array with subset deleted=w1235:string[])  [unwired: 1 in]
        n311 = case shown="\"on\", Default" w1248 {
          tunnel: w1246 -> [w1258 w1261]
          tunnel: [w1257 w1260] -> w1239
          tunnel: w1235 -> [w1255 _]
          frame "on", Default {
            w1256 = u16 1 items=["Continuous", "Pulsed"] ("sweep method")
            n312 = Fract/Exp String To Number(string=w1255) -> (number=w1253:dbl[])  [unwired: 3 in, 1 out]
            n313 = Index Array(array=w1253, index #1=0 ("Index")) -> (element #1=w1252:dbl, element #2=w1251:dbl, element #3=w1250:dbl)  [unwired: 2 in]
            n314 = Bundle By Name(cluster=w1258, "sweep method"=w1256, "Pulse period"=w1252, "Base voltage"=w1251, "Pulse width"=w1250) -> (w1257:T5)
          }
          frame "off" {
            w1259 = u16 0 items=["Continuous", "Pulsed"] ("sweep method")
            n315 = Bundle By Name(cluster=w1261, "sweep method"=w1259) -> (w1260:T5)
          }
        }
      }
      frame "gaterangemode" {
        n316 = Delete From Array(array=w1298, index=0 ("Index")) -> (deleted portion=w1299:string)  [unwired: 1 in, 1 out]
        n317 = case shown="\"f\"" w1299 {
          tunnel: [w1301 w1302 w1303] -> w1288
          frame "a", Default {
            w1301 = u16 0 items=["Auto", "Limited", "Fixed"] ("Gate Range\nmode 2")
          }
          frame "f" {
            w1302 = u16 2 items=["Auto", "Limited", "Fixed"] ("Gate Range\nmode 2")
          }
          frame "l" {
            w1303 = u16 1 items=["Auto", "Limited", "Fixed"] ("Gate Range\nmode 2")
          }
        }
      }
      frame "gaterange" {
        (unwired) u8 11 items=["10fA  ", "100fA  ", "1nA  ", "10nA", "100nA", "1uA", "10uA", "100uA", "1mA", "10mA", "100mA", "1A"] ("Gate Range 2")
        n318 = Delete From Array(array=w1347, index=0 ("Index")) -> (deleted portion=w1337:string)  [unwired: 1 in, 1 out]
        n319 = Scan Value(string=w1337, format string="") -> (value=w1335:dbl)  [unwired: 1 in, 1 out]
        n320 = Logarithm Base 10(1:w1335) -> (0:w1334:dbl)
        n321 = Round To Nearest(number=w1334) -> (nearest integer value=w1333:dbl)
        n322 = Add(x=w1333, y=11.0) -> (x+y=w1331:dbl)
        n323 = To Unsigned Byte Integer(number=w1331) -> (unsigned 8bit integer=w1330:u8)
      }
      frame "drainrange" {
        (unwired) u8 11 items=["10fA  ", "100fA  ", "1nA  ", "10nA", "100nA", "1uA", "10uA", "100uA", "1mA", "10mA", "100mA", "1A"] ("Gate Range 2")
        n324 = Delete From Array(array=w1392, index=0 ("Index")) -> (deleted portion=w1383:string)  [unwired: 1 in, 1 out]
        n325 = Scan Value(string=w1383, format string="") -> (value=w1381:dbl)  [unwired: 1 in, 1 out]
        n326 = Logarithm Base 10(1:w1381) -> (0:w1380:dbl)
        n327 = Round To Nearest(number=w1380) -> (nearest integer value=w1379:dbl)
        n328 = Add(x=w1379, y=11.0) -> (x+y=w1377:dbl)
        n329 = To Unsigned Byte Integer(number=w1377) -> (unsigned 8bit integer=w1376:u8)
      }
      frame "drainrangemode" {
        n330 = Delete From Array(array=w1430, index=0 ("Index")) -> (deleted portion=w1431:string)  [unwired: 1 in, 1 out]
        n331 = case shown="\"f\"" w1431 {
          tunnel: [w1433 w1434 w1435] -> w1420
          frame "a", Default {
            w1433 = u16 0 items=["Auto", "Limited", "Fixed"] ("Gate Range\nmode 2")
          }
          frame "f" {
            w1434 = u16 2 items=["Auto", "Limited", "Fixed"] ("Gate Range\nmode 2")
          }
          frame "l" {
            w1435 = u16 1 items=["Auto", "Limited", "Fixed"] ("Gate Range\nmode 2")
          }
        }
      }
      frame "Error", Default {
      }
      frame "logfile" {
        n332 = Number To Decimal String(number=w1498) -> (decimal integer string=w1533:string)  [unwired: 1 in]
        n333 = Concatenate Strings(w1532, "logfile" ("Substring"), w1533, w1496, ".txt" ("Substring")) -> (w1530:string)
        n334 = String To Path(string=w1530) -> (path=w1503:path)
        n335 = Unbundle(w1529) -> ("integration time"=w1528:u32, "Short/Long integration time"=w1527:dbl, "hold time (sec)"=w1526:dbl, "delay time (sec)"=w1525:dbl, "Step Time (0 disables)"=w1524:dbl, "sweep method"=w1523:u16, "Pulse period"=w1522:dbl, "Base voltage"=w1521:dbl, "Pulse width"=w1520:dbl)
        n336 = Build Array(w1528, w1527, w1526, w1525, w1524, w1523, w1522, w1521, w1520, w1514, w1515, w1516, w1517, w1518, w1519) -> (w1507:dbl[])
        n337 = Insert Into Array(array=dbl[][] [] ("Input Array"), new element=w1507) -> (w1506:dbl[][])  [unwired: 2 in]
        n338 = call <vilib>:"compatOverwrite.vi"("overwrite (F)"=TRUE) -> ("overwrite?"=w1501:T8)
        n339 = Open/Create/Replace File(file path (use dialog)=w1503, error in=w1505, operation (0:open)=w1501) -> (refnum out=w1511:refnum<file>, error out=w1510:errorcluster)  [unwired: 3 in, 1 out]
        n340 = call "4155C Write array to file.vi"("Byte Stream File Refnum"=w1511, "Header"=string[] ["Int Time", "Short/Long Itime", "Hold time", "Delay time", "Step time", "Sweep method", "Pulse period", "Base Voltage", "Pulse width", "Drain compliance", "Gate compliance", "Gate range mode", "Gate range", "S/D range mode", "S/D range"], "Data Array"=w1506, "error in (no error)"=w1510) -> ("dup refnum"=w1513:refnum<file>, "error out"=w1512:errorcluster)  [unwired: 1 in]
        n341 = Close File(refnum=w1513, error in=w1512) -> (error out=w1504:errorcluster)  [unwired: 1 out]
      }
      frame "sample" {
        w1569 = 1
        # "The suffix is Vg_Vd_Time."
        # "Add a time offset (elapsed time) to the time axis."
        # "Adjusts graph colors."
        n342 = Number To Decimal String(number=w1603) -> (decimal integer string=w1641:string)  [unwired: 1 in]
        n343 = local read "Sample - Drain"() -> (w1535:u32)
        n344 = Fract/Exp String To Number(string=w1639) -> (number=w1607:dbl[])  [unwired: 3 in, 1 out]
        n345 = Index Array(array=w1607, index=0 ("Index")) -> (element=w1559:dbl)
        n346 = Index Array(array=w1607, index=2 ("Index")) -> (element=w1635:dbl)
        n347 = Index Array(array=w1607, index=3 ("Index")) -> (element=w1556:dbl)
        n348 = Index Array(array=w1607, index=4 ("Index")) -> (element=w1606:dbl)
        n349 = Index Array(array=w1607, index=1 ("Index")) -> (element=w1561:dbl)
        n350 = local read "Sample - Probe 4"() -> (w1538:u32)
        n351 = local read "Sample - Source/Common"() -> (w1536:u32)
        n352 = local read "Plot sample extrema vs time"() -> (w1571:bool)
        n353 = Number To Decimal String(number=w1561) -> (decimal integer string=w1562:string)  [unwired: 1 in]
        n354 = Number To Decimal String(number=w1559) -> (decimal integer string=w1558:string)  [unwired: 1 in]
        n355 = Number To Decimal String(number=w1556) -> (decimal integer string=w1555:string)  [unwired: 1 in]
        n356 = local read "Sample - Gate"() -> (w1537:u32)
        n357 = call "4155C Config Sampling Measurements v2.0.vi"("VISA session"=w1644, "Num Points"=w1635, "Sample - Drain"=w1535, "Display on/off"=TRUE, "Gate Compliance"=w1622, "Sampling interval"=w1606, "Sample - Source/Common"=w1536, "Sample - Probe 4"=w1538, "Drain Compliance"=w1642, "Standby"=w1539, "error in (no error)"=w1643, "Timings"=w1614, "Sample - Gate"=w1537, "Sample time"=w1556) -> ("dup VISA resource name"=w1646:refnum<visa-resource-name>, "error out"=w1645:errorcluster)
        n358 = call "4155C Take Sample v2.0.vi"("VISA resource name in"=w1646, "Emergency Stop"=w1619, "Sample - Gate"=w1537, "Vg"=w1559, "Sample - Drain"=w1535, "Vd"=w1561, "error in (no error)"=w1645) -> ("Time"=w1567:dbl[], "VISA Resource Name out"=w1616:refnum<visa-resource-name>, "Ig"=w1549:dbl[], "Id"=w1550:dbl[], "Is"=w1551:dbl[], "error out"=w1579:errorcluster)  [unwired: 3 in]
        n359 = Insert Into Array(array=w1543, new element=w1550) -> (w1546:dbl[])  [unwired: 1 in]
        n360 = Insert Into Array(array=w1542, new element=w1551) -> (w1548:dbl[])  [unwired: 1 in]
        n361 = Insert Into Array(array=w1544, new element=w1549) -> (w1547:dbl[])  [unwired: 1 in]
        n362 = Add(x=w1567, y=w1563) -> (x+y=w1552:dbl[])
        n363 = Concatenate Strings(w1562, "_" ("Substring"), w1558, "_" ("Substring"), w1555, ".txt" ("Substring")) -> (w1553:string)
        n364 = Concatenate Strings(w1565, w1564, w1641, w1601, "_S_" ("Substring"), w1553) -> (w1640:string)
        n365 = String To Path(string=w1640) -> (path=w1625:path)
        n366 = Insert Into Array(array=w1541, new element=w1552) -> (w1545:dbl[])  [unwired: 1 in]
        n367 = case shown="True" w1571 {
          tunnel: w1552 -> [_ w1649]
          tunnel: [w1647 w1650] -> w1568
          tunnel: w1572 -> [w1647 w1648]
          frame False {
          }
          frame True {
            n368 = Insert Into Array(array=w1648, new element=w1649) -> (w1650:i32[])  [unwired: 1 in]
          }
        }
        n369 = case shown="True" "Plot sample extrema vs time" {
          tunnel: w1551 -> [_ w1679]
          tunnel: w1550 -> [_ w1680]
          tunnel: w1549 -> [_ w1681]
          tunnel: [w1657 w1667] -> w1540
          tunnel: w1579 -> [w1657 w1672]
          tunnel: w1585 -> [w1656 w1684]
          tunnel: w1584 -> [w1655 w1683]
          tunnel: w1583 -> [w1654 w1685]
          tunnel: w1582 -> [w1653 w1682]
          tunnel: w1581 -> [w1652 w1687]
          tunnel: w1580 -> [w1651 w1686]
          tunnel: [w1656 w1671] -> w1578
          tunnel: [w1655 w1665] -> w1577
          tunnel: [w1654 w1669] -> w1576
          tunnel: [w1653 w1664] -> w1575
          tunnel: [w1652 w1670] -> w1574
          tunnel: [w1651 w1663] -> w1573
          tunnel: w1568 -> [_ w1661]
          frame False {
          }
          frame True {
            w1666 = 1
            # "Number of VAR2 steps is 1."
            # "abs(Ig)"
            # "abs(Is)"
            # "abs(Id)"
            # "Adjusts graph colors."
            n370 = Absolute Value(x=w1681) -> (abs(x)=w1658:dbl[])
            n371 = Absolute Value(x=w1680) -> (abs(x)=w1659:dbl[])
            n372 = Absolute Value(x=w1679) -> (abs(x)=w1660:dbl[])
            n373 = Array Max & Min(array=w1660) -> (max value=w1678:dbl, min value=w1675:dbl)  [unwired: 2 out]
            n374 = Array Max & Min(array=w1659) -> (max value=w1677:dbl, min value=w1674:dbl)  [unwired: 2 out]
            n375 = Array Max & Min(array=w1658) -> (max value=w1676:dbl, min value=w1673:dbl)  [unwired: 2 out]
            n376 = local write "Id max"(w1677) -> ()
            n377 = local write "Id min"(w1674) -> ()
            n378 = local write "Ig max"(w1676) -> ()
            n379 = local write "Ig min"(w1673) -> ()
            n380 = Insert Into Array(array=w1687, new element=w1658) -> (w1670:dbl[])  [unwired: 1 in]
            n381 = Insert Into Array(array=w1686, new element=w1658) -> (w1663:dbl[])  [unwired: 1 in]
            n382 = local write "Is max"(w1678) -> ()
            n383 = local write "Is min"(w1675) -> ()
            n384 = Insert Into Array(array=w1685, new element=w1659) -> (w1669:dbl[])  [unwired: 1 in]
            n385 = Insert Into Array(array=w1682, new element=w1659) -> (w1664:dbl[])  [unwired: 1 in]
            n386 = Insert Into Array(array=w1684, new element=w1660) -> (w1671:dbl[])  [unwired: 1 in]
            n387 = Insert Into Array(array=w1683, new element=w1660) -> (w1665:dbl[])  [unwired: 1 in]
            n388 = control-ref of="Imax vs time"() -> (w1688:refnum<vi>)
            n389 = call "4155C Config Chart Colours.vi"("Numeric"=w1666, "XY Graph 2"=w1688) -> ()  [unwired: 6 in]
            n390 = call "4155C Split array.vi"("Number of VAR2 steps"=w1666, "Y2 data in"=w1669, "X data in"=w1661, "Y1 data in"=w1671, "Y3 data in"=w1670, "error in (no error)"=w1672) -> ("Array of clusters"=w1689:cluster{"Y data in":dbl[], "X data in":dbl[]}[], "error out"=w1668:errorcluster)  [unwired: 1 in]
            n391 = call "4155C Split array.vi"("Number of VAR2 steps"=w1666, "Y2 data in"=w1664, "X data in"=w1661, "Y1 data in"=w1665, "Y3 data in"=w1663, "error in (no error)"=w1668) -> ("Array of clusters"=w1662:cluster{"Y data in":dbl[], "X data in":dbl[]}[], "error out"=w1667:errorcluster)  [unwired: 1 in]
            n392 = local write "Imax vs time"(w1689) -> ()
            n393 = local write "Imin vs time"(w1662) -> ()
          }
        }
        n394 = control-ref of="I vs time (Bias Stress)"() -> (w1566:refnum<vi>)
        n395 = call "4155C Split array.vi"("Number of VAR2 steps"=w1569, "Y2 data in"=w1546, "X data in"=w1545, "Y1 data in"=w1548, "Y3 data in"=w1547) -> ("Array of clusters"=w1570:cluster{"Y data in":dbl[], "X data in":dbl[]}[])  [unwired: 2 in, 1 out]
        n396 = local write "I vs time (Bias Stress)"(w1570) -> ()
        n397 = call "4155C Config Chart Colours.vi"("Numeric"=w1569, "XY Graph 2"=w1566) -> ()  [unwired: 6 in]
        n398 = Insert Into Array(array=dbl[][] [] ("Input Array"), new element=w1552) -> (w1629:dbl[][])  [unwired: 2 in]
        n399 = Insert Into Array(array=w1629, new element=w1549) -> (w1628:dbl[][])  [unwired: 2 in]
        n400 = VISA Write(VISA resource name=w1616, write buffer=":DISP ON" ("write buffer (\"\")"), error in (no error)=w1540) -> (VISA resource name out=w1615:refnum<visa-resource-name>, error out=w1617:errorcluster)  [unwired: 1 out]
        n401 = Insert Into Array(array=w1628, new element=w1550) -> (w1627:dbl[][])  [unwired: 2 in]
        n402 = Insert Into Array(array=w1627, new element=w1551) -> (w1621:dbl[][])  [unwired: 2 in]
        n403 = call <vilib>:"compatOverwrite.vi"("overwrite (F)"=TRUE) -> ("overwrite?"=w1604:T8)
        n404 = Open/Create/Replace File(file path (use dialog)=w1625, error in=w1617, operation (0:open)=w1604) -> (refnum out=w1632:refnum<file>, error out=w1631:errorcluster)  [unwired: 3 in, 1 out]
        n405 = Transpose 2D Array(2D array=w1621) -> (transposed array=w1620:dbl[][])
        n406 = call "4155C Write array to file.vi"("Byte Stream File Refnum"=w1632, "Header"=string[] ["Time /s", "Ig /A", "Id /A", "Is /A"], "Data Array"=w1620, "error in (no error)"=w1631) -> ("dup refnum"=w1634:refnum<file>, "error out"=w1633:errorcluster)  [unwired: 1 in]
        n407 = Close File(refnum=w1634, error in=w1633) -> (error out=w1623:errorcluster)  [unwired: 1 out]
      }
      frame "samplei" {
        n408 = Number To Decimal String(number=w1721) -> (decimal integer string=w1772:string)  [unwired: 1 in]
        n409 = local read "Sample I - Source/Common"() -> (w1690:u32)
        n410 = local read "Sample I - Probe 4 (Disabled)"() -> (w1693:u32)
        n411 = Concatenate Strings(w1751, "-samplei-" ("Substring"), w1772, w1720, ".txt" ("Substring")) -> (w1770:string)
        n412 = Fract/Exp String To Number(string=w1769) -> (number=w1736:dbl[])  [unwired: 3 in, 1 out]
        n413 = String To Path(string=w1770) -> (path=w1754:path)
        n414 = Index Array(array=w1736, index=4 ("Index")) -> (element=w1730:dbl)
        n415 = Index Array(array=w1736, index=3 ("Index")) -> (element=w1731:dbl)
        n416 = Index Array(array=w1736, index=1 ("Index")) -> (element=w1733:dbl)
        n417 = Index Array(array=w1736, index=0 ("Index")) -> (element=w1734:dbl)
        n418 = local read "Sample I - Drain/Gate"() -> (w1692:u32)
        n419 = Index Array(array=w1736, index=2 ("Index")) -> (element=w1732:dbl)
        n420 = local read "Sample I - Probe 3 (Disabled)"() -> (w1691:u32)
        n421 = call "4155C Config SamplingI Measurements v2.0.vi"("VISA session"=w1775, "Num Points"=w1733, "Sample I - Probe 3 (Disabled)"=w1691, "Display on/off"=TRUE, "Sample I - Source/Common"=w1690, "Sample I - Drain/Gate"=w1692, "Sampling interval"=w1731, "Standby"=w1694, "error in (no error)"=w1774, "Timings"=w1743, "Sample I - Probe 4 (Disabled)"=w1693, "Sample time"=w1732) -> ("dup VISA resource name"=w1777:refnum<visa-resource-name>, "error out"=w1776:errorcluster)  [unwired: 2 in]
        n422 = call "4155C Take SampleI v2.0.vi"("Sample I - Drain/Gate"=w1692, "Emergency Stop"=w1748, "error in (no error)"=w1776, "Idg 2"=w1734, "Vdg compliance 2"=w1730, "VISA resource name in"=w1777) -> ("error out"=w1746:errorcluster, "Idg"=w1779:dbl[], "Vdg"=w1756:dbl[], "VISA Resource Name out"=w1744:refnum<visa-resource-name>, "Is"=w1778:dbl[], "Time"=w1760:dbl[])
        n423 = Insert Into Array(array=dbl[][] [] ("Input Array"), new element=w1760) -> (w1759:dbl[][])  [unwired: 2 in]
        n424 = Insert Into Array(array=w1759, new element=w1756) -> (w1758:dbl[][])  [unwired: 2 in]
        n425 = Insert Into Array(array=w1758, new element=w1779) -> (w1757:dbl[][])  [unwired: 2 in]
        n426 = VISA Write(VISA resource name=w1744, write buffer=":DISP ON" ("write buffer (\"\")"), error in (no error)=w1746) -> (VISA resource name out=w1729:refnum<visa-resource-name>, error out=w1745:errorcluster)  [unwired: 1 out]
        n427 = Insert Into Array(array=w1757, new element=w1778) -> (w1750:dbl[][])  [unwired: 2 in]
        n428 = call <vilib>:"compatOverwrite.vi"("overwrite (F)"=TRUE) -> ("overwrite?"=w1724:T8)
        n429 = Open/Create/Replace File(file path (use dialog)=w1754, error in=w1745, operation (0:open)=w1724) -> (refnum out=w1763:refnum<file>, error out=w1762:errorcluster)  [unwired: 3 in, 1 out]
        n430 = Transpose 2D Array(2D array=w1750) -> (transposed array=w1749:dbl[][])
        n431 = call "4155C Write array to file.vi"("Byte Stream File Refnum"=w1763, "Header"=string[] ["Time /s", "Vdg /V", "Idg /A", "Is /A"], "Data Array"=w1749, "error in (no error)"=w1762) -> ("dup refnum"=w1765:refnum<file>, "error out"=w1764:errorcluster)  [unwired: 1 in]
        n432 = Close File(refnum=w1765, error in=w1764) -> (error out=w1727:errorcluster)  [unwired: 1 out]
        n433 = VISA Write(VISA resource name=w1729, write buffer=";:PAGE:SCON:STAN OFF;:PAGE:CHAN:VSU2:DIS;" ("write buffer (\"\")"), error in (no error)=w1727) -> (VISA resource name out=w1725:refnum<visa-resource-name>, error out=w1726:errorcluster)  [unwired: 1 out]
      }
      frame "#" {
        n434 = VISA Write(VISA resource name=w1810, write buffer=":DISP ON" ("write buffer (\"\")"), error in (no error)=w1809) -> (VISA resource name out=w1808:refnum<visa-resource-name>, error out=w1807:errorcluster)  [unwired: 1 out]
      }
      frame "stressV" {
        n435 = Number To Decimal String(number=w1847) -> (decimal integer string=w1888:string)  [unwired: 1 in]
        n436 = Concatenate Strings(w1872, "-stressV-" ("Substring"), w1888, w1846, ".txt" ("Substring")) -> (w1886:string)
        n437 = Fract/Exp String To Number(string=w1885) -> (number=w1858:dbl[])  [unwired: 3 in, 1 out]
        n438 = local read "Stress V - Source/Common"() -> (w1821:u32)
        n439 = String To Path(string=w1886) -> (path=w1876:path)
        n440 = Index Array(array=w1858, index=3 ("Index")) -> (element=w1855:dbl)
        n441 = Index Array(array=w1858, index=1 ("Index")) -> (element=w1853:dbl)
        n442 = Index Array(array=w1858, index=0 ("Index")) -> (element=w1852:dbl)
        n443 = Index Array(array=w1858, index=4 ("Index")) -> (element=w1857:dbl)
        n444 = Index Array(array=w1858, index=2 ("Index")) -> (element=w1854:dbl)
        n445 = local read "Stress V - Drain"() -> (w1820:u32)
        n446 = local read "Stress V - Gate"() -> (w1819:u32)
        n447 = call "4155C Config V Stress v2.0.vi"("Display on/off"=TRUE, "Stress V - Gate"=w1819, "Stress V - Drain"=w1820, "Stress V - Source/Common"=w1821, "IG compliance"=w1854, "ID compliance"=w1855, "error in (no error)"=w1890, "VG"=w1852, "VD"=w1853, "VISA session"=w1891) -> ("error out"=w1892:errorcluster, "dup VISA resource name"=w1893:refnum<visa-resource-name>)
        n448 = call "4155C Apply Stress.vi"("error in (no error)"=w1892, "Duration"=w1857, "Emergency Stop"=w1871, "VISA resource name in"=w1893) -> ("error out"=w1869:errorcluster, "VISA Resource Name out"=w1867:refnum<visa-resource-name>)
        n449 = VISA Write(VISA resource name=w1867, write buffer=":DISP ON" ("write buffer (\"\")"), error in (no error)=w1869) -> (VISA resource name out=w1866:refnum<visa-resource-name>, error out=w1868:errorcluster)  [unwired: 1 out]
        n450 = call <vilib>:"compatOverwrite.vi"("overwrite (F)"=TRUE) -> ("overwrite?"=w1851:T8)
        n451 = Open/Create/Replace File(file path (use dialog)=w1876, error in=w1868, operation (0:open)=w1851) -> (refnum out=w1879:refnum<file>, error out=w1878:errorcluster)  [unwired: 3 in, 1 out]
        n452 = call "4155C Write array to file.vi"("Byte Stream File Refnum"=w1879, "Header"=string[] ["V stress completed successfully", ""], "error in (no error)"=w1878) -> ("dup refnum"=w1881:refnum<file>, "error out"=w1880:errorcluster)  [unwired: 2 in]
        n453 = Close File(refnum=w1881, error in=w1880) -> (error out=w1874:errorcluster)  [unwired: 1 out]
      }
      frame "stressI" {
        n454 = local read "Stress I - Source/Common"() -> (w1894:u32)
        n455 = Number To Decimal String(number=w1921) -> (decimal integer string=w1958:string)  [unwired: 1 in]
        n456 = Concatenate Strings(w1942, "-stressI-" ("Substring"), w1958, w1920, ".txt" ("Substring")) -> (w1956:string)
        n457 = Fract/Exp String To Number(string=w1955) -> (number=w1930:dbl[])  [unwired: 3 in, 1 out]
        n458 = Index Array(array=w1930, index=1 ("Index")) -> (element=w1926:dbl)
        n459 = Index Array(array=w1930, index=0 ("Index")) -> (element=w1927:dbl)
        n460 = Index Array(array=w1930, index=2 ("Index")) -> (element=w1928:dbl)
        n461 = String To Path(string=w1956) -> (path=w1946:path)
        n462 = local read "Stress I - Drain/Gate"() -> (w1895:u32)
        n463 = call "4155C Config I Stress v2.0.vi"("Stress I - Drain/Gate"=w1895, "Stress I - Source/Common"=w1894, "Display on/off"=TRUE, "error in (no error)"=w1960, "VDG compliance"=w1926, "IDG"=w1927, "VISA session"=w1961) -> ("error out"=w1962:errorcluster, "dup VISA resource name"=w1963:refnum<visa-resource-name>)  [unwired: 1 in]
        n464 = call "4155C Apply Stress.vi"("error in (no error)"=w1962, "Duration"=w1928, "Emergency Stop"=w1941, "VISA resource name in"=w1963) -> ("error out"=w1939:errorcluster, "VISA Resource Name out"=w1937:refnum<visa-resource-name>)
        n465 = VISA Write(VISA resource name=w1937, write buffer=":DISP ON" ("write buffer (\"\")"), error in (no error)=w1939) -> (VISA resource name out=w1936:refnum<visa-resource-name>, error out=w1938:errorcluster)  [unwired: 1 out]
        n466 = call <vilib>:"compatOverwrite.vi"("overwrite (F)"=TRUE) -> ("overwrite?"=w1925:T8)
        n467 = Open/Create/Replace File(file path (use dialog)=w1946, error in=w1938, operation (0:open)=w1925) -> (refnum out=w1949:refnum<file>, error out=w1948:errorcluster)  [unwired: 3 in, 1 out]
        n468 = call "4155C Write array to file.vi"("Byte Stream File Refnum"=w1949, "Header"=string[] ["I stress completed successfully", ""], "error in (no error)"=w1948) -> ("dup refnum"=w1951:refnum<file>, "error out"=w1950:errorcluster)  [unwired: 2 in]
        n469 = Close File(refnum=w1951, error in=w1950) -> (error out=w1944:errorcluster)  [unwired: 1 out]
      }
      frame "vsu2pulse" {
        n470 = Number To Decimal String(number=w1990) -> (decimal integer string=w2025:string)  [unwired: 1 in]
        n471 = Concatenate Strings(w2010, "-vsu2-" ("Substring"), w2025, w1989, ".txt" ("Substring")) -> (w2023:string)
        n472 = Fract/Exp String To Number(string=w2022) -> (number=w1998:dbl[])  [unwired: 3 in, 1 out]
        n473 = String To Path(string=w2023) -> (path=w2014:path)
        n474 = Index Array(array=w1998, index=1 ("Index")) -> (element=w1997:dbl)
        n475 = Index Array(array=w1998, index=0 ("Index")) -> (element=w1995:dbl)
        n476 = local read "VSU2 Stress - Source/Common"() -> (w1964:u32)
        n477 = call "4155C Config VSU2 Stress v2.0.vi"("VISA session"=w2028, "Display on/off"=TRUE, "VSU2"=w1995, "error in (no error)"=w2027, "VSU2 Stress - Source/Common"=w1964) -> ("dup VISA resource name"=w2030:refnum<visa-resource-name>, "error out"=w2029:errorcluster)
        n478 = call "4155C Apply Stress.vi"("error in (no error)"=w2029, "Duration"=w1997, "Emergency Stop"=w2009, "VISA resource name in"=w2030) -> ("error out"=w2007:errorcluster, "VISA Resource Name out"=w2005:refnum<visa-resource-name>)
        n479 = VISA Write(VISA resource name=w2005, write buffer=":DISP ON" ("write buffer (\"\")"), error in (no error)=w2007) -> (VISA resource name out=w2004:refnum<visa-resource-name>, error out=w2006:errorcluster)  [unwired: 1 out]
        n480 = call <vilib>:"compatOverwrite.vi"("overwrite (F)"=TRUE) -> ("overwrite?"=w1994:T8)
        n481 = Open/Create/Replace File(file path (use dialog)=w2014, error in=w2006, operation (0:open)=w1994) -> (refnum out=w2017:refnum<file>, error out=w2016:errorcluster)  [unwired: 3 in, 1 out]
        n482 = call "4155C Write array to file.vi"("Byte Stream File Refnum"=w2017, "Header"=string[] ["VSU2 pulse completed successfully", ""], "error in (no error)"=w2016) -> ("dup refnum"=w2019:refnum<file>, "error out"=w2018:errorcluster)  [unwired: 2 in]
        n483 = Close File(refnum=w2019, error in=w2018) -> (error out=w2012:errorcluster)  [unwired: 1 out]
      }
      frame "sample-fpp" {
        w2072 = string[] ["Time /s", "Id VgVd /A", "Ig VgVd /A", "Vp1 VgVd /V", "Vp2 VgVd /V"] ("Header")
        w2076 = "%d" ("format string")
        n484 = Number To Decimal String(number=w2062) -> (decimal integer string=w2124:string)  [unwired: 1 in]
        n485 = Fract/Exp String To Number(string=w2121) -> (number=w2109:dbl[])  [unwired: 3 in, 1 out]
        n486 = Concatenate Strings(w2115, "-samplefpp-" ("Substring"), w2124, w2061, ".txt" ("Substring")) -> (w2122:string)
        n487 = local read "FPP - Source"() -> (w2031:u32)
        n488 = local read "FPP - Drain"() -> (w2032:u32)
        n489 = local read "FPP - Gate"() -> (w2033:u32)
        n490 = local read "FPP - Probe 1"() -> (w2034:u32)
        n491 = String To Path(string=w2122) -> (path=w2084:path)
        n492 = Index Array(array=w2109, index=0 ("Index")) -> (element=w2071:dbl)
        n493 = Index Array(array=w2109, index=1 ("Index")) -> (element=w2070:dbl)
        n494 = Index Array(array=w2109, index=2 ("Index")) -> (element=w2117:dbl)
        n495 = Index Array(array=w2109, index=3 ("Index")) -> (element=w2107:dbl)
        n496 = Number To Decimal String(number=w2071) -> (decimal integer string=w2096:string)  [unwired: 1 in]
        n497 = local read "FPP - Probe 2"() -> (w2035:u32)
        n498 = call "4155C Config Sampling Measurements FPP v2.0.vi"("VISA session"=w2127, "Gate Compliance"=w2116, "FPP - Source"=w2031, "FPP - Drain"=w2032, "Drain Compliance"=w2125, "error in (no error)"=w2126, "Num Points"=w2117, "Timings"=w2114, "FPP - Gate"=w2033, "FPP - Probe 1"=w2034, "Vg"=w2071, "Vd"=w2070, "Display on/off"=TRUE, "Sample time"=w2107, "FPP - Probe 2"=w2035, "Standby"=w2036) -> ("dup VISA resource name"=w2086:refnum<visa-resource-name>, "error out"=w2085:errorcluster)  [unwired: 2 in]
        n499 = call "4155C Take Sample FPP.vi"("VISA resource name in"=w2086, "error in (no error)"=w2085, "Emergency Stop"=w2087) -> ("Time"=w2091:dbl[], "Vp1"=w2101:dbl[], "VISA Resource Name out"=w2068:refnum<visa-resource-name>, "Ig"=w2089:dbl[], "Id"=w2090:dbl[], "Vp2"=w2099:dbl[], "error out"=w2088:errorcluster)  [unwired: 10 in]
        n500 = Insert Into Array(array=dbl[][] [] ("Input Array"), new element=w2091) -> (w2105:dbl[][])  [unwired: 2 in]
        n501 = Number To Decimal String(number=w2070) -> (decimal integer string=w2094:string)  [unwired: 1 in]
        n502 = Insert Into Array(array=w2105, new element=w2090) -> (w2104:dbl[][])  [unwired: 2 in]
        n503 = Concatenate Strings("(Vg = " ("Substring"), w2096, "V, Vd = " ("Substring"), w2094, "V)" ("Substring")) -> (w2092:string)
        n504 = Insert Into Array(array=w2104, new element=w2089) -> (w2103:dbl[][])  [unwired: 2 in]
        n505 = Insert Into Array(array=w2103, new element=w2101) -> (w2100:dbl[][])  [unwired: 2 in]
        n506 = Insert Into Array(array=w2100, new element=w2099) -> (w2069:dbl[][])  [unwired: 2 in]
        n507 = Transpose 2D Array(2D array=w2069) -> (transposed array=w2098:dbl[][])
        n508 = call <vilib>:"compatOverwrite.vi"("overwrite (F)"=TRUE) -> ("overwrite?"=w2066:T8)
        n509 = Open/Create/Replace File(file path (use dialog)=w2084, error in=w2088, operation (0:open)=w2066) -> (refnum out=w2081:refnum<file>, error out=w2082:errorcluster)  [unwired: 3 in, 1 out]
        n510 = Array To Spreadsheet String(array=w2072, 3:w2076) -> (spreadsheet string=w2078:string)  [unwired: 1 in]
        n511 = Search and Replace String(replace all?=TRUE ("replace all? (F)"), input string=w2078, search string="VgVd", replace string=w2092) -> (result string=w2074:string)  [unwired: 4 in, 3 out]
        n512 = Spreadsheet String To Array(format string=w2076, spreadsheet string=w2074, array type (2D Dbl)=w2072) -> (array=w2073:string[])  [unwired: 1 in]
        n513 = call "4155C Write array to file.vi"("Byte Stream File Refnum"=w2081, "Header"=w2073, "Data Array"=w2098, "error in (no error)"=w2082) -> ("dup refnum"=w2079:refnum<file>, "error out"=w2080:errorcluster)  [unwired: 1 in]
        n514 = Close File(refnum=w2079, error in=w2080) -> (error out=w2067:errorcluster)  [unwired: 1 out]
      }
      frame "resample-fpp" {
        w2166 = string[] ["Time /s", "Id VgVd /A", "Ig VgVd /A", "Vp1 VgVd /V", "Vp2 VgVd /V"] ("Header")
        w2170 = "%d" ("format string")
        n515 = Number To Decimal String(number=w2152) -> (decimal integer string=w2210:string)  [unwired: 1 in]
        n516 = Fract/Exp String To Number(string=w2207) -> (number=w2159:dbl[])  [unwired: 3 in, 1 out]
        n517 = Concatenate Strings(w2203, "-resamplefpp-" ("Substring"), w2210, w2153, ".txt" ("Substring")) -> (w2208:string)
        n518 = String To Path(string=w2208) -> (path=w2178:path)
        n519 = Index Array(array=w2159, index=0 ("Index")) -> (element=w2165:dbl)
        n520 = Index Array(array=w2159, index=1 ("Index")) -> (element=w2164:dbl)
        n521 = Number To Decimal String(number=w2165) -> (decimal integer string=w2188:string)  [unwired: 1 in]
        n522 = call "4155C Take Sample FPP.vi"("VISA resource name in"=w2161, "error in (no error)"=w2160, "Emergency Stop"=w2179) -> ("Time"=w2183:dbl[], "Vp1"=w2193:dbl[], "VISA Resource Name out"=w2163:refnum<visa-resource-name>, "Ig"=w2181:dbl[], "Id"=w2182:dbl[], "Vp2"=w2191:dbl[], "error out"=w2180:errorcluster)  [unwired: 10 in]
        n523 = Insert Into Array(array=dbl[][] [] ("Input Array"), new element=w2183) -> (w2197:dbl[][])  [unwired: 2 in]
        n524 = Number To Decimal String(number=w2164) -> (decimal integer string=w2186:string)  [unwired: 1 in]
        n525 = Insert Into Array(array=w2197, new element=w2182) -> (w2196:dbl[][])  [unwired: 2 in]
        n526 = Concatenate Strings("(Vg = " ("Substring"), w2188, "V, Vd = " ("Substring"), w2186, "V)" ("Substring")) -> (w2184:string)
        n527 = Insert Into Array(array=w2196, new element=w2181) -> (w2195:dbl[][])  [unwired: 2 in]
        n528 = Insert Into Array(array=w2195, new element=w2193) -> (w2192:dbl[][])  [unwired: 2 in]
        n529 = Insert Into Array(array=w2192, new element=w2191) -> (w2158:dbl[][])  [unwired: 2 in]
        n530 = call <vilib>:"compatOverwrite.vi"("overwrite (F)"=TRUE) -> ("overwrite?"=w2157:T8)
        n531 = Open/Create/Replace File(file path (use dialog)=w2178, error in=w2180, operation (0:open)=w2157) -> (refnum out=w2175:refnum<file>, error out=w2176:errorcluster)  [unwired: 3 in, 1 out]
        n532 = Array To Spreadsheet String(array=w2166, 3:w2170) -> (spreadsheet string=w2172:string)  [unwired: 1 in]
        n533 = Transpose 2D Array(2D array=w2158) -> (transposed array=w2190:dbl[][])
        n534 = Search and Replace String(replace all?=TRUE ("replace all? (F)"), input string=w2172, search string="VgVd", replace string=w2184) -> (result string=w2168:string)  [unwired: 4 in, 3 out]
        n535 = Spreadsheet String To Array(format string=w2170, spreadsheet string=w2168, array type (2D Dbl)=w2166) -> (array=w2167:string[])  [unwired: 1 in]
        n536 = call "4155C Write array to file.vi"("Byte Stream File Refnum"=w2175, "Header"=w2167, "Data Array"=w2190, "error in (no error)"=w2176) -> ("dup refnum"=w2173:refnum<file>, "error out"=w2174:errorcluster)  [unwired: 1 in]
        n537 = Close File(refnum=w2173, error in=w2174) -> (error out=w2162:errorcluster)  [unwired: 1 out]
      }
      frame "serial" {
        n538 = local read "Termination char\n(0xA = '\\n' = LF)\n(0xD = '\\r' = CR)"() -> (w2243:u8)
        n539 = local read "Enable Termination\nChar (T)"() -> (w2244:bool)
        n540 = Index Array(array=w2251, index=0 ("Index")) -> (element=w2250:string)
        n541 = local read "parity"() -> (w2234:u16)
        n542 = local read "Delay before read (ms)"() -> (w2245:u32)
        n543 = local read "byte count"() -> (w2242:u32)
        n544 = local read "Timeout (ms)"() -> (w2241:u32)
        n545 = local read "VISA resource name"() -> (w2238:refnum<visa-resource-name>)
        n546 = local read "baud rate"() -> (w2237:u32)
        n547 = local read "Serial End Mode for Reads"() -> (w2236:u16)
        n548 = local read "data bits"() -> (w2235:u16)
        n549 = local read "stop bits"() -> (w2240:u16)
        n550 = local read "flow control"() -> (w2239:u16)
        n551 = call "Serial write and read v0.5.vi"("Delay before read (ms)"=w2245, "Termination char\n(0xA = '\\n' = LF)\n(0xD = '\\r' = CR)"=w2243, "Enable Termination\nChar (T)"=w2244, "parity"=w2234, "stop bits"=w2240, "string to write"=w2250, "flow control"=w2239, "byte count"=w2242, "Serial Settings:Serial End Mode for Reads"=w2236, "Timeout (ms)"=w2241, "error in (no error)"=w2256, "VISA resource name"=w2238, "baud rate"=w2237, "data bits"=w2235) -> ("Serial port output"=w2246:string, "error out"=w2255:errorcluster)
        n552 = Build Array (concatenate)(w2246, w2247) -> (w2248:string[])
      }
      frame "pump" {
        # "Time array for valve position"
        # "Time array for absolute plunger position"
        # "Valve position"
        # "Absolute plunger position"
        # "Remove \"_\""
        # "Check if hard stop is pressed."
        # "Check if halt is pressed."
        # "Check if pump is idle. Else halt."
        n553 = Index Array(array=w2326, index=0 ("Index")) -> (element=w2303:string)
        n554 = case shown="\"No error\", Default" w2301 {
          tunnel: w2303 -> [w2362 _ w2364 w2365 w2366 w2367 _ _ w2370 w2371 _]
          tunnel: [w2362 "/1H" w2364 w2365 w2366 w2367 "/1H" "/1H" w2370 w2371 "/1H"] -> w2302
          frame "No error", Default {
          }
          frame "Initialization" {
          }
          frame "Invalid command" {
          }
          frame "Invalid operand" {
          }
          frame "Device not initialized" {
          }
          frame "Internal failure" {
          }
          frame "Plunger overload" {
          }
          frame "Valve overload" {
          }
          frame "Plunger move not allowed" {
          }
          frame "A/D converter failure" {
          }
          frame "Command overflow" {
          }
        }
        n555 = local read "Hard stop pump"() -> (w2305:bool)
        n556 = local read "Halt pump"() -> (w2308:bool)
        n557 = local read "Serial End Mode for Reads"() -> (w2314:u16)
        n558 = local read "flow control"() -> (w2317:u16)
        n559 = local read "stop bits"() -> (w2318:u16)
        n560 = local read "parity"() -> (w2312:u16)
        n561 = local read "Delay before read (ms)"() -> (w2323:u32)
        n562 = local read "byte count"() -> (w2320:u32)
        n563 = local read "Timeout (ms)"() -> (w2319:u32)
        n564 = local read "VISA resource name"() -> (w2316:refnum<visa-resource-name>)
        n565 = local read "baud rate"() -> (w2315:u32)
        n566 = local read "Enable Termination\nChar (T)"() -> (w2322:bool)
        n567 = local read "Termination char\n(0xA = '\\n' = LF)\n(0xD = '\\r' = CR)"() -> (w2321:u8)
        n568 = case shown="True" w2308 {
          tunnel: [w2376 "/1H"] -> w2307
          tunnel: w2302 -> [w2376 _]
          frame False {
          }
          frame True {
            n569 = local write "Halt pump"(FALSE) -> ()
          }
        }
        n570 = case shown="True" w2305 {
          tunnel: [w2373 "/1T"] -> w2306
          tunnel: w2307 -> [w2373 _]
          frame False {
          }
          frame True {
            n571 = local write "Hard stop pump"(FALSE) -> ()
          }
        }
        n572 = local read "data bits"() -> (w2313:u16)
        n573 = String Subset(string=w2297, offset (0)=1) -> (substring=w2295:string)  [unwired: 1 in]
        n574 = call "SPM Pump v0.6.vi"("Termination char\n(0xA = '\\n' = LF)\n(0xD = '\\r' = CR)"=w2321, "Enable Termination\nChar (T)"=w2322, "Timeout (ms)"=w2319, "Serial Settings:Serial End Mode for Reads"=w2314, "byte count"=w2320, "Delay before read (ms)"=w2323, "Time <input>"=w2300, "error in (no error)"=w2331, "Serial port input"=w2306, "VISA resource name"=w2316, "parity"=w2312, "baud rate"=w2315, "stop bits"=w2318, "data bits"=w2313, "flow control"=w2317, "Time units <input>"=w2295) -> ("Input command"=w2294:string, "Serial port data"=w2284:string[], "Pump status"=w2290:string, "Valve position"=w2292:i32, "Absolute plunger position"=w2304:i32, "Serial port"=w2299:string, "error out"=w2330:errorcluster)  [unwired: 1 in, 4 out]
        n575 = case shown="\"?6\"" w2294 {
          tunnel: [w2343 w2351 w2357] -> w2311
          tunnel: w2310 -> [w2343 w2350 w2357]
          tunnel: w2304 -> [_ w2349 _]
          tunnel: w2291 -> [w2342 w2348 w2358]
          tunnel: [w2342 w2348 w2360] -> w2293
          tunnel: w2292 -> [_ _ w2359]
          tunnel: w2289 -> [_ w2347 w2355]
          tunnel: w2288 -> [w2341 w2346 w2356]
          tunnel: [w2341 w2345 w2356] -> w2287
          tunnel: [w2340 w2344 w2354] -> w2286
          tunnel: w2285 -> [w2340 w2344 w2353]
          frame "Q", Default {
          }
          frame "?" {
            n576 = Build Array (concatenate)(w2350, w2349) -> (w2351:i32[])
            n577 = Build Array (concatenate)(w2346, w2347) -> (w2345:i32[])
            n578 = call "4155C Split array.vi"("X data in"=w2345, "Y1 data in"=w2351) -> ("Array of clusters"=w2352:cluster{"Y data in":dbl[], "X data in":dbl[]}[])  [unwired: 5 in, 1 out]
            n579 = local write "Absolute plunger position vs time"(w2352) -> ()
          }
          frame "?6" {
            n580 = Build Array (concatenate)(w2358, w2359) -> (w2360:i32[])
            n581 = Build Array (concatenate)(w2353, w2355) -> (w2354:i32[])
            n582 = call "4155C Split array.vi"("X data in"=w2354, "Y1 data in"=w2360) -> ("Array of clusters"=w2361:cluster{"Y data in":dbl[], "X data in":dbl[]}[])  [unwired: 5 in, 1 out]
            n583 = local write "Valve position vs time"(w2361) -> ()
          }
        }
        n584 = Build Array (concatenate)(w2282, w2284) -> (w2283:string[][])
        n585 = Build Array (concatenate)(w2298, w2299) -> (w2324:string[])
      }
      frame "filename" {
        n586 = Index Array(array=w2385, index=0 ("Index")) -> (element=w2384:string)
      }
    }
    n587 = local read "Time Units"() -> (w104:u16)
    n588 = case shown="0" w104 {
      tunnel: ["Time (Seconds)" ("element") "Time (Minutes)" ("element") "Time (Hours)" ("element")] -> w82
      frame 0 {
      }
      frame 1, Default {
      }
      frame 2 {
      }
    }
    n589 = Build Array(w178, w111, w121, w120, w119, w118, w117, w116, w115, w114, w113, w112, w110) -> (w216:dbl[][])
    n590 = Transpose 2D Array(2D array=w216) -> (transposed array=w215:dbl[][])
    n591 = Concatenate Strings(w75, w74, "Imax_Imin_Ion_Ioff_vs_time.txt" ("Suffix (Imax,Imin,Ion,Ioff)")) -> (w226:string)
    n592 = Build Array(w82, "Is max (A)" ("VAR2 Name"), "Is min (A)" ("VAR2 Name"), "Id max (A)" ("VAR2 Name"), "Id min (A)" ("VAR2 Name"), "Ig max (A)" ("VAR2 Name"), "Ig min (A)" ("VAR2 Name"), "Is on (A)" ("VAR2 Name"), "Is off (A)" ("VAR2 Name"), "Id on (A)" ("VAR2 Name"), "Id off (A)" ("VAR2 Name"), "Ig on (A)" ("VAR2 Name"), "Ig off (A)" ("VAR2 Name")) -> (w221:string[])
    n593 = Array To Spreadsheet String(array=w215, 3:"%e" ("format string")) -> (spreadsheet string=w219:string)  [unwired: 1 in]
    n594 = Array To Spreadsheet String(array=w221, 3:"" ("format string")) -> (spreadsheet string=w220:string)  [unwired: 1 in]
    n595 = String To Path(string=w226) -> (path=w225:path)
    n596 = Build Array(w220, w219) -> (w218:string[])
    n597 = Write to Text File(file (use dialog)=w225, text=w218, error in=w175) -> (refnum out=w227:refnum<file>, error out=w217:errorcluster)  [unwired: 1 in, 1 out]
    n598 = Close File(refnum=w227, error in=w217) -> (error out=w159:errorcluster)  [unwired: 1 out]
    n599 = Build Array(w156, w179) -> (w184:i32[][])
    n600 = Build Array(w82, "Absolute plunger position" ("VAR2 Name")) -> (w187:string[])
    n601 = Transpose 2D Array(2D array=w184) -> (transposed array=w177:i32[][])
    n602 = Array To Spreadsheet String(array=w187, 3:"" ("format string")) -> (spreadsheet string=w186:string)  [unwired: 1 in]
    n603 = Array To Spreadsheet String(array=w177, 3:"%e" ("format string")) -> (spreadsheet string=w183:string)  [unwired: 1 in]
    n604 = Build Array(w186, w183) -> (w189:string[])
    n605 = Concatenate Strings(w75, w74, "plunger_vs_time.txt" ("Suffix (plunger)")) -> (w181:string)
    n606 = String To Path(string=w181) -> (path=w180:path)
    n607 = Write to Text File(file (use dialog)=w180, text=w189, error in=w159) -> (refnum out=w182:refnum<file>, error out=w191:errorcluster)  [unwired: 1 in, 1 out]
    n608 = Close File(refnum=w182, error in=w191) -> (error out=w158:errorcluster)  [unwired: 1 out]
    n609 = Concatenate Strings(w75, w74, "serial_port_output.txt" ("Suffix (serial port log)")) -> (w197:string)
    n610 = String To Path(string=w197) -> (path=w196:path)
    n611 = Build Array(w82, "Serial port input" ("VAR2 Name"), "Pump status" ("VAR2 Name"), "Serial port output: ") -> (w146:string[])
    n612 = Array To Spreadsheet String(array=w152, 3:"" ("format string")) -> (spreadsheet string=w143:string)  [unwired: 1 in]
    n613 = Array To Spreadsheet String(array=w146, 3:"" ("format string")) -> (spreadsheet string=w144:string)  [unwired: 1 in]
    n614 = Array To Spreadsheet String(array=w151, 3:"" ("format string")) -> (spreadsheet string=w202:string)  [unwired: 1 in]
    n615 = Build Array(w144, w143) -> (w145:string[])
    n616 = Write to Text File(file (use dialog)=w196, text=w145, error in=w158) -> (refnum out=w198:refnum<file>, error out=w199:errorcluster)  [unwired: 1 in, 1 out]
    n617 = local write "Serial port data"(w202) -> ()
    n618 = Close File(refnum=w198, error in=w199) -> (error out=w157:errorcluster)  [unwired: 1 out]
    n619 = Build Array(w155, w161) -> (w167:i32[][])
    n620 = Build Array(w82, "Valve port" ("VAR2 Name")) -> (w170:string[])
    n621 = Transpose 2D Array(2D array=w167) -> (transposed array=w162:i32[][])
    n622 = Array To Spreadsheet String(array=w170, 3:"" ("format string")) -> (spreadsheet string=w169:string)  [unwired: 1 in]
    n623 = Array To Spreadsheet String(array=w162, 3:"%e" ("format string")) -> (spreadsheet string=w166:string)  [unwired: 1 in]
    n624 = Build Array(w169, w166) -> (w172:string[])
    n625 = Concatenate Strings(w75, w74, "valve_port_vs_time.txt" ("Suffix (valve)")) -> (w164:string)
    n626 = String To Path(string=w164) -> (path=w163:path)
    n627 = Write to Text File(file (use dialog)=w163, text=w172, error in=w157) -> (refnum out=w165:refnum<file>, error out=w174:errorcluster)  [unwired: 1 in, 1 out]
    n628 = Close File(refnum=w165, error in=w174) -> (error out=w77:errorcluster)  [unwired: 1 out]
    n629 = Build Array(w73, w72, w71, w70) -> (w88:dbl[][])
    n630 = Build Array("Time (Seconds)" ("element"), "Is (A)" ("VAR2 Name"), "Id (A)" ("VAR2 Name"), "Ig (A)" ("VAR2 Name")) -> (w84:string[])
    n631 = Transpose 2D Array(2D array=w88) -> (transposed array=w87:dbl[][])
    n632 = Concatenate Strings(w75, w74, "sample_vs_time.txt" ("Suffix (Imax,Imin,Ion,Ioff)")) -> (w94:string)
    n633 = Array To Spreadsheet String(array=w84, 3:"" ("format string")) -> (spreadsheet string=w83:string)  [unwired: 1 in]
    n634 = Array To Spreadsheet String(array=w87, 3:"%e" ("format string")) -> (spreadsheet string=w91:string)  [unwired: 1 in]
    n635 = String To Path(string=w94) -> (path=w93:path)
    n636 = Build Array(w83, w91) -> (w90:string[])
    n637 = Write to Text File(file (use dialog)=w93, text=w90, error in=w77) -> (refnum out=w95:refnum<file>, error out=w89:errorcluster)  [unwired: 1 in, 1 out]
    n638 = Close File(refnum=w95, error in=w89) -> (error out=w76:errorcluster)  [unwired: 1 out]
  }
  "error out" <- w32
  "Timings Indicator" <- w17
  "Probe 4 Indicator" <- w3
  "Is max" <- w15
  "Id max" <- w15
  "Ig max" <- w15
  "Imax vs time" <- w1
  "I vs Vg" <- w1
  "Imin vs time" <- w1
  "I vs Vd" <- w1
  "Serial port data" <- "" ("Serial port data")
  "Valve position vs time" <- cluster{"Y data in":dbl[], "X data in":dbl[]}[] [] ("Valve position vs time")
  "Is min" <- w14
  "Id min" <- w14
  "Ig min" <- w14
  "Ion vs time" <- w1
  "Ioff vs time" <- w1
  "Is on" <- w13
  "Id on" <- w13
  "Ig on" <- w13
  "Is off" <- w12
  "Id off" <- w12
  "Ig off" <- w12
  "I vs time (Bias Stress)" <- w1
